vi "SubB.vi"(0 "Target B-Field":dbl=1.0 min=-4.0 max=4.0 step=0.1 format="%.4f", 3 "Custom Folder":string, 5 "optional Bias (V)":dbl=1e-08) -> ()   [LabVIEW 2013]
uses:
  <vilib>/Utility/file.llb/Write To Spreadsheet File (DBL).vi
panel:
  out "Numeric 5":dbl
  out "Difference":dbl
  out "Number of Points":dbl
  out "Time of measurement Measurement":dbl
  in  "Sweep Rate":dbl
  out "Current B-Field":dbl
  out "Numeric 4":i32
  in  "Commutator":bool
  in  "Commute SorceMeter":enum32{"Radio Selection 1", "Radio Selection 2"}(radio)
  out "Numeric 3":i32
  in  "Channel 2 (Vnano3b)":bool
  in  "Channel 1 (Vnano3)":bool
  out "Numeric":i32
  in  "Capacitance (C) and Loss (L)":bool
  in  "Magnetic Field (B)":bool
  in  "Current (Ik3)":bool
  in  "Voltage (Vk3)":bool
  in  "Current (Ik2)":bool
  in  "Voltage (Vk2)":bool
  in  "Channel 2 (Vnano2b)":bool
  in  "Channel 1 (Vnano2)":bool
  in  "Thermometer 1 (T1)":bool=TRUE
  in  "Channel 2 (Vnano1b)":bool
  in  "Channel 1 (Vnano1)":bool
  in  "Current (Ik1)":bool=TRUE
  in  "Voltage (Vk1)":bool
  out "Numeric Current":dbl
  out "Delib Time delay":i32
  in  "points at each Vg":i32=1
  out "XY Graph":cluster{dbl[], dbl[]}(graph)={[1.0, 0.8, 0.6000000000000001, 0.4000000000000001, 0.20000000000000007, 5.551115123125783e-17, -0.19999999999999996, -0.39999999999999997, -0.6, -0.8, -1.0], [0.03352775, 0.056811, 0.03911575, 0.04330675, -0.02468015, 0.011641600000000002, 0.10151450000000001, 0.12386675000000001, 0.08288825000000001, -0.00186266, -0.038650000000000004]}
  in  "Time btw \npoints, sec":dbl=1.0 format="%.2f"
  out "Array 2":dbl[][](array[numeric])
  out "array for data":dbl[](array[numeric])
  out "Numeric 2":dbl
  out "Array":string[](array[string])
  in  "Addr 1 lock-in oop":bool
  in  "Ring":u16(ring) caption="Y-axis:" items=["Vg"]
  out "String":string
  out "Data file:":path
  in  "error in (no error)":errorcluster
  in  "Ring 3":u16(ring)=1 items=["1 kOhm", "10 kOhm", "100 kOhm", "1 Mohm", "10 mOhm"]
  in  "Ring 2":u16(ring)=3 items=["1 kOhm", "10 kOhm", "100 kOhm", "1 Mohm", "10 mOhm"]
  in  "Fixed Current mkA":dbl=1.0
  in  "Current is:":T1(radio)
  in  "Ressitance measurements?":bool=TRUE
  in  "Addr 5 lock-in oop":bool
  in  "Addr 4 lock-in oop":bool
  in  "Addr 3 lock-in oop":bool
  in  "Addr 2 lock-in oop":bool
  in  "Addr 5 lock-in":bool
  in  "Addr 4 lock-in":bool
  in  "Addr 3 lock-in":bool=TRUE
  in  "Addr 2 lock-in":bool=TRUE
  in  "Addr 1 lock-in":bool=TRUE
  # "Keithley 2400: address 12"
  # "SourceMeters"
  # "Nanovoltmeters"
  # "Temperature"
  # "Main"
  # "Magnetic Field"
  # "(not recommended, too slow)"
  # "Capacitance & Loss"
  # "(not recommended, too slow)"
  # "(not recommended, too slow)"
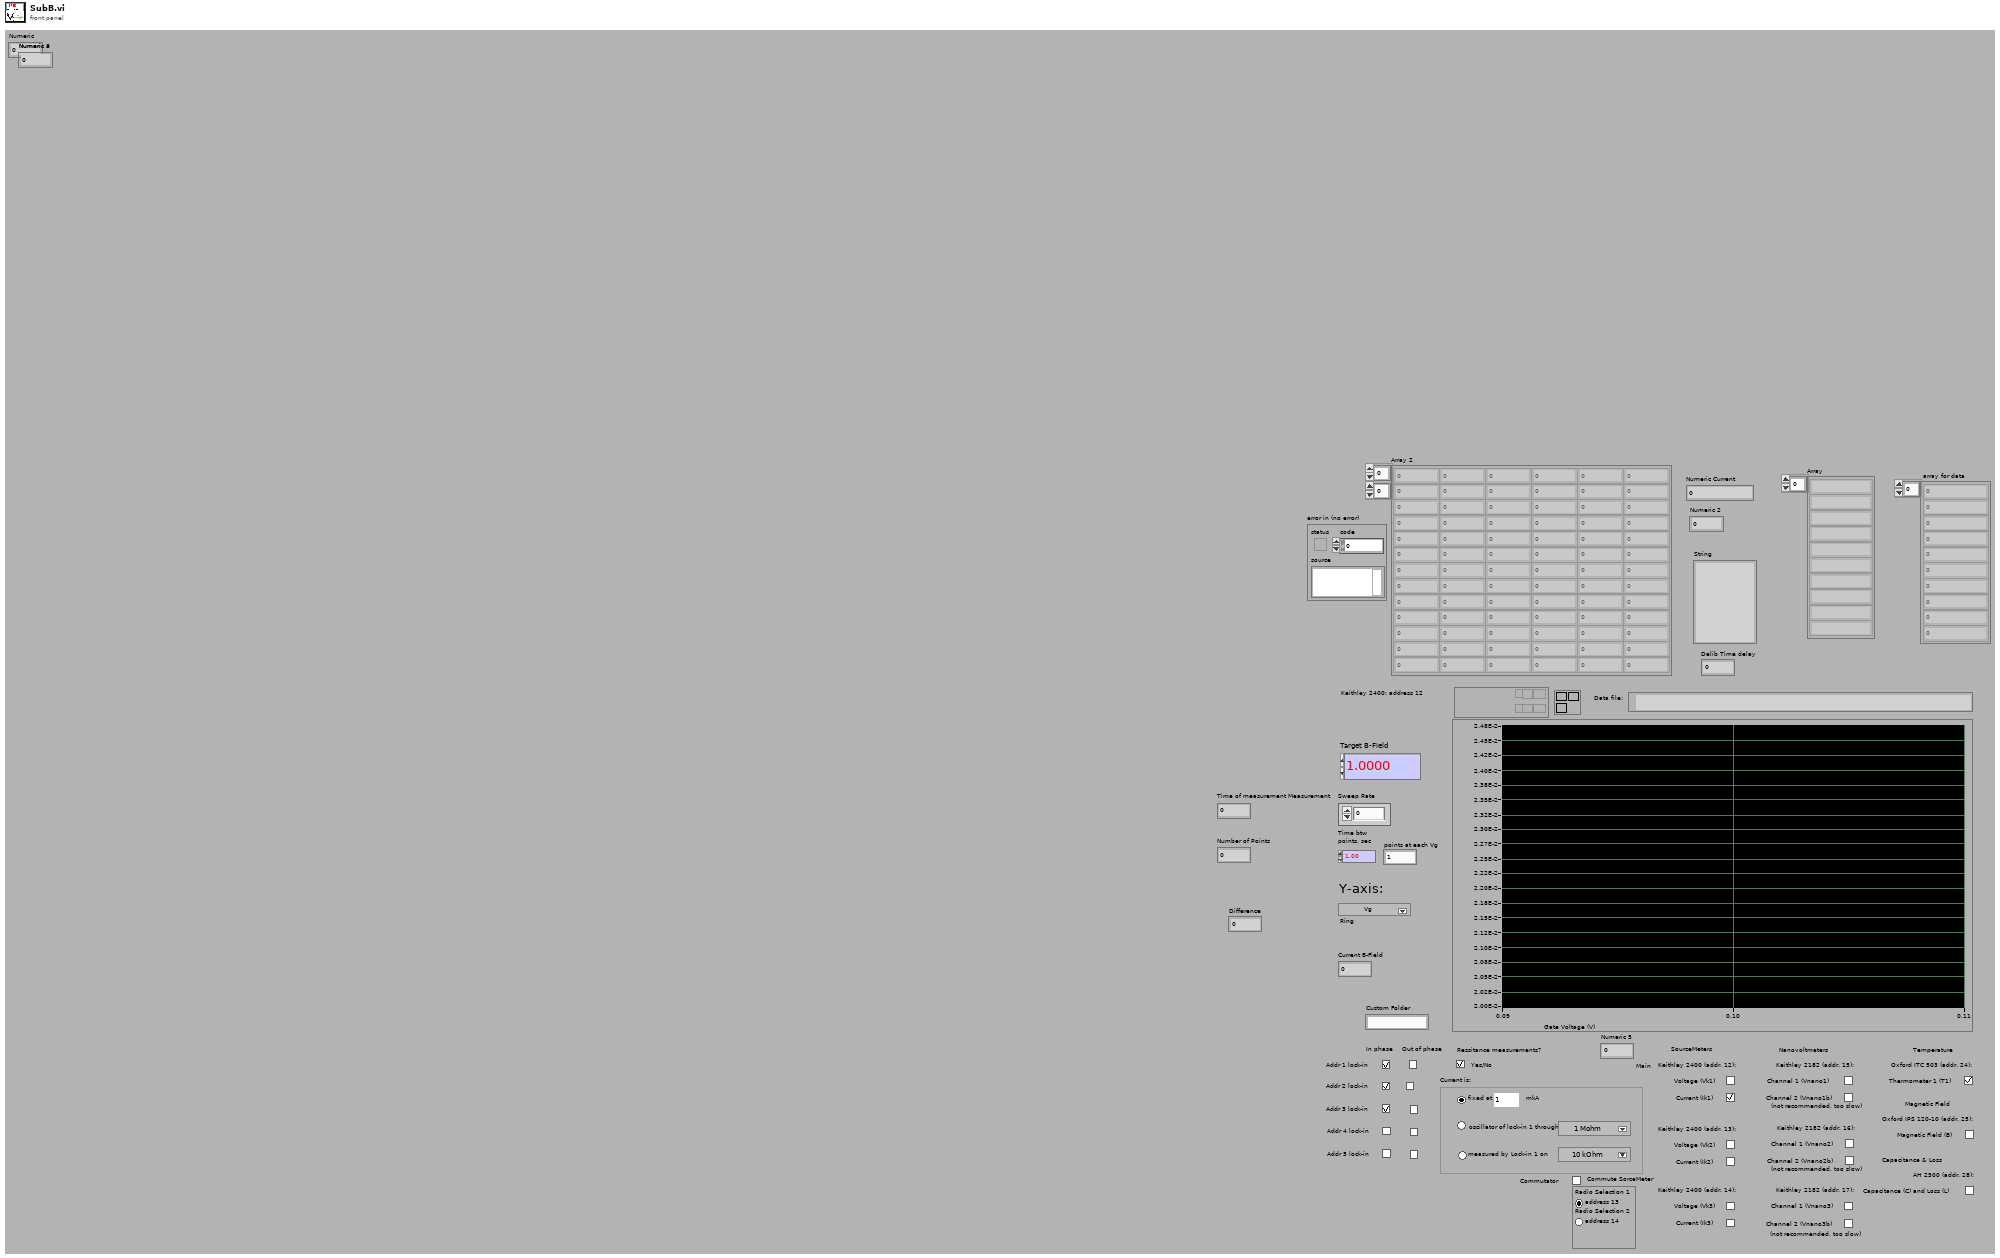
[diagram p1: front panel]
types:
  T1 = enum32{"Radio Selection 1", "Radio Selection 2", "Radio Selection 3"}
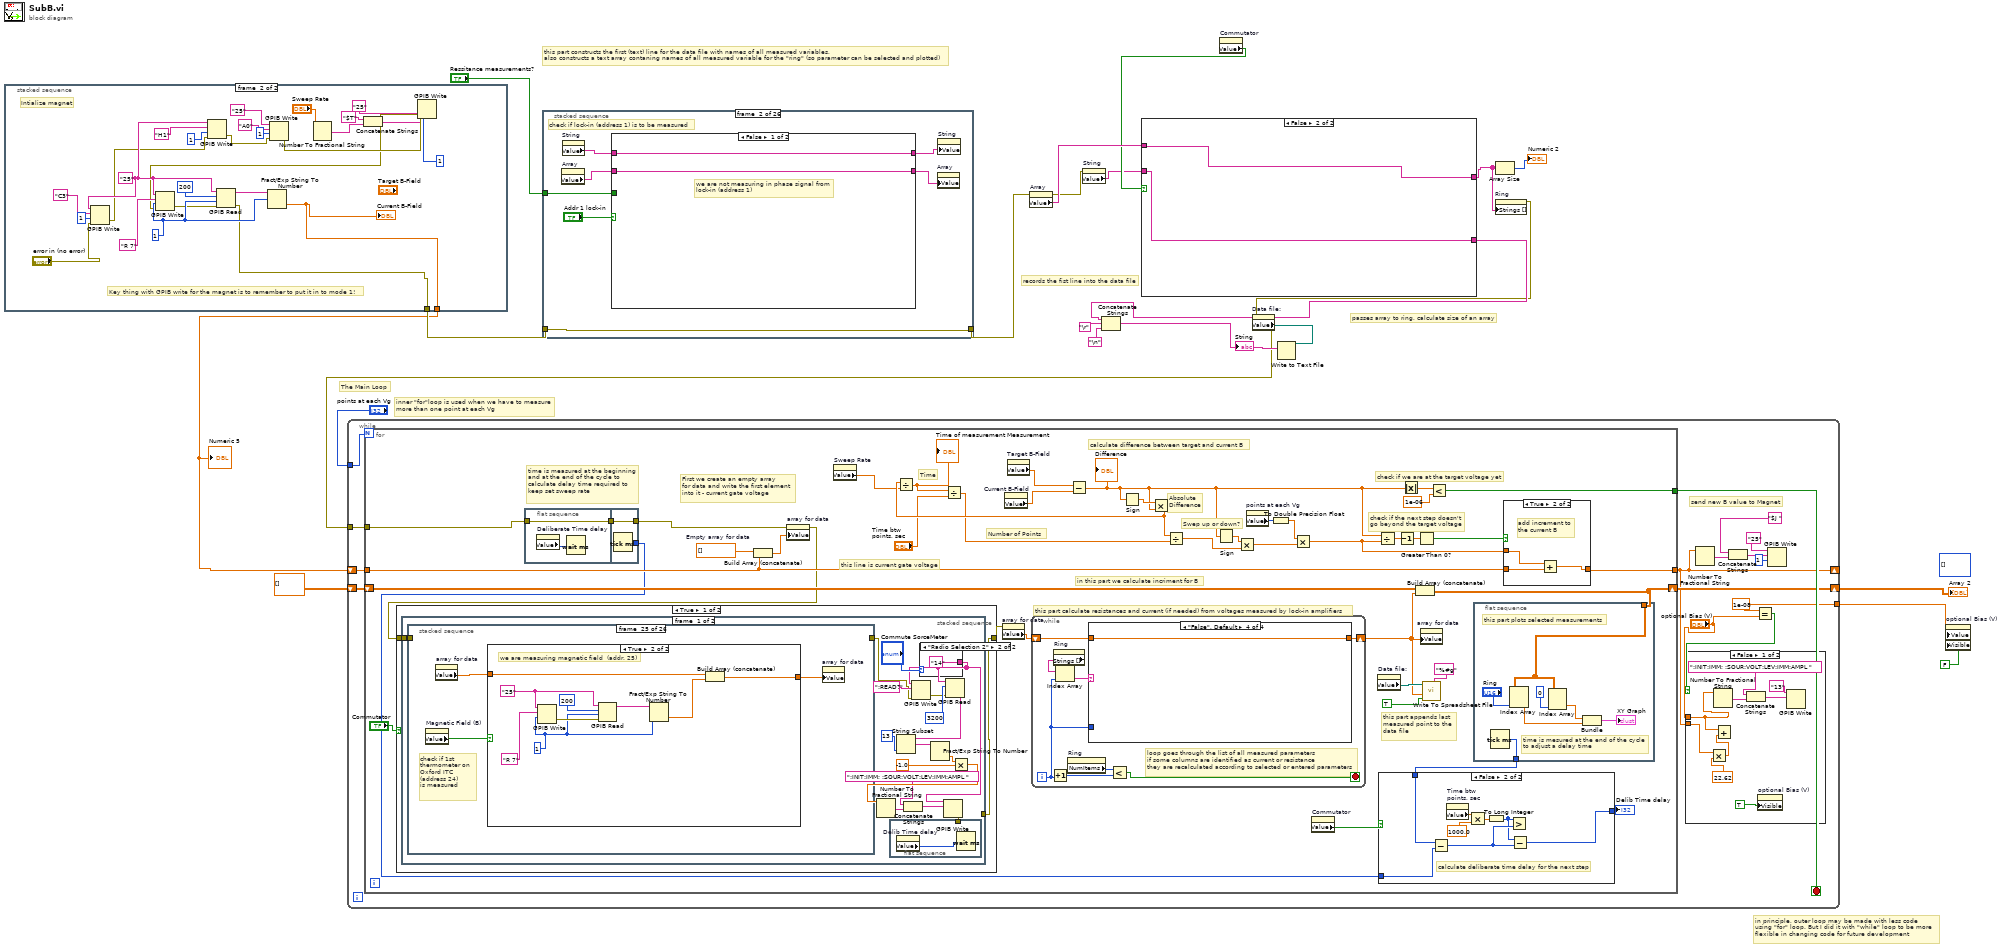
[diagram p0: block diagram]
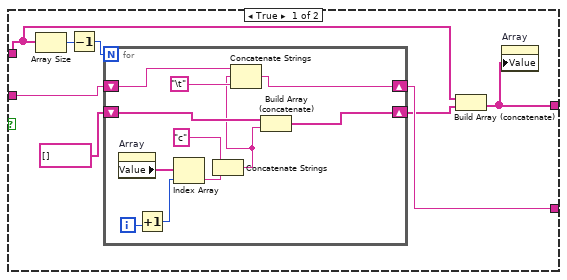
[diagram p2: hidden frame]
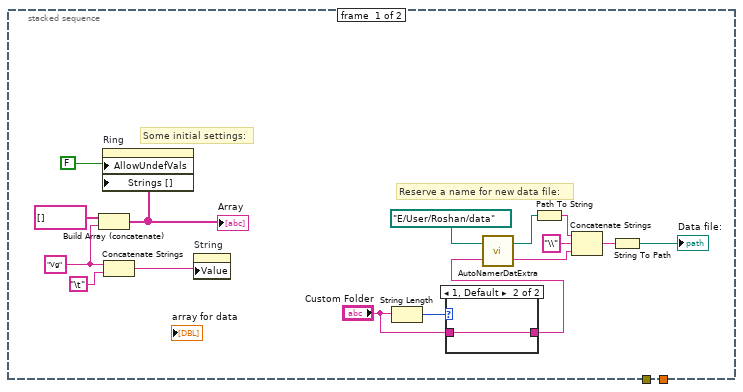
[diagram p3: hidden frame]
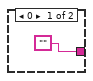
[diagram p4: hidden frame]
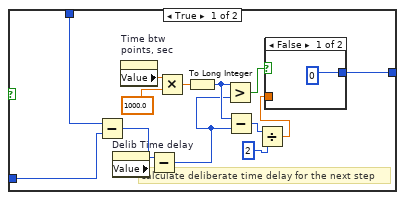
[diagram p6: hidden frame]
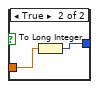
[diagram p7: hidden frame]
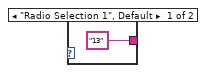
[diagram p8: hidden frame]
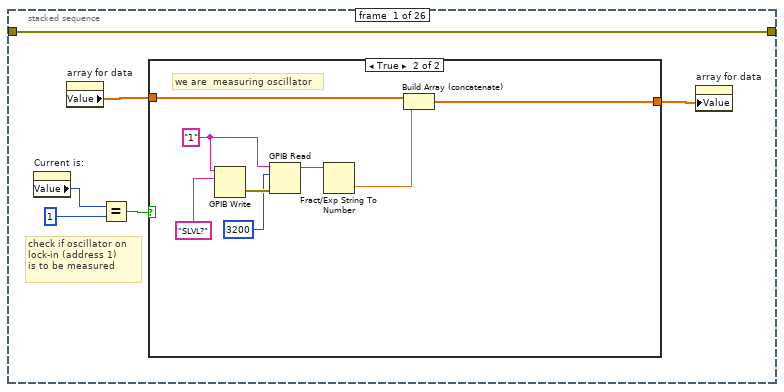
[diagram p9: hidden frame]
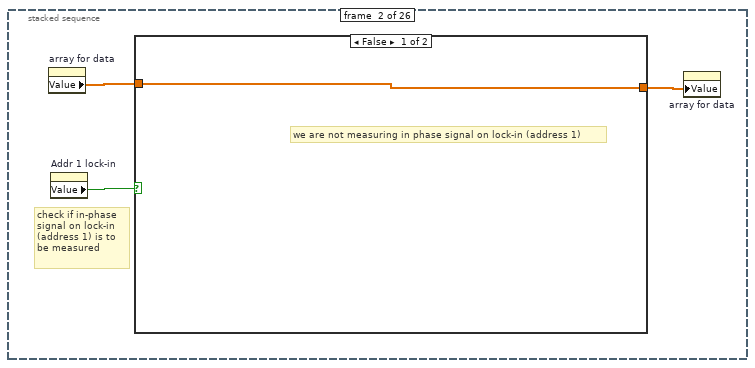
[diagram p11: hidden frame]
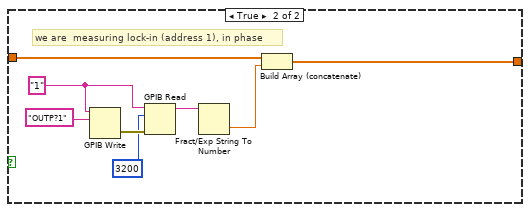
[diagram p12: hidden frame]
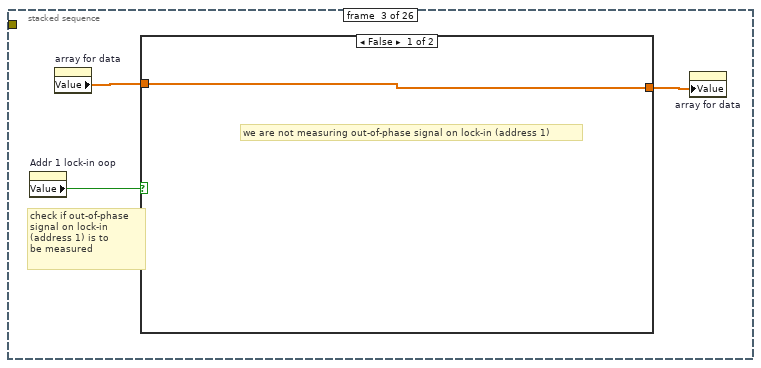
[diagram p13: hidden frame]
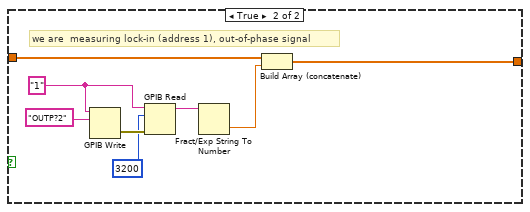
[diagram p14: hidden frame]
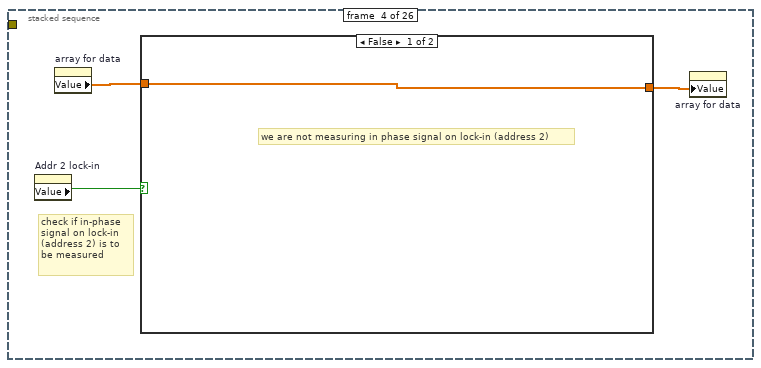
[diagram p15: hidden frame]
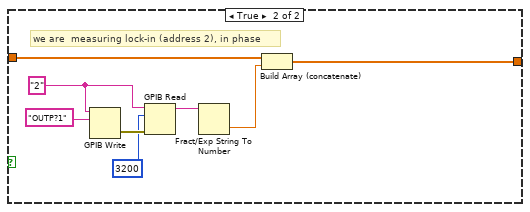
[diagram p16: hidden frame]
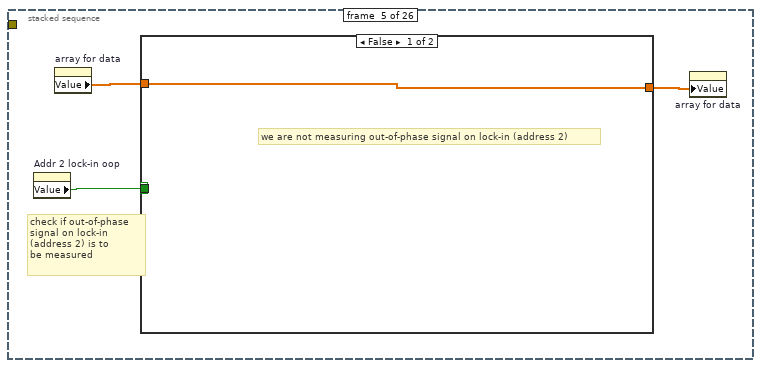
[diagram p17: hidden frame]
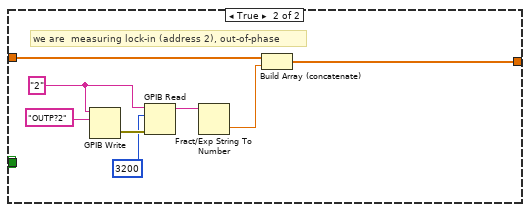
[diagram p18: hidden frame]
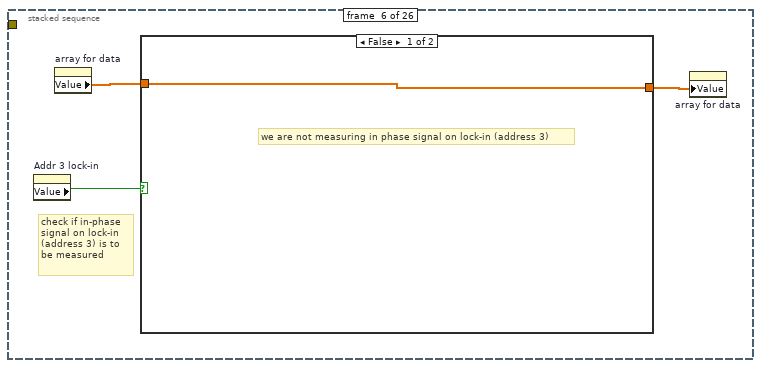
[diagram p19: hidden frame]
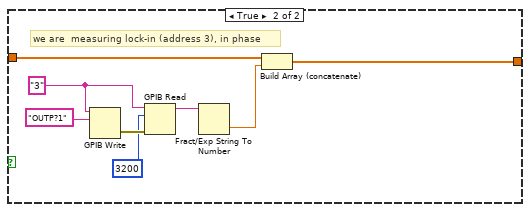
[diagram p20: hidden frame]
diagram:
  (unwired) i32[][] []
  # "passes array to ring, calculate size of an array"
  # "in principle, outer loop may be made with less code\nusing \"for\" loop. But I did it with \"while\" loop to be more \nflexible in changing code for future development"
  # "inner \"for\"loop is used when we have to measure\nmore than one point at each Vg"
  # "The Main Loop"
  # "records the fist line into the data file"
  # "this part constructs the first (text) line for the data file with names of all measured variables,\nalso constructs a text array contaning names of all measured variable for the \"ring\" (so parameter can be selected and plotted)"
  n1 = stacked-sequence {
    tunnel: [_ w61] -> w22
    tunnel: [_ w60] -> w1
    frame #0 {
      w28 = "Vg"
      # "Some initial settings:"
      # "Reserve a name for new data file:"
      n2 = Build Array (concatenate)(string[] [], w28) -> (w30:string[])
      "Array" <- w30
      n3 = property on="Ring" class="Ring (strict)"("AllowUndefVals"=FALSE, "Strings []"=w30) -> ()  [unwired: 2 in, 2 out]
      n4 = Concatenate Strings(w28, "\t") -> (w29:string)
      n5 = property on="String" class="Str"("Value"=w29) -> ()  [unwired: 2 in, 2 out]
      n6 = String Length(string="Custom Folder") -> (length=w25:i32)
      n7 = case shown="1, Default" w25 {
        tunnel: "Custom Folder" -> [_ w40]
        tunnel: ["" w40] -> w23
        frame 0 {
        }
        frame 1, Default {
        }
      }
      n8 = call "AutoNamerDatExtra.vi"("ExtraString"=w23, "Custom User Path"=path "E:/User/Roshan/data") -> ("String"=w38:string, "Path"=w37:path)
      n9 = Path To String(path=w37) -> (string=w32:string)
      n10 = Concatenate Strings(w32, "\\", w38) -> (w34:string)
      n11 = String To Path(string=w34) -> (path=→"Data file:":path)
    }
    frame #1 {
      w66 = 1
      w56 = "25"
      # "Key thing with GPIB write for the magnet is to remember to put it in to mode 1!"
      # "Intialize magnet"
      n12 = GPIB Write(0:w56, 1:"C3" ("data"), 2:i16 1 ("mode (0)"), 3:"error in (no error)") -> (6:w53:errorcluster)  [unwired: 1 in, 1 out]
      n13 = GPIB Write(0:w56, 1:"H1" ("data"), 2:i16 1 ("mode (0)"), 3:w53) -> (6:w49:errorcluster)  [unwired: 1 in, 1 out]
      n14 = GPIB Write(0:"25" ("address string"), 1:"A0" ("data"), 2:i16 1 ("mode (0)"), 3:w49) -> (6:w48:errorcluster)  [unwired: 1 in, 1 out]
      n15 = Number To Fractional String(number="Sweep Rate") -> (F-format string=w44:string)  [unwired: 3 in]
      n16 = Concatenate Strings("$T" ("string"), w44) -> (w42:string)
      n17 = GPIB Write(0:"25" ("address string"), 1:w42, 2:i16 1 ("mode (0)"), 3:w48) -> (6:w47:errorcluster)  [unwired: 1 in, 1 out]
      n18 = GPIB Write(0:w56, 1:"R 7", 2:w66, 3:w47) -> (6:w62:errorcluster)  [unwired: 1 in, 1 out]
      n19 = GPIB Read(0:w56, 1:200, 2:w66, 3:w62) -> (5:w65:string, 7:w61:errorcluster)  [unwired: 1 in, 1 out]
      n20 = Fract/Exp String To Number(string=w65, offset=w66) -> (number=w60:dbl)  [unwired: 2 in, 1 out]
      "Current B-Field" <- w60
    }
  }
  "Numeric 5" <- w1
  n21 = stacked-sequence {
    tunnel: "Ressitance measurements?" -> [w74 w89 w113 w136 w154 w172 w190 w208 w226 w244 w262 _ _ _ _ _ _ _ _ _ _ _ _ _ _ _]
    tunnel: w22 -> [_ w86 _ _ _ _ _ _ _ _ _ _ _ _ _ _ _ _ _ _ _ _ _ _ _ _]
    tunnel: [_ w86 _ _ _ _ _ _ _ _ _ _ _ _ _ _ _ _ _ _ _ _ _ _ _ _] -> w19
    frame #0 {
      # "check if oscillator of  lock-in (address 1) is to be measured"
      n22 = property on="Array" class="Arr (strict)"() -> ("Value"=w69:string[])  [unwired: 2 in, 2 out]
      n23 = property on="String" class="Str"() -> ("Value"=w73:string)  [unwired: 2 in, 2 out]
      n24 = Equal?(x="Current is:", y=1) -> (x = y?=w70:bool)
      n25 = case shown="False" w70 {
        tunnel: w74 -> [_ _]
        tunnel: [w76 w77] -> w72
        tunnel: w73 -> [w76 w80]
        tunnel: w69 -> [w75 w79]
        tunnel: [w75 w78] -> w68
        frame False {
          # "we are not measuring oscillator from\nlock-in (address 1)"
        }
        frame True {
          w81 = "I"
          # "we are  measuring oscillator"
          n26 = GPIB Clear(3:"1") -> ()  [unwired: 1 in, 2 out]
          n27 = Concatenate Strings(w80, w81, "\t") -> (w77:string)
          n28 = Build Array (concatenate)(w79, w81) -> (w78:string[])
        }
      }
      n29 = property on="Array" class="Arr (strict)"("Value"=w68) -> ()  [unwired: 2 in, 2 out]
      n30 = property on="String" class="Str"("Value"=w72) -> ()  [unwired: 2 in, 2 out]
    }
    frame #1 {
      # "check if lock-in (address 1) is to be measured"
      n31 = property on="Array" class="Arr (strict)"() -> ("Value"=w85:string[])  [unwired: 2 in, 2 out]
      n32 = property on="String" class="Str"() -> ("Value"=w88:string)  [unwired: 2 in, 2 out]
      n33 = case shown="False" "Addr 1 lock-in" {
        tunnel: w89 -> [_ w100]
        tunnel: [w92 w96] -> w87
        tunnel: w88 -> [w92 w95]
        tunnel: w85 -> [w91 w97]
        tunnel: [w91 w98] -> w84
        frame False {
          # "we are not measuring in phase signal from\nlock-in (address 1)"
        }
        frame True {
          # "are we measuring resistance?"
          n34 = GPIB Clear(3:"1") -> ()  [unwired: 1 in, 2 out]
          n35 = case shown="True" w100 {
            tunnel: ["V1" w102] -> w93
            frame False {
              # "no, we are not measuring resistanse;\nall lock-ins are measuring voltage"
            }
            frame True {
              # "are we measuring current as well?"
              n36 = property on="Current is:" class="RadioBtnsControl (strict)"() -> ("Value"=w104:T1)  [unwired: 2 in, 2 out]
              n37 = Equal?(x=w104, y=2) -> (x = y?=w105:bool)
              n38 = case shown="False" w105 {
                tunnel: ["R1" "I"] -> w102
                frame False {
                  # "no, we are not \nmeasuring current\nby lock-in \n(address 1); \nso this lock-in is \nmeasuring resistance"
                }
                frame True {
                  # "yes, we are measuring \ncurrent by lock-in \n(address 1) as \nvoltage drop on \nknown resistance"
                }
              }
            }
          }
          n39 = Concatenate Strings(w95, w93, "\t") -> (w96:string)
          n40 = Build Array (concatenate)(w97, w93) -> (w98:string[])
        }
      }
      n41 = property on="Array" class="Arr (strict)"("Value"=w84) -> ()  [unwired: 2 in, 2 out]
      n42 = property on="String" class="Str"("Value"=w87) -> ()  [unwired: 2 in, 2 out]
    }
    frame #2 {
      # "check if out-of-phase signal on  lock-in (address 1) is to be measured"
      n43 = property on="Array" class="Arr (strict)"() -> ("Value"=w110:string[])  [unwired: 2 in, 2 out]
      n44 = property on="String" class="Str"() -> ("Value"=w112:string)  [unwired: 2 in, 2 out]
      n45 = case shown="False" "Addr 1 lock-in oop" {
        tunnel: w113 -> [_ w123]
        tunnel: [w115 w119] -> w111
        tunnel: w112 -> [w115 w118]
        tunnel: w110 -> [w114 w120]
        tunnel: [w114 w121] -> w109
        frame False {
          # "we are not measuring iout-of-phase signal from\nlock-in (address 1)"
        }
        frame True {
          # "are we measuring resistance?"
          n46 = GPIB Clear(3:"1") -> ()  [unwired: 1 in, 2 out]
          n47 = case shown="True" w123 {
            tunnel: ["V1oop" w125] -> w116
            frame False {
              # "no, we are not measuring resistance;\nall lock-ins are measuring voltage"
            }
            frame True {
              # "are we measuring out-of-phase current as well?"
              n48 = property on="Current is:" class="RadioBtnsControl (strict)"() -> ("Value"=w127:T1)  [unwired: 2 in, 2 out]
              n49 = Equal?(x=w127, y=2) -> (x = y?=w128:bool)
              n50 = case shown="False" w128 {
                tunnel: ["R1oop" "Ioop"] -> w125
                frame False {
                  # "no, we are not \nmeasuring current\nby lock-in \n(address 1); so this \nlock-in is measuring\nout-of-phase resistance"
                }
                frame True {
                  # "yes, we are measuring \nout-of phase current \nby lock-in (address 1) \nas voltage drop on \nknown resistance"
                }
              }
            }
          }
          n51 = Concatenate Strings(w118, w116, "\t") -> (w119:string)
          n52 = Build Array (concatenate)(w120, w116) -> (w121:string[])
        }
      }
      n53 = property on="Array" class="Arr (strict)"("Value"=w109) -> ()  [unwired: 2 in, 2 out]
      n54 = property on="String" class="Str"("Value"=w111) -> ()  [unwired: 2 in, 2 out]
    }
    frame #3 {
      # "check if in-phase signal on  lock-in (address 2) is to be measured"
      n55 = property on="Array" class="Arr (strict)"() -> ("Value"=w133:string[])  [unwired: 2 in, 2 out]
      n56 = property on="String" class="Str"() -> ("Value"=w135:string)  [unwired: 2 in, 2 out]
      n57 = case shown="False" "Addr 2 lock-in" {
        tunnel: w136 -> [_ w146]
        tunnel: [w138 w142] -> w134
        tunnel: w135 -> [w138 w141]
        tunnel: w133 -> [w137 w143]
        tunnel: [w137 w144] -> w132
        frame False {
          # "we are not measuring in-phase signal from\nlock-in (address 2)"
        }
        frame True {
          # "are we measuring resistance?"
          n58 = GPIB Clear(3:"2") -> ()  [unwired: 1 in, 2 out]
          n59 = case shown="True" w146 {
            tunnel: ["R2" "V2"] -> w139
            frame True {
              # "we are measuring \nresistance by lock-in \n(address 2)"
            }
            frame False, Default {
              # "no, we are not measuring resistance;\nall lock-ins are measuring voltage"
            }
          }
          n60 = Concatenate Strings(w141, w139, "\t") -> (w142:string)
          n61 = Build Array (concatenate)(w143, w139) -> (w144:string[])
        }
      }
      n62 = property on="Array" class="Arr (strict)"("Value"=w132) -> ()  [unwired: 2 in, 2 out]
      n63 = property on="String" class="Str"("Value"=w134) -> ()  [unwired: 2 in, 2 out]
    }
    frame #4 {
      # "check if out-of-phase signal on  lock-in (address 2) is to be measured"
      n64 = property on="Array" class="Arr (strict)"() -> ("Value"=w151:string[])  [unwired: 2 in, 2 out]
      n65 = property on="String" class="Str"() -> ("Value"=w153:string)  [unwired: 2 in, 2 out]
      n66 = case shown="False" "Addr 2 lock-in oop" {
        tunnel: w154 -> [_ w164]
        tunnel: [w156 w160] -> w152
        tunnel: w153 -> [w156 w159]
        tunnel: w151 -> [w155 w161]
        tunnel: [w155 w162] -> w150
        frame False {
          # "we are not measuring out-of-phase signal from\nlock-in (address 2)"
        }
        frame True {
          # "are we measuring resistance?"
          n67 = GPIB Clear(3:"2") -> ()  [unwired: 1 in, 2 out]
          n68 = case shown="True" w164 {
            tunnel: ["R2oop" "V2oop"] -> w157
            frame True {
              # "we are measuring out-of-phase resistance by lock-in (address 2)\n(address 2)"
            }
            frame False, Default {
              # "no, we are not measuring resistance;\nall lock-ins are measuring voltage"
            }
          }
          n69 = Concatenate Strings(w159, w157, "\t") -> (w160:string)
          n70 = Build Array (concatenate)(w161, w157) -> (w162:string[])
        }
      }
      n71 = property on="Array" class="Arr (strict)"("Value"=w150) -> ()  [unwired: 2 in, 2 out]
      n72 = property on="String" class="Str"("Value"=w152) -> ()  [unwired: 2 in, 2 out]
    }
    frame #5 {
      # "check if in-phase signal on  lock-in (address 3) is to be measured"
      n73 = property on="Array" class="Arr (strict)"() -> ("Value"=w169:string[])  [unwired: 2 in, 2 out]
      n74 = property on="String" class="Str"() -> ("Value"=w171:string)  [unwired: 2 in, 2 out]
      n75 = case shown="False" "Addr 3 lock-in" {
        tunnel: w172 -> [_ w182]
        tunnel: [w174 w178] -> w170
        tunnel: w171 -> [w174 w177]
        tunnel: w169 -> [w173 w179]
        tunnel: [w173 w180] -> w168
        frame False {
          # "we are not measuring in-phase signal from\nlock-in (address 3)"
        }
        frame True {
          # "are we measuring resistance?"
          n76 = GPIB Clear(3:"3") -> ()  [unwired: 1 in, 2 out]
          n77 = case shown="True" w182 {
            tunnel: ["R3" "V3"] -> w175
            frame True {
              # "we are measuring \nresistance by lock-in \n(address 3)"
            }
            frame False, Default {
              # "no, we are not measuring resistance;\nall lock-ins are measuring voltage"
            }
          }
          n78 = Concatenate Strings(w177, w175, "\t") -> (w178:string)
          n79 = Build Array (concatenate)(w179, w175) -> (w180:string[])
        }
      }
      n80 = property on="Array" class="Arr (strict)"("Value"=w168) -> ()  [unwired: 2 in, 2 out]
      n81 = property on="String" class="Str"("Value"=w170) -> ()  [unwired: 2 in, 2 out]
    }
    frame #6 {
      # "check if out-of-phase signal on  lock-in (address 3) is to be measured"
      n82 = property on="Array" class="Arr (strict)"() -> ("Value"=w187:string[])  [unwired: 2 in, 2 out]
      n83 = property on="String" class="Str"() -> ("Value"=w189:string)  [unwired: 2 in, 2 out]
      n84 = case shown="False" "Addr 3 lock-in oop" {
        tunnel: w190 -> [_ w200]
        tunnel: [w192 w196] -> w188
        tunnel: w189 -> [w192 w195]
        tunnel: w187 -> [w191 w197]
        tunnel: [w191 w198] -> w186
        frame False {
          # "we are not measuring out-of-phase signal from\nlock-in (address 3)"
        }
        frame True {
          # "are we measuring resistance?"
          n85 = GPIB Clear(3:"3") -> ()  [unwired: 1 in, 2 out]
          n86 = case shown="True" w200 {
            tunnel: ["R3oop" "V3oop"] -> w193
            frame True {
              # "we are measuring out-of-phase resistance by lock-in (address 3)\n(address 2)"
            }
            frame False, Default {
              # "no, we are not measuring resistance;\nall lock-ins are measuring voltage"
            }
          }
          n87 = Concatenate Strings(w195, w193, "\t") -> (w196:string)
          n88 = Build Array (concatenate)(w197, w193) -> (w198:string[])
        }
      }
      n89 = property on="Array" class="Arr (strict)"("Value"=w186) -> ()  [unwired: 2 in, 2 out]
      n90 = property on="String" class="Str"("Value"=w188) -> ()  [unwired: 2 in, 2 out]
    }
    frame #7 {
      # "check if in-phase signal on  lock-in (address 4) is to be measured"
      n91 = property on="Array" class="Arr (strict)"() -> ("Value"=w205:string[])  [unwired: 2 in, 2 out]
      n92 = property on="String" class="Str"() -> ("Value"=w207:string)  [unwired: 2 in, 2 out]
      n93 = case shown="False" "Addr 4 lock-in" {
        tunnel: w208 -> [_ w218]
        tunnel: [w210 w214] -> w206
        tunnel: w207 -> [w210 w213]
        tunnel: w205 -> [w209 w215]
        tunnel: [w209 w216] -> w204
        frame False {
          # "we are not measuring in-phase signal from\nlock-in (address 4)"
        }
        frame True {
          # "are we measuring resistance?"
          n94 = GPIB Clear(3:"4") -> ()  [unwired: 1 in, 2 out]
          n95 = case shown="True" w218 {
            tunnel: ["R4" "V4"] -> w211
            frame True {
              # "we are measuring \nresistance by lock-in \n(address 4)"
            }
            frame False, Default {
              # "no, we are not measuring resistance;\nall lock-ins are measuring voltage"
            }
          }
          n96 = Concatenate Strings(w213, w211, "\t") -> (w214:string)
          n97 = Build Array (concatenate)(w215, w211) -> (w216:string[])
        }
      }
      n98 = property on="Array" class="Arr (strict)"("Value"=w204) -> ()  [unwired: 2 in, 2 out]
      n99 = property on="String" class="Str"("Value"=w206) -> ()  [unwired: 2 in, 2 out]
    }
    frame #8 {
      # "check if out-of-phase signal on  lock-in (address 4) is to be measured"
      n100 = property on="Array" class="Arr (strict)"() -> ("Value"=w223:string[])  [unwired: 2 in, 2 out]
      n101 = property on="String" class="Str"() -> ("Value"=w225:string)  [unwired: 2 in, 2 out]
      n102 = case shown="False" "Addr 4 lock-in oop" {
        tunnel: w226 -> [_ w236]
        tunnel: [w228 w232] -> w224
        tunnel: w225 -> [w228 w231]
        tunnel: w223 -> [w227 w233]
        tunnel: [w227 w234] -> w222
        frame False {
          # "we are not measuring out-of-phase signal from\nlock-in (address 4)"
        }
        frame True {
          # "are we measuring resistance?"
          n103 = GPIB Clear(3:"4") -> ()  [unwired: 1 in, 2 out]
          n104 = case shown="True" w236 {
            tunnel: ["R4oop" "V4oop"] -> w229
            frame True {
              # "we are measuring out-of-phase resistance by lock-in (address 4)\n(address 2)"
            }
            frame False, Default {
              # "no, we are not measuring resistance;\nall lock-ins are measuring voltage"
            }
          }
          n105 = Concatenate Strings(w231, w229, "\t") -> (w232:string)
          n106 = Build Array (concatenate)(w233, w229) -> (w234:string[])
        }
      }
      n107 = property on="Array" class="Arr (strict)"("Value"=w222) -> ()  [unwired: 2 in, 2 out]
      n108 = property on="String" class="Str"("Value"=w224) -> ()  [unwired: 2 in, 2 out]
    }
    frame #9 {
      # "check if in-phase signal on  lock-in (address 5) is to be measured"
      n109 = property on="Array" class="Arr (strict)"() -> ("Value"=w241:string[])  [unwired: 2 in, 2 out]
      n110 = property on="String" class="Str"() -> ("Value"=w243:string)  [unwired: 2 in, 2 out]
      n111 = case shown="False" "Addr 5 lock-in" {
        tunnel: w244 -> [_ w254]
        tunnel: [w246 w250] -> w242
        tunnel: w243 -> [w246 w249]
        tunnel: w241 -> [w245 w251]
        tunnel: [w245 w252] -> w240
        frame False {
          # "we are not measuring in-phase signal from\nlock-in (address 5)"
        }
        frame True {
          # "are we measuring resistance?"
          n112 = GPIB Clear(3:"5") -> ()  [unwired: 1 in, 2 out]
          n113 = case shown="True" w254 {
            tunnel: ["R5" "V5"] -> w247
            frame True {
              # "we are measuring \nresistance by lock-in \n(address 5)"
            }
            frame False, Default {
              # "no, we are not measuring resistance;\nall lock-ins are measuring voltage"
            }
          }
          n114 = Concatenate Strings(w249, w247, "\t") -> (w250:string)
          n115 = Build Array (concatenate)(w251, w247) -> (w252:string[])
        }
      }
      n116 = property on="Array" class="Arr (strict)"("Value"=w240) -> ()  [unwired: 2 in, 2 out]
      n117 = property on="String" class="Str"("Value"=w242) -> ()  [unwired: 2 in, 2 out]
    }
    frame #10 {
      # "check if out-of-phase signal on  lock-in (address 5) is to be measured"
      n118 = property on="Array" class="Arr (strict)"() -> ("Value"=w259:string[])  [unwired: 2 in, 2 out]
      n119 = property on="String" class="Str"() -> ("Value"=w261:string)  [unwired: 2 in, 2 out]
      n120 = case shown="False" "Addr 5 lock-in oop" {
        tunnel: w262 -> [_ w272]
        tunnel: [w264 w268] -> w260
        tunnel: w261 -> [w264 w267]
        tunnel: w259 -> [w263 w269]
        tunnel: [w263 w270] -> w258
        frame False {
          # "we are not measuring out-of-phase signal from\nlock-in (address 5)"
        }
        frame True {
          # "are we measuring resistance?"
          n121 = GPIB Clear(3:"5") -> ()  [unwired: 1 in, 2 out]
          n122 = case shown="True" w272 {
            tunnel: ["R5oop" "V5oop"] -> w265
            frame True {
              # "we are measuring out-of-phase resistance by lock-in (address 5)\n(address 2)"
            }
            frame False, Default {
              # "no, we are not measuring resistance;\nall lock-ins are measuring voltage"
            }
          }
          n123 = Concatenate Strings(w267, w265, "\t") -> (w268:string)
          n124 = Build Array (concatenate)(w269, w265) -> (w270:string[])
        }
      }
      n125 = property on="Array" class="Arr (strict)"("Value"=w258) -> ()  [unwired: 2 in, 2 out]
      n126 = property on="String" class="Str"("Value"=w260) -> ()  [unwired: 2 in, 2 out]
    }
    frame #11 {
      # "check if voltage on main Keithley 2400 (addr. 12) is measured"
      n127 = property on="Array" class="Arr (strict)"() -> ("Value"=w277:string[])  [unwired: 2 in, 2 out]
      n128 = property on="String" class="Str"() -> ("Value"=w279:string)  [unwired: 2 in, 2 out]
      n129 = case shown="False" "Voltage (Vk1)" {
        tunnel: [w281 w285] -> w278
        tunnel: w279 -> [w281 w284]
        tunnel: w277 -> [w280 w286]
        tunnel: [w280 w287] -> w276
        frame False {
          # "no , we aren't measuring voltage \non main Keithley 2400 (addr. 12)"
        }
        frame True {
          w282 = "Vk1"
          # "yes , we are measuring voltage \non main Keithley 2400 (addr. 12)"
          n130 = GPIB Clear(3:"12") -> ()  [unwired: 1 in, 2 out]
          n131 = Concatenate Strings(w284, w282, "\t") -> (w285:string)
          n132 = Build Array (concatenate)(w286, w282) -> (w287:string[])
        }
      }
      n133 = property on="String" class="Str"("Value"=w278) -> ()  [unwired: 2 in, 2 out]
      n134 = property on="Array" class="Arr (strict)"("Value"=w276) -> ()  [unwired: 2 in, 2 out]
    }
    frame #12 {
      # "check if current on main Keithley 2400 (addr. 12) is measured"
      n135 = property on="Array" class="Arr (strict)"() -> ("Value"=w291:string[])  [unwired: 2 in, 2 out]
      n136 = property on="String" class="Str"() -> ("Value"=w293:string)  [unwired: 2 in, 2 out]
      n137 = case shown="True" "Current (Ik1)" {
        tunnel: [w295 w299] -> w292
        tunnel: w293 -> [w295 w298]
        tunnel: w291 -> [w294 w300]
        tunnel: [w294 w301] -> w290
        frame False {
          # "no , we aren't measuring current\non main Keithley 2400 (addr. 12)"
        }
        frame True {
          w296 = "Ik1"
          # "yes , we are measuring current \non main Keithley 2400 (addr. 12)"
          n138 = GPIB Clear(3:"12") -> ()  [unwired: 1 in, 2 out]
          n139 = Concatenate Strings(w298, w296, "\t") -> (w299:string)
          n140 = Build Array (concatenate)(w300, w296) -> (w301:string[])
        }
      }
      n141 = property on="String" class="Str"("Value"=w292) -> ()  [unwired: 2 in, 2 out]
      n142 = property on="Array" class="Arr (strict)"("Value"=w290) -> ()  [unwired: 2 in, 2 out]
    }
    frame #13 {
      # "check if voltage on additional Keithley 2400 (addr. 13) is measured"
      n143 = property on="Array" class="Arr (strict)"() -> ("Value"=w305:string[])  [unwired: 2 in, 2 out]
      n144 = property on="String" class="Str"() -> ("Value"=w307:string)  [unwired: 2 in, 2 out]
      n145 = case shown="False" "Voltage (Vk2)" {
        tunnel: [w309 w313] -> w306
        tunnel: w307 -> [w309 w312]
        tunnel: w305 -> [w308 w314]
        tunnel: [w308 w315] -> w304
        frame False {
          # "no , we aren't measuring voltage \non Keithley 2400 (addr. 13)"
        }
        frame True {
          w310 = "Vk2"
          # "yes , we are measuring voltage \non Keithley 2400 (addr. 13)"
          n146 = GPIB Clear(3:"13") -> ()  [unwired: 1 in, 2 out]
          n147 = Concatenate Strings(w312, w310, "\t") -> (w313:string)
          n148 = Build Array (concatenate)(w314, w310) -> (w315:string[])
        }
      }
      n149 = property on="String" class="Str"("Value"=w306) -> ()  [unwired: 2 in, 2 out]
      n150 = property on="Array" class="Arr (strict)"("Value"=w304) -> ()  [unwired: 2 in, 2 out]
    }
    frame #14 {
      # "check if current on additional Keithley 2400 (addr. 13) is measured"
      n151 = property on="Array" class="Arr (strict)"() -> ("Value"=w319:string[])  [unwired: 2 in, 2 out]
      n152 = property on="String" class="Str"() -> ("Value"=w321:string)  [unwired: 2 in, 2 out]
      n153 = case shown="False" "Current (Ik2)" {
        tunnel: [w323 w327] -> w320
        tunnel: w321 -> [w323 w326]
        tunnel: w319 -> [w322 w328]
        tunnel: [w322 w329] -> w318
        frame False {
          # "no , we aren't measuring current\non Keithley 2400 (addr. 13)"
        }
        frame True {
          w324 = "Ik2"
          # "yes , we are measuring current \non Keithley 2400 (addr. 13)"
          n154 = GPIB Clear(3:"13") -> ()  [unwired: 1 in, 2 out]
          n155 = Concatenate Strings(w326, w324, "\t") -> (w327:string)
          n156 = Build Array (concatenate)(w328, w324) -> (w329:string[])
        }
      }
      n157 = property on="String" class="Str"("Value"=w320) -> ()  [unwired: 2 in, 2 out]
      n158 = property on="Array" class="Arr (strict)"("Value"=w318) -> ()  [unwired: 2 in, 2 out]
    }
    frame #15 {
      # "check if voltage on additional Keithley 2400 (addr. 14) is measured"
      n159 = property on="Array" class="Arr (strict)"() -> ("Value"=w333:string[])  [unwired: 2 in, 2 out]
      n160 = property on="String" class="Str"() -> ("Value"=w335:string)  [unwired: 2 in, 2 out]
      n161 = case shown="False" "Voltage (Vk3)" {
        tunnel: [w337 w341] -> w334
        tunnel: w335 -> [w337 w340]
        tunnel: w333 -> [w336 w342]
        tunnel: [w336 w343] -> w332
        frame False {
          # "no , we aren't measuring voltage \non Keithley 2400 (addr. 14)"
        }
        frame True {
          w338 = "Vk3"
          # "yes , we are measuring voltage \non Keithley 2400 (addr. 14)"
          n162 = GPIB Clear(3:"14") -> ()  [unwired: 1 in, 2 out]
          n163 = Concatenate Strings(w340, w338, "\t") -> (w341:string)
          n164 = Build Array (concatenate)(w342, w338) -> (w343:string[])
        }
      }
      n165 = property on="String" class="Str"("Value"=w334) -> ()  [unwired: 2 in, 2 out]
      n166 = property on="Array" class="Arr (strict)"("Value"=w332) -> ()  [unwired: 2 in, 2 out]
    }
    frame #16 {
      # "check if current on additional Keithley 2400 (addr. 14) is measured"
      n167 = property on="Array" class="Arr (strict)"() -> ("Value"=w347:string[])  [unwired: 2 in, 2 out]
      n168 = property on="String" class="Str"() -> ("Value"=w349:string)  [unwired: 2 in, 2 out]
      n169 = case shown="False" "Current (Ik3)" {
        tunnel: [w351 w355] -> w348
        tunnel: w349 -> [w351 w354]
        tunnel: w347 -> [w350 w356]
        tunnel: [w350 w357] -> w346
        frame False {
          # "no , we aren't measuring current\non Keithley 2400 (addr. 14)"
        }
        frame True {
          w352 = "Ik3"
          # "yes , we are measuring current \non Keithley 2400 (addr. 14)"
          n170 = GPIB Clear(3:"14") -> ()  [unwired: 1 in, 2 out]
          n171 = Concatenate Strings(w354, w352, "\t") -> (w355:string)
          n172 = Build Array (concatenate)(w356, w352) -> (w357:string[])
        }
      }
      n173 = property on="String" class="Str"("Value"=w348) -> ()  [unwired: 2 in, 2 out]
      n174 = property on="Array" class="Arr (strict)"("Value"=w346) -> ()  [unwired: 2 in, 2 out]
    }
    frame #17 {
      # "check if 1st channel of nanovoltmeter Keithley 2182 (addr. 15) is measured"
      n175 = property on="Array" class="Arr (strict)"() -> ("Value"=w361:string[])  [unwired: 2 in, 2 out]
      n176 = property on="String" class="Str"() -> ("Value"=w363:string)  [unwired: 2 in, 2 out]
      n177 = case shown="True" "Channel 1 (Vnano1)" {
        tunnel: [w365 w370] -> w362
        tunnel: w363 -> [w365 w369]
        tunnel: w361 -> [w364 w371]
        tunnel: [w364 w372] -> w360
        frame False {
          # "no , we are not measuring 1st channel\non Keithley 2182 (addr. 15)"
        }
        frame True {
          w367 = "Vnano1"
          # "yes , we are measuring 1st channel\non Keithley 2182 (addr. 15)"
          n178 = GPIB Clear(3:"15") -> ()  [unwired: 1 in, 2 out]
          n179 = Concatenate Strings(w369, w367, "\t") -> (w370:string)
          n180 = Build Array (concatenate)(w371, w367) -> (w372:string[])
        }
      }
      n181 = property on="String" class="Str"("Value"=w362) -> ()  [unwired: 2 in, 2 out]
      n182 = property on="Array" class="Arr (strict)"("Value"=w360) -> ()  [unwired: 2 in, 2 out]
    }
    frame #18 {
      # "check if 2nd channel of nanovoltmeter Keithley 2182 (addr. 15) is measured"
      n183 = property on="Array" class="Arr (strict)"() -> ("Value"=w375:string[])  [unwired: 2 in, 2 out]
      n184 = property on="String" class="Str"() -> ("Value"=w377:string)  [unwired: 2 in, 2 out]
      n185 = case shown="False" "Channel 2 (Vnano1b)" {
        tunnel: [w379 w383] -> w376
        tunnel: w377 -> [w379 w382]
        tunnel: w375 -> [w378 w384]
        tunnel: [w378 w385] -> w374
        frame False {
          # "no , we are not measuring 2nd channel\non Keithley 2182 (addr. 15)"
        }
        frame True {
          w380 = "Vnano1b"
          # "yes , we are measuring 2nd channel\non Keithley 2182 (addr. 15)"
          n186 = GPIB Clear(3:"15") -> ()  [unwired: 1 in, 2 out]
          n187 = Concatenate Strings(w382, w380, "\t") -> (w383:string)
          n188 = Build Array (concatenate)(w384, w380) -> (w385:string[])
        }
      }
      n189 = property on="String" class="Str"("Value"=w376) -> ()  [unwired: 2 in, 2 out]
      n190 = property on="Array" class="Arr (strict)"("Value"=w374) -> ()  [unwired: 2 in, 2 out]
    }
    frame #19 {
      # "check if 1st channel of nanovoltmeter Keithley 2182 (addr. 16) is measured"
      n191 = property on="Array" class="Arr (strict)"() -> ("Value"=w389:string[])  [unwired: 2 in, 2 out]
      n192 = property on="String" class="Str"() -> ("Value"=w391:string)  [unwired: 2 in, 2 out]
      n193 = case shown="True" "Channel 1 (Vnano2)" {
        tunnel: [w393 w398] -> w390
        tunnel: w391 -> [w393 w397]
        tunnel: w389 -> [w392 w399]
        tunnel: [w392 w400] -> w388
        frame False {
          # "no , we are not measuring 1st channel\non Keithley 2182 (addr. 16)"
        }
        frame True {
          w395 = "Vnano2"
          # "yes , we are measuring 1st channel\non Keithley 2182 (addr. 16)"
          n194 = GPIB Clear(3:"16") -> ()  [unwired: 1 in, 2 out]
          n195 = Concatenate Strings(w397, w395, "\t") -> (w398:string)
          n196 = Build Array (concatenate)(w399, w395) -> (w400:string[])
        }
      }
      n197 = property on="String" class="Str"("Value"=w390) -> ()  [unwired: 2 in, 2 out]
      n198 = property on="Array" class="Arr (strict)"("Value"=w388) -> ()  [unwired: 2 in, 2 out]
    }
    frame #20 {
      # "check if 2nd channel of nanovoltmeter Keithley 2182 (addr. 16) is measured"
      n199 = property on="Array" class="Arr (strict)"() -> ("Value"=w403:string[])  [unwired: 2 in, 2 out]
      n200 = property on="String" class="Str"() -> ("Value"=w405:string)  [unwired: 2 in, 2 out]
      n201 = case shown="False" "Channel 2 (Vnano2b)" {
        tunnel: [w407 w411] -> w404
        tunnel: w405 -> [w407 w410]
        tunnel: w403 -> [w406 w412]
        tunnel: [w406 w413] -> w402
        frame False {
          # "no , we are not measuring 2nd channel\non Keithley 2182 (addr. 16)"
        }
        frame True {
          w408 = "Vnano2b"
          # "yes , we are measuring 2nd channel\non Keithley 2182 (addr. 16)"
          n202 = GPIB Clear(3:"16") -> ()  [unwired: 1 in, 2 out]
          n203 = Concatenate Strings(w410, w408, "\t") -> (w411:string)
          n204 = Build Array (concatenate)(w412, w408) -> (w413:string[])
        }
      }
      n205 = property on="String" class="Str"("Value"=w404) -> ()  [unwired: 2 in, 2 out]
      n206 = property on="Array" class="Arr (strict)"("Value"=w402) -> ()  [unwired: 2 in, 2 out]
    }
    frame #21 {
      # "check if 1st channel of nanovoltmeter Keithley 2182 (addr. 17) is measured"
      n207 = property on="Array" class="Arr (strict)"() -> ("Value"=w417:string[])  [unwired: 2 in, 2 out]
      n208 = property on="String" class="Str"() -> ("Value"=w419:string)  [unwired: 2 in, 2 out]
      n209 = case shown="False" "Channel 1 (Vnano3)" {
        tunnel: [w421 w425] -> w418
        tunnel: w419 -> [w421 w424]
        tunnel: w417 -> [w420 w426]
        tunnel: [w420 w427] -> w416
        frame False {
          # "no , we are not measuring 1st channel\non Keithley 2182 (addr. 17)"
        }
        frame True {
          w422 = "Vnano3"
          # "yes , we are measuring 1st channel\non Keithley 2182 (addr. 17)"
          n210 = GPIB Clear(3:"17") -> ()  [unwired: 1 in, 2 out]
          n211 = Concatenate Strings(w424, w422, "\t") -> (w425:string)
          n212 = Build Array (concatenate)(w426, w422) -> (w427:string[])
        }
      }
      n213 = property on="String" class="Str"("Value"=w418) -> ()  [unwired: 2 in, 2 out]
      n214 = property on="Array" class="Arr (strict)"("Value"=w416) -> ()  [unwired: 2 in, 2 out]
    }
    frame #22 {
      # "check if 2nd channel of nanovoltmeter Keithley 2182 (addr. 16) is measured"
      n215 = property on="Array" class="Arr (strict)"() -> ("Value"=w431:string[])  [unwired: 2 in, 2 out]
      n216 = property on="String" class="Str"() -> ("Value"=w433:string)  [unwired: 2 in, 2 out]
      n217 = case shown="False" "Channel 2 (Vnano3b)" {
        tunnel: [w435 w439] -> w432
        tunnel: w433 -> [w435 w438]
        tunnel: w431 -> [w434 w440]
        tunnel: [w434 w441] -> w430
        frame False {
          # "no , we are not measuring 2nd channel\non Keithley 2182 (addr. 17)"
        }
        frame True {
          w436 = "Vnano3b"
          # "yes , we are measuring 2nd channel\non Keithley 2182 (addr. 17)"
          n218 = GPIB Clear(3:"17") -> ()  [unwired: 1 in, 2 out]
          n219 = Concatenate Strings(w438, w436, "\t") -> (w439:string)
          n220 = Build Array (concatenate)(w440, w436) -> (w441:string[])
        }
      }
      n221 = property on="String" class="Str"("Value"=w432) -> ()  [unwired: 2 in, 2 out]
      n222 = property on="Array" class="Arr (strict)"("Value"=w430) -> ()  [unwired: 2 in, 2 out]
    }
    frame #23 {
      # "check if 1st thermometer on Oxford ITC (address 24) is measured"
      n223 = property on="Array" class="Arr (strict)"() -> ("Value"=w445:string[])  [unwired: 2 in, 2 out]
      n224 = property on="String" class="Str"() -> ("Value"=w447:string)  [unwired: 2 in, 2 out]
      n225 = case shown="True" "Thermometer 1 (T1)" {
        tunnel: [w449 w453] -> w446
        tunnel: w447 -> [w449 w452]
        tunnel: w445 -> [w448 w454]
        tunnel: [w448 w455] -> w444
        frame False {
          # "no, we are not measuring temperature\non thermometer 1 (addr. 24)"
        }
        frame True {
          w450 = "T1"
          # "yes, we are measuring temperature,\nthermometer 1 (addr. 24)"
          n226 = GPIB Clear(3:"24") -> ()  [unwired: 1 in, 2 out]
          n227 = Concatenate Strings(w452, w450, "\t") -> (w453:string)
          n228 = Build Array (concatenate)(w454, w450) -> (w455:string[])
        }
      }
      n229 = property on="String" class="Str"("Value"=w446) -> ()  [unwired: 2 in, 2 out]
      n230 = property on="Array" class="Arr (strict)"("Value"=w444) -> ()  [unwired: 2 in, 2 out]
    }
    frame #24 {
      # "check if magnetic field from Oxford IPS 120 (address 25) is measured"
      n231 = property on="Array" class="Arr (strict)"() -> ("Value"=w459:string[])  [unwired: 2 in, 2 out]
      n232 = property on="String" class="Str"() -> ("Value"=w461:string)  [unwired: 2 in, 2 out]
      n233 = case shown="True" "Magnetic Field (B)" {
        tunnel: [w463 w467] -> w460
        tunnel: w461 -> [w463 w466]
        tunnel: w459 -> [w462 w468]
        tunnel: [w462 w469] -> w458
        frame False {
          # "no, we are not measuring magnetic field  (addr. 25)"
        }
        frame True {
          w464 = "B"
          # "yes, we are measuring magnetic field  (addr. 25)"
          n234 = GPIB Clear(3:"25") -> ()  [unwired: 1 in, 2 out]
          n235 = Concatenate Strings(w466, w464, "\t") -> (w467:string)
          n236 = Build Array (concatenate)(w468, w464) -> (w469:string[])
        }
      }
      n237 = property on="String" class="Str"("Value"=w460) -> ()  [unwired: 2 in, 2 out]
      n238 = property on="Array" class="Arr (strict)"("Value"=w458) -> ()  [unwired: 2 in, 2 out]
    }
    frame #25 {
      # "check if capacitance and loss from AH 2500 (address 28) are measured"
      n239 = property on="Array" class="Arr (strict)"() -> ("Value"=w473:string[])  [unwired: 2 in, 2 out]
      n240 = property on="String" class="Str"() -> ("Value"=w475:string)  [unwired: 2 in, 2 out]
      n241 = case shown="False" "Capacitance (C) and Loss (L)" {
        tunnel: [w477 w486] -> w474
        tunnel: w475 -> [w477 w479]
        tunnel: w473 -> [w476 w481]
        tunnel: [w476 w487] -> w472
        frame False {
          # "no, we are not measuring capacitance  (addr. 28)"
        }
        frame True {
          w482 = "C"
          w484 = "L"
          # "yes, we are measuring capacitance and loss  (addr. 28)"
          n242 = GPIB Clear(3:"28") -> ()  [unwired: 1 in, 2 out]
          n243 = Concatenate Strings(w479, w482, "\t") -> (w478:string)
          n244 = Build Array (concatenate)(w481, w482) -> (w480:string[])
          n245 = Concatenate Strings(w478, w484, "\t") -> (w486:string)
          n246 = Build Array (concatenate)(w480, w484) -> (w487:string[])
        }
      }
      n247 = property on="String" class="Str"("Value"=w474) -> ()  [unwired: 2 in, 2 out]
      n248 = property on="Array" class="Arr (strict)"("Value"=w472) -> ()  [unwired: 2 in, 2 out]
    }
  }
  n249 = property on="Array" class="Arr (strict)"(error in=w19) -> (error out=w2:errorcluster, "Value"=w9:string[])  [unwired: 1 in, 1 out]
  n250 = property on="String" class="Str"(error in=w2) -> ("Value"=w5:string)  [unwired: 1 in, 2 out]
  n251 = property on="Commutator" class="Bool (strict)"() -> ("Value"=w8:bool)  [unwired: 2 in, 2 out]
  n252 = case shown="False" w8 {
    tunnel: w9 -> [w491 w509]
    tunnel: [w489 w509] -> w6
    tunnel: w5 -> [w493 w508]
    tunnel: [w492 w508] -> w4
    frame True {
      n253 = Array Size(array=w491) -> (size(s)=w495:i32)
      n254 = Decrement(x=w495) -> (x-1=w494:i32)
      n255 = for {
        N: w494 -> [_]
        shift-right: [w506] -> w490
        shift-left: string[] [] -> [w507]
        shift-right: [w498] -> w492
        shift-left: w493 -> [w499]
        i -> [w503]
        n256 = property on="Array" class="Arr (strict)"() -> ("Value"=w501:string[])  [unwired: 2 in, 2 out]
        n257 = Increment(x=w503) -> (x+1=w502:i32)
        n258 = Index Array(array=w501, index=w502) -> (element=w505:string)
        n259 = Concatenate Strings("c", w505) -> (w497:string)
        n260 = Concatenate Strings(w499, w497, "\t") -> (w498:string)
        n261 = Build Array (concatenate)(w507, w497) -> (w506:string[])
      }
      n262 = Build Array (concatenate)(w491, w490) -> (w489:string[])
      n263 = property on="Array" class="Arr (strict)"("Value"=w489) -> ()  [unwired: 2 in, 2 out]
    }
    frame False {
    }
  }
  n264 = Concatenate Strings(w4, "\r", "\n") -> (w15:string)
  "String" <- w15
  n265 = property on="Ring" class="Ring (strict)"("Strings []"=w6) -> (error out=w3:errorcluster)  [unwired: 2 in, 1 out]
  n266 = property on="Data file:" class="Path"(error in=w3) -> (error out=w14:errorcluster, "Value"=w16:path)  [unwired: 1 in, 1 out]
  n267 = while {
    tunnel: w14 -> [w524]
    shift-right: [w521] -> w13
    shift-left: dbl[][] [] -> [w523]
    shift-right: [w514] -> _
    shift-left: w1 -> [w520]
    tunnel: "points at each Vg" -> [w516]
    tunnel: [w512] -> w11
    stop <- w522 stop-if-true
    w512 = 1e-08
    # "send new B value to Magnet"
    n268 = for {
      N: w516 -> [_]
      tunnel: w524 -> [w550]
      tunnel: [w567] -> w522
      shift-right: [w555] -> w521
      shift-left: w523 -> [w574]
      tunnel: w520 -> [w565]
      tunnel: [w570] -> w514
      w566 = dbl[] []  # Empty array for data
      # "Number of Points"
      # "Time"
      # "Swep up or down?"
      # "Absolute\nDifference"
      # "this part appends last\nmeasured point to the \ndata file"
      # "this line is current gate voltage"
      # "First we create an empty array \nfor data and write the first element \ninto it - current gate voltage"
      # "time is measured at the beginning\nand at the end of the cycle to\ncalculate delay time required to\nkeep set sweep rate"
      # "this part calculate resistances and current (if needed) from voltages measured by lock-in amplifiers"
      # "check if the next step doesn't\ngo beyond the target voltage"
      # "calculate difference between target and current B"
      # "check if we are at the target voltage yet"
      # "in this part we calculate incriment for B"
      n269 = flat-sequence {
        tunnel: w550 -> [w1752]
        tunnel: [w1752] -> w548
        tunnel: [w1754] -> w549
        tunnel: w548 -> [w1754]
        tunnel: [w1753] -> w547
        frame #0 {
          n270 = property on="Deliberate Time delay" class="DigNum (strict)"() -> ("Value"=w1751:i32)  [unwired: 2 in, 2 out]
          n271 = Wait (ms)(milliseconds to wait=w1751) -> ()  [unwired: 1 out]
        }
        frame #1 {
          n272 = Tick Count (ms)() -> (millisecond timer value=w1753:u32)
        }
      }
      n273 = Build Array (concatenate)(w566, w565) -> (w564:dbl[])
      n274 = property on="array for data" class="Arr (strict)"(error in=w549, "Value"=w564) -> (error out=w563:errorcluster)  [unwired: 1 in, 1 out]
      n275 = case shown="True" "Commutator" {
        tunnel: [w601 w1381] -> w575
        tunnel: w563 -> [w602 w1380]
        frame True {
          n276 = stacked-sequence {
            tunnel: w602 -> [w619 w1008]
            tunnel: [_ w993] -> w601
            frame #0 {
              n277 = stacked-sequence {
                tunnel: w619 -> [w623 _ _ _ _ _ _ _ _ _ _ _ _ _ _ _ _ _ _ _ _ _ _ _ _ _]
                tunnel: [w623 _ _ _ _ _ _ _ _ _ _ _ _ _ _ _ _ _ _ _ _ _ _ _ _ _] -> w603
                frame #0 {
                  # "check if oscillator on \nlock-in (address 1)\nis to be measured"
                  n278 = property on="Current is:" class="RadioBtnsControl (strict)"() -> ("Value"=w626:T1)  [unwired: 2 in, 2 out]
                  n279 = property on="array for data" class="Arr (strict)"() -> ("Value"=w625:dbl[])  [unwired: 2 in, 2 out]
                  n280 = Equal?(x=w626, y=1) -> (x = y?=w627:bool)
                  n281 = case shown="True" w627 {
                    tunnel: w625 -> [w629 w637]
                    tunnel: [w629 w636] -> w624
                    frame False {
                      # "we are not measuring oscillator from\nlock-in (address 1)"
                    }
                    frame True {
                      w633 = "1"
                      # "we are  measuring oscillator"
                      n282 = GPIB Write(0:w633, 1:"SLVL?") -> (6:w634:errorcluster)  [unwired: 3 in, 1 out]
                      n283 = GPIB Read(0:w633, 1:3200, 3:w634) -> (5:w631:string)  [unwired: 2 in, 2 out]
                      n284 = Fract/Exp String To Number(string=w631) -> (number=w630:dbl)  [unwired: 3 in, 1 out]
                      n285 = Build Array (concatenate)(w637, w630) -> (w636:dbl[])
                    }
                  }
                  n286 = property on="array for data" class="Arr (strict)"("Value"=w624) -> ()  [unwired: 2 in, 2 out]
                }
                frame #1 {
                  # "check if in-phase\nsignal on lock-in \n(address 1) is to\nbe measured"
                  n287 = property on="array for data" class="Arr (strict)"() -> ("Value"=w640:dbl[])  [unwired: 2 in, 2 out]
                  n288 = property on="Addr 1 lock-in" class="Bool (strict)"() -> ("Value"=w638:bool)  [unwired: 2 in, 2 out]
                  n289 = case shown="False" w638 {
                    tunnel: w640 -> [w641 w649]
                    tunnel: [w641 w648] -> w639
                    frame False {
                      # "we are not measuring in phase signal on lock-in (address 1)"
                    }
                    frame True {
                      w646 = "1"
                      # "we are  measuring lock-in (address 1), in phase"
                      n290 = GPIB Write(0:w646, 1:"OUTP?1") -> (6:w647:errorcluster)  [unwired: 3 in, 1 out]
                      n291 = GPIB Read(0:w646, 1:3200, 3:w647) -> (5:w644:string)  [unwired: 2 in, 2 out]
                      n292 = Fract/Exp String To Number(string=w644) -> (number=w643:dbl)  [unwired: 3 in, 1 out]
                      n293 = Build Array (concatenate)(w649, w643) -> (w648:dbl[])
                    }
                  }
                  n294 = property on="array for data" class="Arr (strict)"("Value"=w639) -> ()  [unwired: 2 in, 2 out]
                }
                frame #2 {
                  # "check if out-of-phase\nsignal on lock-in \n(address 1) is to\nbe measured"
                  n295 = property on="Addr 1 lock-in oop" class="Bool (strict)"() -> ("Value"=w650:bool)  [unwired: 2 in, 2 out]
                  n296 = property on="array for data" class="Arr (strict)"() -> ("Value"=w652:dbl[])  [unwired: 2 in, 2 out]
                  n297 = case shown="False" w650 {
                    tunnel: w652 -> [w653 w661]
                    tunnel: [w653 w660] -> w651
                    frame False {
                      # "we are not measuring out-of-phase signal on lock-in (address 1)"
                    }
                    frame True {
                      w658 = "1"
                      # "we are  measuring lock-in (address 1), out-of-phase signal"
                      n298 = GPIB Write(0:w658, 1:"OUTP?2") -> (6:w659:errorcluster)  [unwired: 3 in, 1 out]
                      n299 = GPIB Read(0:w658, 1:3200, 3:w659) -> (5:w656:string)  [unwired: 2 in, 2 out]
                      n300 = Fract/Exp String To Number(string=w656) -> (number=w655:dbl)  [unwired: 3 in, 1 out]
                      n301 = Build Array (concatenate)(w661, w655) -> (w660:dbl[])
                    }
                  }
                  n302 = property on="array for data" class="Arr (strict)"("Value"=w651) -> ()  [unwired: 2 in, 2 out]
                }
                frame #3 {
                  # "check if in-phase\nsignal on lock-in \n(address 2) is to\nbe measured"
                  n303 = property on="Addr 2 lock-in" class="Bool (strict)"() -> ("Value"=w662:bool)  [unwired: 2 in, 2 out]
                  n304 = property on="array for data" class="Arr (strict)"() -> ("Value"=w664:dbl[])  [unwired: 2 in, 2 out]
                  n305 = case shown="False" w662 {
                    tunnel: w664 -> [w665 w673]
                    tunnel: [w665 w672] -> w663
                    frame False {
                      # "we are not measuring in phase signal on lock-in (address 2)"
                    }
                    frame True {
                      w670 = "2"
                      # "we are  measuring lock-in (address 2), in phase"
                      n306 = GPIB Write(0:w670, 1:"OUTP?1") -> (6:w671:errorcluster)  [unwired: 3 in, 1 out]
                      n307 = GPIB Read(0:w670, 1:3200, 3:w671) -> (5:w668:string)  [unwired: 2 in, 2 out]
                      n308 = Fract/Exp String To Number(string=w668) -> (number=w667:dbl)  [unwired: 3 in, 1 out]
                      n309 = Build Array (concatenate)(w673, w667) -> (w672:dbl[])
                    }
                  }
                  n310 = property on="array for data" class="Arr (strict)"("Value"=w663) -> ()  [unwired: 2 in, 2 out]
                }
                frame #4 {
                  # "check if out-of-phase\nsignal on lock-in \n(address 2) is to\nbe measured"
                  n311 = property on="Addr 2 lock-in oop" class="Bool (strict)"() -> ("Value"=w674:bool)  [unwired: 2 in, 2 out]
                  n312 = property on="array for data" class="Arr (strict)"() -> ("Value"=w676:dbl[])  [unwired: 2 in, 2 out]
                  n313 = case shown="False" w674 {
                    tunnel: w676 -> [w677 w685]
                    tunnel: [w677 w684] -> w675
                    tunnel: w674 -> [_ _]
                    frame False {
                      # "we are not measuring out-of-phase signal on lock-in (address 2)"
                    }
                    frame True {
                      w682 = "2"
                      # "we are  measuring lock-in (address 2), out-of-phase"
                      n314 = GPIB Write(0:w682, 1:"OUTP?2") -> (6:w683:errorcluster)  [unwired: 3 in, 1 out]
                      n315 = GPIB Read(0:w682, 1:3200, 3:w683) -> (5:w680:string)  [unwired: 2 in, 2 out]
                      n316 = Fract/Exp String To Number(string=w680) -> (number=w679:dbl)  [unwired: 3 in, 1 out]
                      n317 = Build Array (concatenate)(w685, w679) -> (w684:dbl[])
                    }
                  }
                  n318 = property on="array for data" class="Arr (strict)"("Value"=w675) -> ()  [unwired: 2 in, 2 out]
                }
                frame #5 {
                  # "check if in-phase\nsignal on lock-in \n(address 3) is to\nbe measured"
                  n319 = property on="Addr 3 lock-in" class="Bool (strict)"() -> ("Value"=w686:bool)  [unwired: 2 in, 2 out]
                  n320 = property on="array for data" class="Arr (strict)"() -> ("Value"=w688:dbl[])  [unwired: 2 in, 2 out]
                  n321 = case shown="False" w686 {
                    tunnel: w688 -> [w689 w697]
                    tunnel: [w689 w696] -> w687
                    frame False {
                      # "we are not measuring in phase signal on lock-in (address 3)"
                    }
                    frame True {
                      w694 = "3"
                      # "we are  measuring lock-in (address 3), in phase"
                      n322 = GPIB Write(0:w694, 1:"OUTP?1") -> (6:w695:errorcluster)  [unwired: 3 in, 1 out]
                      n323 = GPIB Read(0:w694, 1:3200, 3:w695) -> (5:w692:string)  [unwired: 2 in, 2 out]
                      n324 = Fract/Exp String To Number(string=w692) -> (number=w691:dbl)  [unwired: 3 in, 1 out]
                      n325 = Build Array (concatenate)(w697, w691) -> (w696:dbl[])
                    }
                  }
                  n326 = property on="array for data" class="Arr (strict)"("Value"=w687) -> ()  [unwired: 2 in, 2 out]
                }
                frame #6 {
                  # "check if out-of-phase\nsignal on lock-in \n(address 3) is to\nbe measured"
                  n327 = property on="Addr 3 lock-in oop" class="Bool (strict)"() -> ("Value"=w698:bool)  [unwired: 2 in, 2 out]
                  n328 = property on="array for data" class="Arr (strict)"() -> ("Value"=w700:dbl[])  [unwired: 2 in, 2 out]
                  n329 = case shown="False" w698 {
                    tunnel: w700 -> [w701 w709]
                    tunnel: [w701 w708] -> w699
                    frame False {
                      # "we are not measuring out-of-phase signal on lock-in (address 3)"
                    }
                    frame True {
                      w706 = "3"
                      # "we are  measuring lock-in (address 3), out-of-phase"
                      n330 = GPIB Write(0:w706, 1:"OUTP?2") -> (6:w707:errorcluster)  [unwired: 3 in, 1 out]
                      n331 = GPIB Read(0:w706, 1:3200, 3:w707) -> (5:w704:string)  [unwired: 2 in, 2 out]
                      n332 = Fract/Exp String To Number(string=w704) -> (number=w703:dbl)  [unwired: 3 in, 1 out]
                      n333 = Build Array (concatenate)(w709, w703) -> (w708:dbl[])
                    }
                  }
                  n334 = property on="array for data" class="Arr (strict)"("Value"=w699) -> ()  [unwired: 2 in, 2 out]
                }
                frame #7 {
                  # "check if in-phase\nsignal on lock-in \n(address 4) is to\nbe measured"
                  n335 = property on="Addr 4 lock-in" class="Bool (strict)"() -> ("Value"=w710:bool)  [unwired: 2 in, 2 out]
                  n336 = property on="array for data" class="Arr (strict)"() -> ("Value"=w712:dbl[])  [unwired: 2 in, 2 out]
                  n337 = case shown="False" w710 {
                    tunnel: w712 -> [w713 w721]
                    tunnel: [w713 w720] -> w711
                    frame False {
                      # "we are not measuring in phase signal on lock-in (address 4)"
                    }
                    frame True {
                      w718 = "4"
                      # "we are  measuring lock-in (address 4), in phase"
                      n338 = GPIB Write(0:w718, 1:"OUTP?1") -> (6:w719:errorcluster)  [unwired: 3 in, 1 out]
                      n339 = GPIB Read(0:w718, 1:3200, 3:w719) -> (5:w716:string)  [unwired: 2 in, 2 out]
                      n340 = Fract/Exp String To Number(string=w716) -> (number=w715:dbl)  [unwired: 3 in, 1 out]
                      n341 = Build Array (concatenate)(w721, w715) -> (w720:dbl[])
                    }
                  }
                  n342 = property on="array for data" class="Arr (strict)"("Value"=w711) -> ()  [unwired: 2 in, 2 out]
                }
                frame #8 {
                  # "check if out-of-phase\nsignal on lock-in \n(address 4) is to\nbe measured"
                  n343 = property on="Addr 4 lock-in oop" class="Bool (strict)"() -> ("Value"=w722:bool)  [unwired: 2 in, 2 out]
                  n344 = property on="array for data" class="Arr (strict)"() -> ("Value"=w724:dbl[])  [unwired: 2 in, 2 out]
                  n345 = case shown="False" w722 {
                    tunnel: w724 -> [w725 w733]
                    tunnel: [w725 w732] -> w723
                    frame False {
                      # "we are not measuring out-of-phase signal on lock-in (address 4)"
                    }
                    frame True {
                      w730 = "4"
                      # "we are  measuring lock-in (address 4), out-of-phase"
                      n346 = GPIB Write(0:w730, 1:"OUTP?2") -> (6:w731:errorcluster)  [unwired: 3 in, 1 out]
                      n347 = GPIB Read(0:w730, 1:3200, 3:w731) -> (5:w728:string)  [unwired: 2 in, 2 out]
                      n348 = Fract/Exp String To Number(string=w728) -> (number=w727:dbl)  [unwired: 3 in, 1 out]
                      n349 = Build Array (concatenate)(w733, w727) -> (w732:dbl[])
                    }
                  }
                  n350 = property on="array for data" class="Arr (strict)"("Value"=w723) -> ()  [unwired: 2 in, 2 out]
                }
                frame #9 {
                  # "check if in-phase\nsignal on lock-in \n(address 5) is to\nbe measured"
                  n351 = property on="Addr 5 lock-in" class="Bool (strict)"() -> ("Value"=w734:bool)  [unwired: 2 in, 2 out]
                  n352 = property on="array for data" class="Arr (strict)"() -> ("Value"=w736:dbl[])  [unwired: 2 in, 2 out]
                  n353 = case shown="False" w734 {
                    tunnel: w736 -> [w737 w745]
                    tunnel: [w737 w744] -> w735
                    frame False {
                      # "we are not measuring in phase signal on lock-in (address 5)"
                    }
                    frame True {
                      w742 = "5"
                      # "we are  measuring lock-in (address 5), in phase"
                      n354 = GPIB Write(0:w742, 1:"OUTP?1") -> (6:w743:errorcluster)  [unwired: 3 in, 1 out]
                      n355 = GPIB Read(0:w742, 1:3200, 3:w743) -> (5:w740:string)  [unwired: 2 in, 2 out]
                      n356 = Fract/Exp String To Number(string=w740) -> (number=w739:dbl)  [unwired: 3 in, 1 out]
                      n357 = Build Array (concatenate)(w745, w739) -> (w744:dbl[])
                    }
                  }
                  n358 = property on="array for data" class="Arr (strict)"("Value"=w735) -> ()  [unwired: 2 in, 2 out]
                }
                frame #10 {
                  # "check if out-of-phase\nsignal on lock-in \n(address 5) is to\nbe measured"
                  n359 = property on="Addr 5 lock-in oop" class="Bool (strict)"() -> ("Value"=w746:bool)  [unwired: 2 in, 2 out]
                  n360 = property on="array for data" class="Arr (strict)"() -> ("Value"=w748:dbl[])  [unwired: 2 in, 2 out]
                  n361 = case shown="False" w746 {
                    tunnel: w748 -> [w749 w757]
                    tunnel: [w749 w756] -> w747
                    frame False {
                      # "we are not measuring out-of-phase signal on lock-in (address 5)"
                    }
                    frame True {
                      w754 = "5"
                      # "we are  measuring lock-in (address 5), out-of-phase"
                      n362 = GPIB Write(0:w754, 1:"OUTP?2") -> (6:w755:errorcluster)  [unwired: 3 in, 1 out]
                      n363 = GPIB Read(0:w754, 1:3200, 3:w755) -> (5:w752:string)  [unwired: 2 in, 2 out]
                      n364 = Fract/Exp String To Number(string=w752) -> (number=w751:dbl)  [unwired: 3 in, 1 out]
                      n365 = Build Array (concatenate)(w757, w751) -> (w756:dbl[])
                    }
                  }
                  n366 = property on="array for data" class="Arr (strict)"("Value"=w747) -> ()  [unwired: 2 in, 2 out]
                }
                frame #11 {
                  # "check if voltage on \nmain Keithley 2400 \n(addr. 12) is to\nbe measured"
                  n367 = property on="Voltage (Vk1)" class="Bool (strict)"() -> ("Value"=w758:bool)  [unwired: 2 in, 2 out]
                  n368 = property on="array for data" class="Arr (strict)"() -> ("Value"=w760:dbl[])  [unwired: 2 in, 2 out]
                  n369 = case shown="False" w758 {
                    tunnel: w760 -> [w761 w771]
                    tunnel: [w761 w770] -> w759
                    frame False {
                      # "we aren't measuring voltage \non main Keithley 2400 (addr. 12)"
                    }
                    frame True {
                      w768 = "12"
                      # "we are measuring voltage \non main Keithley 2400 (addr. 12)"
                      n370 = GPIB Write(0:w768, 1:":READ?") -> (6:w769:errorcluster)  [unwired: 3 in, 1 out]
                      n371 = GPIB Read(0:w768, 1:3200, 3:w769) -> (5:w764:string)  [unwired: 2 in, 2 out]
                      n372 = String Subset(string=w764, length (rest)=13) -> (substring=w763:string)  [unwired: 1 in]
                      n373 = Fract/Exp String To Number(string=w763) -> (number=w766:dbl)  [unwired: 3 in, 1 out]
                      n374 = Build Array (concatenate)(w771, w766) -> (w770:dbl[])
                    }
                  }
                  n375 = property on="array for data" class="Arr (strict)"("Value"=w759) -> ()  [unwired: 2 in, 2 out]
                }
                frame #12 {
                  # "check if  current on \nmain Keithley 2400 \n(addr. 12) is to\nbe measured"
                  n376 = property on="Current (Ik1)" class="Bool (strict)"() -> ("Value"=w772:bool)  [unwired: 2 in, 2 out]
                  n377 = property on="array for data" class="Arr (strict)"() -> ("Value"=w774:dbl[])  [unwired: 2 in, 2 out]
                  n378 = case shown="True" w772 {
                    tunnel: w774 -> [w775 w786]
                    tunnel: [w775 w785] -> w773
                    frame False {
                      # "we aren't measuring current \non main Keithley 2400 (addr. 12)"
                    }
                    frame True {
                      w783 = "12"
                      # "we are measuring current\non main Keithley 2400 (addr. 12)"
                      n379 = GPIB Write(0:w783, 1:":READ?") -> (6:w784:errorcluster)  [unwired: 3 in, 1 out]
                      n380 = GPIB Read(0:w783, 1:3200, 3:w784) -> (5:w779:string)  [unwired: 2 in, 2 out]
                      n381 = String Subset(string=w779, offset (0)=14, length (rest)=13) -> (substring=w778:string)
                      n382 = Fract/Exp String To Number(string=w778) -> (number=w781:dbl)  [unwired: 3 in, 1 out]
                      n383 = Build Array (concatenate)(w786, w781) -> (w785:dbl[])
                    }
                  }
                  n384 = property on="array for data" class="Arr (strict)"("Value"=w773) -> ()  [unwired: 2 in, 2 out]
                }
                frame #13 {
                  # "check if voltage on \nadd. Keithley 2400 \n(addr. 13) is to\nbe measured"
                  n385 = property on="Voltage (Vk2)" class="Bool (strict)"() -> ("Value"=w787:bool)  [unwired: 2 in, 2 out]
                  n386 = property on="array for data" class="Arr (strict)"() -> ("Value"=w789:dbl[])  [unwired: 2 in, 2 out]
                  n387 = case shown="True" w787 {
                    tunnel: w789 -> [w790 w800]
                    tunnel: [w790 w799] -> w788
                    frame False {
                      # "we aren't measuring voltage \non additional Keithley 2400 (addr. 13)"
                    }
                    frame True {
                      w797 = "13"
                      # "we are measuring voltage \non additional Keithley 2400 (addr. 13)"
                      n388 = GPIB Write(0:w797, 1:":READ?") -> (6:w798:errorcluster)  [unwired: 3 in, 1 out]
                      n389 = GPIB Read(0:w797, 1:3200, 3:w798) -> (5:w793:string)  [unwired: 2 in, 2 out]
                      n390 = String Subset(string=w793, length (rest)=13) -> (substring=w792:string)  [unwired: 1 in]
                      n391 = Fract/Exp String To Number(string=w792) -> (number=w795:dbl)  [unwired: 3 in, 1 out]
                      n392 = Build Array (concatenate)(w800, w795) -> (w799:dbl[])
                    }
                  }
                  n393 = property on="array for data" class="Arr (strict)"("Value"=w788) -> ()  [unwired: 2 in, 2 out]
                }
                frame #14 {
                  # "check if  current on \nadd. Keithley 2400 \n(addr. 13) is to\nbe measured"
                  n394 = property on="Current (Ik2)" class="Bool (strict)"() -> ("Value"=w801:bool)  [unwired: 2 in, 2 out]
                  n395 = property on="array for data" class="Arr (strict)"() -> ("Value"=w803:dbl[])  [unwired: 2 in, 2 out]
                  n396 = case shown="True" w801 {
                    tunnel: w803 -> [w804 w815]
                    tunnel: [w804 w814] -> w802
                    frame False {
                      # "we aren't measuring current \non additional Keithley 2400 (addr. 13)"
                    }
                    frame True {
                      w812 = "13"
                      # "we are measuring current\non additional Keithley 2400 (addr. 13)"
                      n397 = GPIB Write(0:w812, 1:":READ?") -> (6:w813:errorcluster)  [unwired: 3 in, 1 out]
                      n398 = GPIB Read(0:w812, 1:3200, 3:w813) -> (5:w808:string)  [unwired: 2 in, 2 out]
                      n399 = String Subset(string=w808, offset (0)=14, length (rest)=13) -> (substring=w807:string)
                      n400 = Fract/Exp String To Number(string=w807) -> (number=w810:dbl)  [unwired: 3 in, 1 out]
                      n401 = Build Array (concatenate)(w815, w810) -> (w814:dbl[])
                    }
                  }
                  n402 = property on="array for data" class="Arr (strict)"("Value"=w802) -> ()  [unwired: 2 in, 2 out]
                }
                frame #15 {
                  # "check if voltage on \nadd. Keithley 2400 \n(addr. 14) is to\nbe measured"
                  n403 = property on="Voltage (Vk3)" class="Bool (strict)"() -> ("Value"=w816:bool)  [unwired: 2 in, 2 out]
                  n404 = property on="array for data" class="Arr (strict)"() -> ("Value"=w818:dbl[])  [unwired: 2 in, 2 out]
                  n405 = case shown="True" w816 {
                    tunnel: w818 -> [w819 w829]
                    tunnel: [w819 w828] -> w817
                    frame False {
                      # "we aren't measuring voltage \non additional Keithley 2400 (addr. 14)"
                    }
                    frame True {
                      w826 = "14"
                      # "we are measuring voltage \non additional Keithley 2400 (addr. 14)"
                      n406 = GPIB Write(0:w826, 1:":READ?") -> (6:w827:errorcluster)  [unwired: 3 in, 1 out]
                      n407 = GPIB Read(0:w826, 1:3200, 3:w827) -> (5:w822:string)  [unwired: 2 in, 2 out]
                      n408 = String Subset(string=w822, length (rest)=13) -> (substring=w821:string)  [unwired: 1 in]
                      n409 = Fract/Exp String To Number(string=w821) -> (number=w824:dbl)  [unwired: 3 in, 1 out]
                      n410 = Build Array (concatenate)(w829, w824) -> (w828:dbl[])
                    }
                  }
                  n411 = property on="array for data" class="Arr (strict)"("Value"=w817) -> ()  [unwired: 2 in, 2 out]
                }
                frame #16 {
                  # "check if  current on \nadd. Keithley 2400 \n(addr. 14) is to\nbe measured"
                  n412 = property on="Current (Ik3)" class="Bool (strict)"() -> ("Value"=w830:bool)  [unwired: 2 in, 2 out]
                  n413 = property on="array for data" class="Arr (strict)"() -> ("Value"=w832:dbl[])  [unwired: 2 in, 2 out]
                  n414 = case shown="True" w830 {
                    tunnel: w832 -> [w833 w844]
                    tunnel: [w833 w843] -> w831
                    frame False {
                      # "we aren't measuring current \non additional Keithley 2400 (addr. 14)"
                    }
                    frame True {
                      w841 = "14"
                      # "we are measuring current\non additional Keithley 2400 (addr. 14)"
                      n415 = GPIB Write(0:w841, 1:":READ?") -> (6:w842:errorcluster)  [unwired: 3 in, 1 out]
                      n416 = GPIB Read(0:w841, 1:3200, 3:w842) -> (5:w837:string)  [unwired: 2 in, 2 out]
                      n417 = String Subset(string=w837, offset (0)=14, length (rest)=13) -> (substring=w836:string)
                      n418 = Fract/Exp String To Number(string=w836) -> (number=w839:dbl)  [unwired: 3 in, 1 out]
                      n419 = Build Array (concatenate)(w844, w839) -> (w843:dbl[])
                    }
                  }
                  n420 = property on="array for data" class="Arr (strict)"("Value"=w831) -> ()  [unwired: 2 in, 2 out]
                }
                frame #17 {
                  # "check if 1st channel\non Keithley 2182 \n(addr. 15) is to\nbe measured"
                  n421 = property on="Channel 1 (Vnano1)" class="Bool (strict)"() -> ("Value"=w845:bool)  [unwired: 2 in, 2 out]
                  n422 = property on="array for data" class="Arr (strict)"() -> ("Value"=w847:dbl[])  [unwired: 2 in, 2 out]
                  n423 = case shown="True" w845 {
                    tunnel: w847 -> [w848 w856]
                    tunnel: [w848 w855] -> w846
                    frame False {
                      # "we are not measuring 1st channel\non Keithley 2182 (addr. 15)"
                    }
                    frame True {
                      w853 = "15"
                      # "we are measuring 1st channel\non Keithley 2182 (addr. 15)"
                      n424 = GPIB Write(0:w853, 1:":SENSe:DATA:FRES?") -> (6:w854:errorcluster)  [unwired: 3 in, 1 out]
                      n425 = GPIB Read(0:w853, 1:200, 3:w854) -> (5:w849:string)  [unwired: 2 in, 2 out]
                      n426 = Fract/Exp String To Number(string=w849) -> (number=w851:dbl)  [unwired: 3 in, 1 out]
                      n427 = Build Array (concatenate)(w856, w851) -> (w855:dbl[])
                    }
                  }
                  n428 = property on="array for data" class="Arr (strict)"("Value"=w846) -> ()  [unwired: 2 in, 2 out]
                }
                frame #18 {
                  # "check if 2nd channel\non Keithley 2182 \n(addr. 15) is to\nbe measured"
                  n429 = property on="Channel 2 (Vnano1b)" class="Bool (strict)"() -> ("Value"=w857:bool)  [unwired: 2 in, 2 out]
                  n430 = property on="array for data" class="Arr (strict)"() -> ("Value"=w859:dbl[])  [unwired: 2 in, 2 out]
                  n431 = case shown="False" w857 {
                    tunnel: w859 -> [w860 w872]
                    tunnel: [w860 w871] -> w858
                    frame False {
                      # "we are not measuring 1st channel\non Keithley 2182 (addr. 15)"
                    }
                    frame True {
                      w863 = "15"
                      # "switching to channel 2 and then\nback to channel 1"
                      # "we are measuring 2nd channel\non Keithley 2182 (addr. 15)"
                      n432 = GPIB Write(0:w863, 1:":SENSe:CHAN 2") -> (6:w864:errorcluster)  [unwired: 3 in, 1 out]
                      n433 = GPIB Write(0:w863, 1:":SENSe:DATA:FRES?", 3:w864) -> (6:w870:errorcluster)  [unwired: 2 in, 1 out]
                      n434 = GPIB Read(0:w863, 1:200, 3:w870) -> (5:w866:string, 7:w862:errorcluster)  [unwired: 2 in, 1 out]
                      n435 = GPIB Write(0:w863, 1:":SENSe:CHAN 1", 3:w862) -> ()  [unwired: 2 in, 2 out]
                      n436 = Fract/Exp String To Number(string=w866) -> (number=w868:dbl)  [unwired: 3 in, 1 out]
                      n437 = Build Array (concatenate)(w872, w868) -> (w871:dbl[])
                    }
                  }
                  n438 = property on="array for data" class="Arr (strict)"("Value"=w858) -> ()  [unwired: 2 in, 2 out]
                }
                frame #19 {
                  # "check if 1st channel\non Keithley 2182 \n(addr. 16) is to\nbe measured"
                  n439 = property on="Channel 1 (Vnano2)" class="Bool (strict)"() -> ("Value"=w873:bool)  [unwired: 2 in, 2 out]
                  n440 = property on="array for data" class="Arr (strict)"() -> ("Value"=w875:dbl[])  [unwired: 2 in, 2 out]
                  n441 = case shown="True" w873 {
                    tunnel: w875 -> [w876 w884]
                    tunnel: [w876 w883] -> w874
                    frame False {
                      # "we are not measuring 1st channel\non Keithley 2182 (addr. 16)"
                    }
                    frame True {
                      w881 = "16"
                      # "we are measuring 1st channel\non Keithley 2182 (addr. 16)"
                      n442 = GPIB Write(0:w881, 1:":SENSe:DATA:FRES?") -> (6:w882:errorcluster)  [unwired: 3 in, 1 out]
                      n443 = GPIB Read(0:w881, 1:200, 3:w882) -> (5:w877:string)  [unwired: 2 in, 2 out]
                      n444 = Fract/Exp String To Number(string=w877) -> (number=w879:dbl)  [unwired: 3 in, 1 out]
                      n445 = Build Array (concatenate)(w884, w879) -> (w883:dbl[])
                    }
                  }
                  n446 = property on="array for data" class="Arr (strict)"("Value"=w874) -> ()  [unwired: 2 in, 2 out]
                }
                frame #20 {
                  # "check if 2nd channel\non Keithley 2182 \n(addr. 16) is to\nbe measured"
                  n447 = property on="Channel 2 (Vnano2b)" class="Bool (strict)"() -> ("Value"=w885:bool)  [unwired: 2 in, 2 out]
                  n448 = property on="array for data" class="Arr (strict)"() -> ("Value"=w887:dbl[])  [unwired: 2 in, 2 out]
                  n449 = case shown="False" w885 {
                    tunnel: w887 -> [w888 w900]
                    tunnel: [w888 w899] -> w886
                    frame False {
                      # "we are not measuring 1st channel\non Keithley 2182 (addr. 16)"
                    }
                    frame True {
                      w891 = "16"
                      # "switching to channel 2 and then\nback to channel 1"
                      # "we are measuring 2nd channel\non Keithley 2182 (addr. 16)"
                      n450 = GPIB Write(0:w891, 1:":SENSe:CHAN 2") -> (6:w892:errorcluster)  [unwired: 3 in, 1 out]
                      n451 = GPIB Write(0:w891, 1:":SENSe:DATA:FRES?", 3:w892) -> (6:w898:errorcluster)  [unwired: 2 in, 1 out]
                      n452 = GPIB Read(0:w891, 1:200, 3:w898) -> (5:w894:string, 7:w890:errorcluster)  [unwired: 2 in, 1 out]
                      n453 = GPIB Write(0:w891, 1:":SENSe:CHAN 1", 3:w890) -> ()  [unwired: 2 in, 2 out]
                      n454 = Fract/Exp String To Number(string=w894) -> (number=w896:dbl)  [unwired: 3 in, 1 out]
                      n455 = Build Array (concatenate)(w900, w896) -> (w899:dbl[])
                    }
                  }
                  n456 = property on="array for data" class="Arr (strict)"("Value"=w886) -> ()  [unwired: 2 in, 2 out]
                }
                frame #21 {
                  # "check if 1st channel\non Keithley 2182 \n(addr. 17) is to\nbe measured"
                  n457 = property on="Channel 1 (Vnano3)" class="Bool (strict)"() -> ("Value"=w901:bool)  [unwired: 2 in, 2 out]
                  n458 = property on="array for data" class="Arr (strict)"() -> ("Value"=w903:dbl[])  [unwired: 2 in, 2 out]
                  n459 = case shown="True" w901 {
                    tunnel: w903 -> [w904 w912]
                    tunnel: [w904 w911] -> w902
                    frame False {
                      # "we are not measuring 1st channel\non Keithley 2182 (addr. 17)"
                    }
                    frame True {
                      w909 = "17"
                      # "we are measuring 1st channel\non Keithley 2182 (addr. 17)"
                      n460 = GPIB Write(0:w909, 1:":SENSe:DATA:FRES?") -> (6:w910:errorcluster)  [unwired: 3 in, 1 out]
                      n461 = GPIB Read(0:w909, 1:200, 3:w910) -> (5:w905:string)  [unwired: 2 in, 2 out]
                      n462 = Fract/Exp String To Number(string=w905) -> (number=w907:dbl)  [unwired: 3 in, 1 out]
                      n463 = Build Array (concatenate)(w912, w907) -> (w911:dbl[])
                    }
                  }
                  n464 = property on="array for data" class="Arr (strict)"("Value"=w902) -> ()  [unwired: 2 in, 2 out]
                }
                frame #22 {
                  # "check if 2nd channel\non Keithley 2182 \n(addr. 17) is to\nbe measured"
                  n465 = property on="Channel 2 (Vnano3b)" class="Bool (strict)"() -> ("Value"=w913:bool)  [unwired: 2 in, 2 out]
                  n466 = property on="array for data" class="Arr (strict)"() -> ("Value"=w915:dbl[])  [unwired: 2 in, 2 out]
                  n467 = case shown="False" w913 {
                    tunnel: w915 -> [w916 w928]
                    tunnel: [w916 w927] -> w914
                    frame False {
                      # "we are not measuring 1st channel\non Keithley 2182 (addr. 17)"
                    }
                    frame True {
                      w919 = "17"
                      # "switching to channel 2 and then\nback to channel 1"
                      # "we are measuring 2nd channel\non Keithley 2182 (addr. 17)"
                      n468 = GPIB Write(0:w919, 1:":SENSe:CHAN 2") -> (6:w920:errorcluster)  [unwired: 3 in, 1 out]
                      n469 = GPIB Write(0:w919, 1:":SENSe:DATA:FRES?", 3:w920) -> (6:w926:errorcluster)  [unwired: 2 in, 1 out]
                      n470 = GPIB Read(0:w919, 1:200, 3:w926) -> (5:w922:string, 7:w918:errorcluster)  [unwired: 2 in, 1 out]
                      n471 = GPIB Write(0:w919, 1:":SENSe:CHAN 1", 3:w918) -> ()  [unwired: 2 in, 2 out]
                      n472 = Fract/Exp String To Number(string=w922) -> (number=w924:dbl)  [unwired: 3 in, 1 out]
                      n473 = Build Array (concatenate)(w928, w924) -> (w927:dbl[])
                    }
                  }
                  n474 = property on="array for data" class="Arr (strict)"("Value"=w914) -> ()  [unwired: 2 in, 2 out]
                }
                frame #23 {
                  # "check if 1st \nthermometer on \nOxford ITC \n(address 24) \nis measured"
                  n475 = property on="Thermometer 1 (T1)" class="Bool (strict)"() -> ("Value"=w929:bool)  [unwired: 2 in, 2 out]
                  n476 = property on="array for data" class="Arr (strict)"() -> ("Value"=w931:dbl[])  [unwired: 2 in, 2 out]
                  n477 = case shown="True" w929 {
                    tunnel: w931 -> [w932 w941]
                    tunnel: [w932 w940] -> w930
                    frame False {
                      # "we are not measuring temperature on\nthermometer 1 (addr. 24)"
                    }
                    frame True {
                      w933 = 1
                      w938 = "24"
                      # "we are measuring temperature,\nthermometer 1 (addr. 24)"
                      n478 = GPIB Write(0:w938, 1:"R 1", 2:w933) -> (6:w939:errorcluster)  [unwired: 2 in, 1 out]
                      n479 = GPIB Read(0:w938, 1:200, 2:w933, 3:w939) -> (5:w934:string)  [unwired: 1 in, 2 out]
                      n480 = Fract/Exp String To Number(string=w934, offset=w933) -> (number=w936:dbl)  [unwired: 2 in, 1 out]
                      n481 = Build Array (concatenate)(w941, w936) -> (w940:dbl[])
                    }
                  }
                  n482 = property on="array for data" class="Arr (strict)"("Value"=w930) -> ()  [unwired: 2 in, 2 out]
                }
                frame #24 {
                  # "check if 1st \nthermometer on \nOxford ITC \n(address 24) \nis measured"
                  n483 = property on="Magnetic Field (B)" class="Bool (strict)"() -> ("Value"=w942:bool)  [unwired: 2 in, 2 out]
                  n484 = property on="array for data" class="Arr (strict)"() -> ("Value"=w944:dbl[])  [unwired: 2 in, 2 out]
                  n485 = case shown="True" w942 {
                    tunnel: w944 -> [w945 w954]
                    tunnel: [w945 w953] -> w943
                    frame False {
                      # "we are not measuringmagnetic field (addr. 25)"
                    }
                    frame True {
                      w946 = 1
                      w951 = "25"
                      # "we are measuring magnetic field  (addr. 25)"
                      n486 = GPIB Write(0:w951, 1:"R 7", 2:w946) -> (6:w952:errorcluster)  [unwired: 2 in, 1 out]
                      n487 = GPIB Read(0:w951, 1:200, 2:w946, 3:w952) -> (5:w947:string)  [unwired: 1 in, 2 out]
                      n488 = Fract/Exp String To Number(string=w947, offset=w946) -> (number=w949:dbl)  [unwired: 2 in, 1 out]
                      n489 = Build Array (concatenate)(w954, w949) -> (w953:dbl[])
                    }
                  }
                  n490 = property on="array for data" class="Arr (strict)"("Value"=w943) -> ()  [unwired: 2 in, 2 out]
                }
                frame #25 {
                  # "check if capacitance\nand loss (address 28)\nare measured"
                  n491 = property on="Capacitance (C) and Loss (L)" class="Bool (strict)"() -> ("Value"=w955:bool)  [unwired: 2 in, 2 out]
                  n492 = property on="array for data" class="Arr (strict)"() -> ("Value"=w957:dbl[])  [unwired: 2 in, 2 out]
                  n493 = case shown="False" w955 {
                    tunnel: w957 -> [w958 w964]
                    tunnel: [w958 w960] -> w956
                    frame False {
                      # "we are not measuringmagnetic capacitance (addr. 28)"
                    }
                    frame True {
                      # "we are measuring capacitance and loss  (addr. 28)"
                      n494 = stacked-sequence {
                        seq-local: [w966 _ _] -> [_ _ w989]
                        tunnel: [_ _ w983] -> w959
                        tunnel: [_ _ w984] -> w962
                        tunnel: "28" ("data") -> [w965 w969 w978]
                        frame #0 {
                          n495 = GPIB Write(0:w965, 1:"SINGLE" ("data"), 2:i16 0 ("mode (0)")) -> (6:w966:errorcluster)  [unwired: 2 in, 1 out]
                        }
                        frame #1 {
                          n496 = while {
                            tunnel: w969 -> [w970]
                            i -> [w971]
                            stop <- w973 continue-if-true
                            n497 = GPIB Serial Poll(0:w970) -> (2:w975:i16)  [unwired: 1 in, 2 out]
                            n498 = Less?(x=w975, y=i16 128) -> (x < y?=w973:bool)
                            n499 = Wait (ms)(milliseconds to wait=u32 50) -> ()  [unwired: 1 out]
                            "Numeric" <- w971
                          }
                        }
                        frame #2 {
                          w976 = i16 2 ("mode (0)")
                          n500 = GPIB Read(0:w978, 1:200 ("byte count"), 2:i16 2 ("mode (0)"), 3:w989) -> (5:w982:string)  [unwired: 1 in, 2 out]
                          n501 = Match Pattern(string=w982, regular expression="C=") -> (after substring=w981:string)  [unwired: 1 in, 3 out]
                          n502 = Match Pattern(string=w981, regular expression="PF L=") -> (after substring=w979:string)  [unwired: 1 in, 3 out]
                          n503 = Search/Split String(string=w981, search string/char (-)=" ", offset (0)=w976) -> (substring before match=w986:string)  [unwired: 2 out]
                          n504 = Search/Split String(string=w979, search string/char (-)=" ", offset (0)=w976) -> (substring before match=w985:string)  [unwired: 2 out]
                          n505 = Fract/Exp String To Number(string=w985) -> (number=w983:dbl)  [unwired: 3 in, 1 out]
                          n506 = Fract/Exp String To Number(string=w986) -> (number=w984:dbl)  [unwired: 3 in, 1 out]
                        }
                      }
                      n507 = Build Array (concatenate)(w964, w962) -> (w961:dbl[])
                      n508 = Build Array (concatenate)(w961, w959) -> (w960:dbl[])
                    }
                  }
                  n509 = property on="array for data" class="Arr (strict)"("Value"=w956) -> ()  [unwired: 2 in, 2 out]
                }
              }
              n510 = flat-sequence {
                tunnel: w604 -> [_]
                frame #0 {
                  n511 = property on="Delib Time delay" class="DigNum (strict)"() -> ("Value"=w620:i32)  [unwired: 2 in, 2 out]
                  n512 = Wait (ms)(milliseconds to wait=w620) -> ()  [unwired: 1 out]
                }
              }
              n513 = case shown="\"Radio Selection 2\"" "Commute SorceMeter" {
                tunnel: ["13" "14"] -> w605
                frame "Radio Selection 1", Default {
                }
                frame "Radio Selection 2" {
                }
              }
              n514 = GPIB Write(0:w605, 1:":READ?", 3:w603) -> (6:w606:errorcluster)  [unwired: 2 in, 1 out]
              n515 = GPIB Read(0:w605, 1:3200, 3:w606) -> (5:w609:string)  [unwired: 2 in, 2 out]
              n516 = String Subset(string=w609, length (rest)=13) -> (substring=w610:string)  [unwired: 1 in]
              n517 = Fract/Exp String To Number(string=w610) -> (number=w612:dbl)  [unwired: 3 in, 1 out]
              n518 = Multiply(x=w612, y=-1.0) -> (x*y=w617:dbl)
              n519 = Number To Fractional String(number=w617) -> (F-format string=w614:string)  [unwired: 3 in]
              n520 = Concatenate Strings(":INIT:IMM; :SOUR:VOLT:LEV:IMM:AMPL " ("data"), w614) -> (w615:string)
              n521 = GPIB Write(0:w605, 1:w615) -> (6:w604:errorcluster)  [unwired: 3 in, 1 out]
            }
            frame #1 {
              n522 = stacked-sequence {
                tunnel: w1008 -> [w1011 _ _ _ _ _ _ _ _ _ _ _ _ _ _ _ _ _ _ _ _ _ _ _ _ _]
                tunnel: [w1011 _ _ _ _ _ _ _ _ _ _ _ _ _ _ _ _ _ _ _ _ _ _ _ _ _] -> w994
                frame #0 {
                  # "check if oscillator on \nlock-in (address 1)\nis to be measured"
                  n523 = property on="Current is:" class="RadioBtnsControl (strict)"() -> ("Value"=w1014:T1)  [unwired: 2 in, 2 out]
                  n524 = property on="array for data" class="Arr (strict)"() -> ("Value"=w1013:dbl[])  [unwired: 2 in, 2 out]
                  n525 = Equal?(x=w1014, y=1) -> (x = y?=w1015:bool)
                  n526 = case shown="False" w1015 {
                    tunnel: w1013 -> [w1017 w1025]
                    tunnel: [w1017 w1024] -> w1012
                    frame False {
                      # "we are not measuring oscillator from\nlock-in (address 1)"
                    }
                    frame True {
                      w1021 = "1"
                      # "we are  measuring oscillator"
                      n527 = GPIB Write(0:w1021, 1:"SLVL?") -> (6:w1022:errorcluster)  [unwired: 3 in, 1 out]
                      n528 = GPIB Read(0:w1021, 1:3200, 3:w1022) -> (5:w1019:string)  [unwired: 2 in, 2 out]
                      n529 = Fract/Exp String To Number(string=w1019) -> (number=w1018:dbl)  [unwired: 3 in, 1 out]
                      n530 = Build Array (concatenate)(w1025, w1018) -> (w1024:dbl[])
                    }
                  }
                  n531 = property on="array for data" class="Arr (strict)"("Value"=w1012) -> ()  [unwired: 2 in, 2 out]
                }
                frame #1 {
                  # "check if in-phase\nsignal on lock-in \n(address 1) is to\nbe measured"
                  n532 = property on="array for data" class="Arr (strict)"() -> ("Value"=w1028:dbl[])  [unwired: 2 in, 2 out]
                  n533 = property on="Addr 1 lock-in" class="Bool (strict)"() -> ("Value"=w1026:bool)  [unwired: 2 in, 2 out]
                  n534 = case shown="True" w1026 {
                    tunnel: w1028 -> [w1029 w1037]
                    tunnel: [w1029 w1036] -> w1027
                    frame False {
                      # "we are not measuring in phase signal on lock-in (address 1)"
                    }
                    frame True {
                      w1034 = "1"
                      # "we are  measuring lock-in (address 1), in phase"
                      n535 = GPIB Write(0:w1034, 1:"OUTP?1") -> (6:w1035:errorcluster)  [unwired: 3 in, 1 out]
                      n536 = GPIB Read(0:w1034, 1:3200, 3:w1035) -> (5:w1032:string)  [unwired: 2 in, 2 out]
                      n537 = Fract/Exp String To Number(string=w1032) -> (number=w1031:dbl)  [unwired: 3 in, 1 out]
                      n538 = Build Array (concatenate)(w1037, w1031) -> (w1036:dbl[])
                    }
                  }
                  n539 = property on="array for data" class="Arr (strict)"("Value"=w1027) -> ()  [unwired: 2 in, 2 out]
                }
                frame #2 {
                  # "check if out-of-phase\nsignal on lock-in \n(address 1) is to\nbe measured"
                  n540 = property on="Addr 1 lock-in oop" class="Bool (strict)"() -> ("Value"=w1038:bool)  [unwired: 2 in, 2 out]
                  n541 = property on="array for data" class="Arr (strict)"() -> ("Value"=w1040:dbl[])  [unwired: 2 in, 2 out]
                  n542 = case shown="True" w1038 {
                    tunnel: w1040 -> [w1041 w1049]
                    tunnel: [w1041 w1048] -> w1039
                    frame False {
                      # "we are not measuring out-of-phase signal on lock-in (address 1)"
                    }
                    frame True {
                      w1046 = "1"
                      # "we are  measuring lock-in (address 1), out-of-phase signal"
                      n543 = GPIB Write(0:w1046, 1:"OUTP?2") -> (6:w1047:errorcluster)  [unwired: 3 in, 1 out]
                      n544 = GPIB Read(0:w1046, 1:3200, 3:w1047) -> (5:w1044:string)  [unwired: 2 in, 2 out]
                      n545 = Fract/Exp String To Number(string=w1044) -> (number=w1043:dbl)  [unwired: 3 in, 1 out]
                      n546 = Build Array (concatenate)(w1049, w1043) -> (w1048:dbl[])
                    }
                  }
                  n547 = property on="array for data" class="Arr (strict)"("Value"=w1039) -> ()  [unwired: 2 in, 2 out]
                }
                frame #3 {
                  # "check if in-phase\nsignal on lock-in \n(address 2) is to\nbe measured"
                  n548 = property on="Addr 2 lock-in" class="Bool (strict)"() -> ("Value"=w1050:bool)  [unwired: 2 in, 2 out]
                  n549 = property on="array for data" class="Arr (strict)"() -> ("Value"=w1052:dbl[])  [unwired: 2 in, 2 out]
                  n550 = case shown="False" w1050 {
                    tunnel: w1052 -> [w1053 w1061]
                    tunnel: [w1053 w1060] -> w1051
                    frame False {
                      # "we are not measuring in phase signal on lock-in (address 2)"
                    }
                    frame True {
                      w1058 = "2"
                      # "we are  measuring lock-in (address 2), in phase"
                      n551 = GPIB Write(0:w1058, 1:"OUTP?1") -> (6:w1059:errorcluster)  [unwired: 3 in, 1 out]
                      n552 = GPIB Read(0:w1058, 1:3200, 3:w1059) -> (5:w1056:string)  [unwired: 2 in, 2 out]
                      n553 = Fract/Exp String To Number(string=w1056) -> (number=w1055:dbl)  [unwired: 3 in, 1 out]
                      n554 = Build Array (concatenate)(w1061, w1055) -> (w1060:dbl[])
                    }
                  }
                  n555 = property on="array for data" class="Arr (strict)"("Value"=w1051) -> ()  [unwired: 2 in, 2 out]
                }
                frame #4 {
                  # "check if out-of-phase\nsignal on lock-in \n(address 2) is to\nbe measured"
                  n556 = property on="Addr 2 lock-in oop" class="Bool (strict)"() -> ("Value"=w1062:bool)  [unwired: 2 in, 2 out]
                  n557 = property on="array for data" class="Arr (strict)"() -> ("Value"=w1064:dbl[])  [unwired: 2 in, 2 out]
                  n558 = case shown="False" w1062 {
                    tunnel: w1064 -> [w1065 w1073]
                    tunnel: [w1065 w1072] -> w1063
                    tunnel: w1062 -> [_ _]
                    frame False {
                      # "we are not measuring out-of-phase signal on lock-in (address 2)"
                    }
                    frame True {
                      w1070 = "2"
                      # "we are  measuring lock-in (address 2), out-of-phase"
                      n559 = GPIB Write(0:w1070, 1:"OUTP?2") -> (6:w1071:errorcluster)  [unwired: 3 in, 1 out]
                      n560 = GPIB Read(0:w1070, 1:3200, 3:w1071) -> (5:w1068:string)  [unwired: 2 in, 2 out]
                      n561 = Fract/Exp String To Number(string=w1068) -> (number=w1067:dbl)  [unwired: 3 in, 1 out]
                      n562 = Build Array (concatenate)(w1073, w1067) -> (w1072:dbl[])
                    }
                  }
                  n563 = property on="array for data" class="Arr (strict)"("Value"=w1063) -> ()  [unwired: 2 in, 2 out]
                }
                frame #5 {
                  # "check if in-phase\nsignal on lock-in \n(address 3) is to\nbe measured"
                  n564 = property on="Addr 3 lock-in" class="Bool (strict)"() -> ("Value"=w1074:bool)  [unwired: 2 in, 2 out]
                  n565 = property on="array for data" class="Arr (strict)"() -> ("Value"=w1076:dbl[])  [unwired: 2 in, 2 out]
                  n566 = case shown="True" w1074 {
                    tunnel: w1076 -> [w1077 w1085]
                    tunnel: [w1077 w1084] -> w1075
                    frame False {
                      # "we are not measuring in phase signal on lock-in (address 3)"
                    }
                    frame True {
                      w1082 = "3"
                      # "we are  measuring lock-in (address 3), in phase"
                      n567 = GPIB Write(0:w1082, 1:"OUTP?1") -> (6:w1083:errorcluster)  [unwired: 3 in, 1 out]
                      n568 = GPIB Read(0:w1082, 1:3200, 3:w1083) -> (5:w1080:string)  [unwired: 2 in, 2 out]
                      n569 = Fract/Exp String To Number(string=w1080) -> (number=w1079:dbl)  [unwired: 3 in, 1 out]
                      n570 = Build Array (concatenate)(w1085, w1079) -> (w1084:dbl[])
                    }
                  }
                  n571 = property on="array for data" class="Arr (strict)"("Value"=w1075) -> ()  [unwired: 2 in, 2 out]
                }
                frame #6 {
                  # "check if out-of-phase\nsignal on lock-in \n(address 3) is to\nbe measured"
                  n572 = property on="Addr 3 lock-in oop" class="Bool (strict)"() -> ("Value"=w1086:bool)  [unwired: 2 in, 2 out]
                  n573 = property on="array for data" class="Arr (strict)"() -> ("Value"=w1088:dbl[])  [unwired: 2 in, 2 out]
                  n574 = case shown="True" w1086 {
                    tunnel: w1088 -> [w1089 w1097]
                    tunnel: [w1089 w1096] -> w1087
                    frame False {
                      # "we are not measuring out-of-phase signal on lock-in (address 3)"
                    }
                    frame True {
                      w1094 = "3"
                      # "we are  measuring lock-in (address 3), out-of-phase"
                      n575 = GPIB Write(0:w1094, 1:"OUTP?2") -> (6:w1095:errorcluster)  [unwired: 3 in, 1 out]
                      n576 = GPIB Read(0:w1094, 1:3200, 3:w1095) -> (5:w1092:string)  [unwired: 2 in, 2 out]
                      n577 = Fract/Exp String To Number(string=w1092) -> (number=w1091:dbl)  [unwired: 3 in, 1 out]
                      n578 = Build Array (concatenate)(w1097, w1091) -> (w1096:dbl[])
                    }
                  }
                  n579 = property on="array for data" class="Arr (strict)"("Value"=w1087) -> ()  [unwired: 2 in, 2 out]
                }
                frame #7 {
                  # "check if in-phase\nsignal on lock-in \n(address 4) is to\nbe measured"
                  n580 = property on="Addr 4 lock-in" class="Bool (strict)"() -> ("Value"=w1098:bool)  [unwired: 2 in, 2 out]
                  n581 = property on="array for data" class="Arr (strict)"() -> ("Value"=w1100:dbl[])  [unwired: 2 in, 2 out]
                  n582 = case shown="True" w1098 {
                    tunnel: w1100 -> [w1101 w1109]
                    tunnel: [w1101 w1108] -> w1099
                    frame False {
                      # "we are not measuring in phase signal on lock-in (address 4)"
                    }
                    frame True {
                      w1106 = "4"
                      # "we are  measuring lock-in (address 4), in phase"
                      n583 = GPIB Write(0:w1106, 1:"OUTP?1") -> (6:w1107:errorcluster)  [unwired: 3 in, 1 out]
                      n584 = GPIB Read(0:w1106, 1:3200, 3:w1107) -> (5:w1104:string)  [unwired: 2 in, 2 out]
                      n585 = Fract/Exp String To Number(string=w1104) -> (number=w1103:dbl)  [unwired: 3 in, 1 out]
                      n586 = Build Array (concatenate)(w1109, w1103) -> (w1108:dbl[])
                    }
                  }
                  n587 = property on="array for data" class="Arr (strict)"("Value"=w1099) -> ()  [unwired: 2 in, 2 out]
                }
                frame #8 {
                  # "check if out-of-phase\nsignal on lock-in \n(address 4) is to\nbe measured"
                  n588 = property on="Addr 4 lock-in oop" class="Bool (strict)"() -> ("Value"=w1110:bool)  [unwired: 2 in, 2 out]
                  n589 = property on="array for data" class="Arr (strict)"() -> ("Value"=w1112:dbl[])  [unwired: 2 in, 2 out]
                  n590 = case shown="True" w1110 {
                    tunnel: w1112 -> [w1113 w1121]
                    tunnel: [w1113 w1120] -> w1111
                    frame False {
                      # "we are not measuring out-of-phase signal on lock-in (address 4)"
                    }
                    frame True {
                      w1118 = "4"
                      # "we are  measuring lock-in (address 4), out-of-phase"
                      n591 = GPIB Write(0:w1118, 1:"OUTP?2") -> (6:w1119:errorcluster)  [unwired: 3 in, 1 out]
                      n592 = GPIB Read(0:w1118, 1:3200, 3:w1119) -> (5:w1116:string)  [unwired: 2 in, 2 out]
                      n593 = Fract/Exp String To Number(string=w1116) -> (number=w1115:dbl)  [unwired: 3 in, 1 out]
                      n594 = Build Array (concatenate)(w1121, w1115) -> (w1120:dbl[])
                    }
                  }
                  n595 = property on="array for data" class="Arr (strict)"("Value"=w1111) -> ()  [unwired: 2 in, 2 out]
                }
                frame #9 {
                  # "check if in-phase\nsignal on lock-in \n(address 5) is to\nbe measured"
                  n596 = property on="Addr 5 lock-in" class="Bool (strict)"() -> ("Value"=w1122:bool)  [unwired: 2 in, 2 out]
                  n597 = property on="array for data" class="Arr (strict)"() -> ("Value"=w1124:dbl[])  [unwired: 2 in, 2 out]
                  n598 = case shown="False" w1122 {
                    tunnel: w1124 -> [w1125 w1133]
                    tunnel: [w1125 w1132] -> w1123
                    frame False {
                      # "we are not measuring in phase signal on lock-in (address 5)"
                    }
                    frame True {
                      w1130 = "5"
                      # "we are  measuring lock-in (address 5), in phase"
                      n599 = GPIB Write(0:w1130, 1:"OUTP?1") -> (6:w1131:errorcluster)  [unwired: 3 in, 1 out]
                      n600 = GPIB Read(0:w1130, 1:3200, 3:w1131) -> (5:w1128:string)  [unwired: 2 in, 2 out]
                      n601 = Fract/Exp String To Number(string=w1128) -> (number=w1127:dbl)  [unwired: 3 in, 1 out]
                      n602 = Build Array (concatenate)(w1133, w1127) -> (w1132:dbl[])
                    }
                  }
                  n603 = property on="array for data" class="Arr (strict)"("Value"=w1123) -> ()  [unwired: 2 in, 2 out]
                }
                frame #10 {
                  # "check if out-of-phase\nsignal on lock-in \n(address 5) is to\nbe measured"
                  n604 = property on="Addr 5 lock-in oop" class="Bool (strict)"() -> ("Value"=w1134:bool)  [unwired: 2 in, 2 out]
                  n605 = property on="array for data" class="Arr (strict)"() -> ("Value"=w1136:dbl[])  [unwired: 2 in, 2 out]
                  n606 = case shown="False" w1134 {
                    tunnel: w1136 -> [w1137 w1145]
                    tunnel: [w1137 w1144] -> w1135
                    frame False {
                      # "we are not measuring out-of-phase signal on lock-in (address 5)"
                    }
                    frame True {
                      w1142 = "5"
                      # "we are  measuring lock-in (address 5), out-of-phase"
                      n607 = GPIB Write(0:w1142, 1:"OUTP?2") -> (6:w1143:errorcluster)  [unwired: 3 in, 1 out]
                      n608 = GPIB Read(0:w1142, 1:3200, 3:w1143) -> (5:w1140:string)  [unwired: 2 in, 2 out]
                      n609 = Fract/Exp String To Number(string=w1140) -> (number=w1139:dbl)  [unwired: 3 in, 1 out]
                      n610 = Build Array (concatenate)(w1145, w1139) -> (w1144:dbl[])
                    }
                  }
                  n611 = property on="array for data" class="Arr (strict)"("Value"=w1135) -> ()  [unwired: 2 in, 2 out]
                }
                frame #11 {
                  # "check if voltage on \nmain Keithley 2400 \n(addr. 12) is to\nbe measured"
                  n612 = property on="Voltage (Vk1)" class="Bool (strict)"() -> ("Value"=w1146:bool)  [unwired: 2 in, 2 out]
                  n613 = property on="array for data" class="Arr (strict)"() -> ("Value"=w1148:dbl[])  [unwired: 2 in, 2 out]
                  n614 = case shown="False" w1146 {
                    tunnel: w1148 -> [w1149 w1159]
                    tunnel: [w1149 w1158] -> w1147
                    frame False {
                      # "we aren't measuring voltage \non main Keithley 2400 (addr. 12)"
                    }
                    frame True {
                      w1156 = "12"
                      # "we are measuring voltage \non main Keithley 2400 (addr. 12)"
                      n615 = GPIB Write(0:w1156, 1:":READ?") -> (6:w1157:errorcluster)  [unwired: 3 in, 1 out]
                      n616 = GPIB Read(0:w1156, 1:3200, 3:w1157) -> (5:w1152:string)  [unwired: 2 in, 2 out]
                      n617 = String Subset(string=w1152, length (rest)=13) -> (substring=w1151:string)  [unwired: 1 in]
                      n618 = Fract/Exp String To Number(string=w1151) -> (number=w1154:dbl)  [unwired: 3 in, 1 out]
                      n619 = Build Array (concatenate)(w1159, w1154) -> (w1158:dbl[])
                    }
                  }
                  n620 = property on="array for data" class="Arr (strict)"("Value"=w1147) -> ()  [unwired: 2 in, 2 out]
                }
                frame #12 {
                  # "check if  current on \nmain Keithley 2400 \n(addr. 12) is to\nbe measured"
                  n621 = property on="Current (Ik1)" class="Bool (strict)"() -> ("Value"=w1160:bool)  [unwired: 2 in, 2 out]
                  n622 = property on="array for data" class="Arr (strict)"() -> ("Value"=w1162:dbl[])  [unwired: 2 in, 2 out]
                  n623 = case shown="True" w1160 {
                    tunnel: w1162 -> [w1163 w1174]
                    tunnel: [w1163 w1173] -> w1161
                    frame False {
                      # "we aren't measuring current \non main Keithley 2400 (addr. 12)"
                    }
                    frame True {
                      w1171 = "12"
                      # "we are measuring current\non main Keithley 2400 (addr. 12)"
                      n624 = GPIB Write(0:w1171, 1:":READ?") -> (6:w1172:errorcluster)  [unwired: 3 in, 1 out]
                      n625 = GPIB Read(0:w1171, 1:3200, 3:w1172) -> (5:w1167:string)  [unwired: 2 in, 2 out]
                      n626 = String Subset(string=w1167, offset (0)=14, length (rest)=13) -> (substring=w1166:string)
                      n627 = Fract/Exp String To Number(string=w1166) -> (number=w1169:dbl)  [unwired: 3 in, 1 out]
                      n628 = Build Array (concatenate)(w1174, w1169) -> (w1173:dbl[])
                    }
                  }
                  n629 = property on="array for data" class="Arr (strict)"("Value"=w1161) -> ()  [unwired: 2 in, 2 out]
                }
                frame #13 {
                  # "check if voltage on \nadd. Keithley 2400 \n(addr. 13) is to\nbe measured"
                  n630 = property on="Voltage (Vk2)" class="Bool (strict)"() -> ("Value"=w1175:bool)  [unwired: 2 in, 2 out]
                  n631 = property on="array for data" class="Arr (strict)"() -> ("Value"=w1177:dbl[])  [unwired: 2 in, 2 out]
                  n632 = case shown="True" w1175 {
                    tunnel: w1177 -> [w1178 w1188]
                    tunnel: [w1178 w1187] -> w1176
                    frame False {
                      # "we aren't measuring voltage \non additional Keithley 2400 (addr. 13)"
                    }
                    frame True {
                      w1185 = "13"
                      # "we are measuring voltage \non additional Keithley 2400 (addr. 13)"
                      n633 = GPIB Write(0:w1185, 1:":READ?") -> (6:w1186:errorcluster)  [unwired: 3 in, 1 out]
                      n634 = GPIB Read(0:w1185, 1:3200, 3:w1186) -> (5:w1181:string)  [unwired: 2 in, 2 out]
                      n635 = String Subset(string=w1181, length (rest)=13) -> (substring=w1180:string)  [unwired: 1 in]
                      n636 = Fract/Exp String To Number(string=w1180) -> (number=w1183:dbl)  [unwired: 3 in, 1 out]
                      n637 = Build Array (concatenate)(w1188, w1183) -> (w1187:dbl[])
                    }
                  }
                  n638 = property on="array for data" class="Arr (strict)"("Value"=w1176) -> ()  [unwired: 2 in, 2 out]
                }
                frame #14 {
                  # "check if  current on \nadd. Keithley 2400 \n(addr. 13) is to\nbe measured"
                  n639 = property on="Current (Ik2)" class="Bool (strict)"() -> ("Value"=w1189:bool)  [unwired: 2 in, 2 out]
                  n640 = property on="array for data" class="Arr (strict)"() -> ("Value"=w1191:dbl[])  [unwired: 2 in, 2 out]
                  n641 = case shown="True" w1189 {
                    tunnel: w1191 -> [w1192 w1203]
                    tunnel: [w1192 w1202] -> w1190
                    frame False {
                      # "we aren't measuring current \non additional Keithley 2400 (addr. 13)"
                    }
                    frame True {
                      w1200 = "13"
                      # "we are measuring current\non additional Keithley 2400 (addr. 13)"
                      n642 = GPIB Write(0:w1200, 1:":READ?") -> (6:w1201:errorcluster)  [unwired: 3 in, 1 out]
                      n643 = GPIB Read(0:w1200, 1:3200, 3:w1201) -> (5:w1196:string)  [unwired: 2 in, 2 out]
                      n644 = String Subset(string=w1196, offset (0)=14, length (rest)=13) -> (substring=w1195:string)
                      n645 = Fract/Exp String To Number(string=w1195) -> (number=w1198:dbl)  [unwired: 3 in, 1 out]
                      n646 = Build Array (concatenate)(w1203, w1198) -> (w1202:dbl[])
                    }
                  }
                  n647 = property on="array for data" class="Arr (strict)"("Value"=w1190) -> ()  [unwired: 2 in, 2 out]
                }
                frame #15 {
                  # "check if voltage on \nadd. Keithley 2400 \n(addr. 14) is to\nbe measured"
                  n648 = property on="Voltage (Vk3)" class="Bool (strict)"() -> ("Value"=w1204:bool)  [unwired: 2 in, 2 out]
                  n649 = property on="array for data" class="Arr (strict)"() -> ("Value"=w1206:dbl[])  [unwired: 2 in, 2 out]
                  n650 = case shown="False" w1204 {
                    tunnel: w1206 -> [w1207 w1217]
                    tunnel: [w1207 w1216] -> w1205
                    frame False {
                      # "we aren't measuring voltage \non additional Keithley 2400 (addr. 14)"
                    }
                    frame True {
                      w1214 = "14"
                      # "we are measuring voltage \non additional Keithley 2400 (addr. 14)"
                      n651 = GPIB Write(0:w1214, 1:":READ?") -> (6:w1215:errorcluster)  [unwired: 3 in, 1 out]
                      n652 = GPIB Read(0:w1214, 1:3200, 3:w1215) -> (5:w1210:string)  [unwired: 2 in, 2 out]
                      n653 = String Subset(string=w1210, length (rest)=13) -> (substring=w1209:string)  [unwired: 1 in]
                      n654 = Fract/Exp String To Number(string=w1209) -> (number=w1212:dbl)  [unwired: 3 in, 1 out]
                      n655 = Build Array (concatenate)(w1217, w1212) -> (w1216:dbl[])
                    }
                  }
                  n656 = property on="array for data" class="Arr (strict)"("Value"=w1205) -> ()  [unwired: 2 in, 2 out]
                }
                frame #16 {
                  # "check if  current on \nadd. Keithley 2400 \n(addr. 14) is to\nbe measured"
                  n657 = property on="Current (Ik3)" class="Bool (strict)"() -> ("Value"=w1218:bool)  [unwired: 2 in, 2 out]
                  n658 = property on="array for data" class="Arr (strict)"() -> ("Value"=w1220:dbl[])  [unwired: 2 in, 2 out]
                  n659 = case shown="True" w1218 {
                    tunnel: w1220 -> [w1221 w1232]
                    tunnel: [w1221 w1231] -> w1219
                    frame False {
                      # "we aren't measuring current \non additional Keithley 2400 (addr. 14)"
                    }
                    frame True {
                      w1229 = "14"
                      # "we are measuring current\non additional Keithley 2400 (addr. 14)"
                      n660 = GPIB Write(0:w1229, 1:":READ?") -> (6:w1230:errorcluster)  [unwired: 3 in, 1 out]
                      n661 = GPIB Read(0:w1229, 1:3200, 3:w1230) -> (5:w1225:string)  [unwired: 2 in, 2 out]
                      n662 = String Subset(string=w1225, offset (0)=14, length (rest)=13) -> (substring=w1224:string)
                      n663 = Fract/Exp String To Number(string=w1224) -> (number=w1227:dbl)  [unwired: 3 in, 1 out]
                      n664 = Build Array (concatenate)(w1232, w1227) -> (w1231:dbl[])
                    }
                  }
                  n665 = property on="array for data" class="Arr (strict)"("Value"=w1219) -> ()  [unwired: 2 in, 2 out]
                }
                frame #17 {
                  # "check if 1st channel\non Keithley 2182 \n(addr. 15) is to\nbe measured"
                  n666 = property on="Channel 1 (Vnano1)" class="Bool (strict)"() -> ("Value"=w1233:bool)  [unwired: 2 in, 2 out]
                  n667 = property on="array for data" class="Arr (strict)"() -> ("Value"=w1235:dbl[])  [unwired: 2 in, 2 out]
                  n668 = case shown="True" w1233 {
                    tunnel: w1235 -> [w1236 w1244]
                    tunnel: [w1236 w1243] -> w1234
                    frame False {
                      # "we are not measuring 1st channel\non Keithley 2182 (addr. 15)"
                    }
                    frame True {
                      w1241 = "15"
                      # "we are measuring 1st channel\non Keithley 2182 (addr. 15)"
                      n669 = GPIB Write(0:w1241, 1:":SENSe:DATA:FRES?") -> (6:w1242:errorcluster)  [unwired: 3 in, 1 out]
                      n670 = GPIB Read(0:w1241, 1:200, 3:w1242) -> (5:w1237:string)  [unwired: 2 in, 2 out]
                      n671 = Fract/Exp String To Number(string=w1237) -> (number=w1239:dbl)  [unwired: 3 in, 1 out]
                      n672 = Build Array (concatenate)(w1244, w1239) -> (w1243:dbl[])
                    }
                  }
                  n673 = property on="array for data" class="Arr (strict)"("Value"=w1234) -> ()  [unwired: 2 in, 2 out]
                }
                frame #18 {
                  # "check if 2nd channel\non Keithley 2182 \n(addr. 15) is to\nbe measured"
                  n674 = property on="Channel 2 (Vnano1b)" class="Bool (strict)"() -> ("Value"=w1245:bool)  [unwired: 2 in, 2 out]
                  n675 = property on="array for data" class="Arr (strict)"() -> ("Value"=w1247:dbl[])  [unwired: 2 in, 2 out]
                  n676 = case shown="False" w1245 {
                    tunnel: w1247 -> [w1248 w1260]
                    tunnel: [w1248 w1259] -> w1246
                    frame False {
                      # "we are not measuring 1st channel\non Keithley 2182 (addr. 15)"
                    }
                    frame True {
                      w1251 = "15"
                      # "switching to channel 2 and then\nback to channel 1"
                      # "we are measuring 2nd channel\non Keithley 2182 (addr. 15)"
                      n677 = GPIB Write(0:w1251, 1:":SENSe:CHAN 2") -> (6:w1252:errorcluster)  [unwired: 3 in, 1 out]
                      n678 = GPIB Write(0:w1251, 1:":SENSe:DATA:FRES?", 3:w1252) -> (6:w1258:errorcluster)  [unwired: 2 in, 1 out]
                      n679 = GPIB Read(0:w1251, 1:200, 3:w1258) -> (5:w1254:string, 7:w1250:errorcluster)  [unwired: 2 in, 1 out]
                      n680 = GPIB Write(0:w1251, 1:":SENSe:CHAN 1", 3:w1250) -> ()  [unwired: 2 in, 2 out]
                      n681 = Fract/Exp String To Number(string=w1254) -> (number=w1256:dbl)  [unwired: 3 in, 1 out]
                      n682 = Build Array (concatenate)(w1260, w1256) -> (w1259:dbl[])
                    }
                  }
                  n683 = property on="array for data" class="Arr (strict)"("Value"=w1246) -> ()  [unwired: 2 in, 2 out]
                }
                frame #19 {
                  # "check if 1st channel\non Keithley 2182 \n(addr. 16) is to\nbe measured"
                  n684 = property on="Channel 1 (Vnano2)" class="Bool (strict)"() -> ("Value"=w1261:bool)  [unwired: 2 in, 2 out]
                  n685 = property on="array for data" class="Arr (strict)"() -> ("Value"=w1263:dbl[])  [unwired: 2 in, 2 out]
                  n686 = case shown="True" w1261 {
                    tunnel: w1263 -> [w1264 w1272]
                    tunnel: [w1264 w1271] -> w1262
                    frame False {
                      # "we are not measuring 1st channel\non Keithley 2182 (addr. 16)"
                    }
                    frame True {
                      w1269 = "16"
                      # "we are measuring 1st channel\non Keithley 2182 (addr. 16)"
                      n687 = GPIB Write(0:w1269, 1:":SENSe:DATA:FRES?") -> (6:w1270:errorcluster)  [unwired: 3 in, 1 out]
                      n688 = GPIB Read(0:w1269, 1:200, 3:w1270) -> (5:w1265:string)  [unwired: 2 in, 2 out]
                      n689 = Fract/Exp String To Number(string=w1265) -> (number=w1267:dbl)  [unwired: 3 in, 1 out]
                      n690 = Build Array (concatenate)(w1272, w1267) -> (w1271:dbl[])
                    }
                  }
                  n691 = property on="array for data" class="Arr (strict)"("Value"=w1262) -> ()  [unwired: 2 in, 2 out]
                }
                frame #20 {
                  # "check if 2nd channel\non Keithley 2182 \n(addr. 16) is to\nbe measured"
                  n692 = property on="Channel 2 (Vnano2b)" class="Bool (strict)"() -> ("Value"=w1273:bool)  [unwired: 2 in, 2 out]
                  n693 = property on="array for data" class="Arr (strict)"() -> ("Value"=w1275:dbl[])  [unwired: 2 in, 2 out]
                  n694 = case shown="True" w1273 {
                    tunnel: w1275 -> [w1276 w1288]
                    tunnel: [w1276 w1287] -> w1274
                    frame False {
                      # "we are not measuring 1st channel\non Keithley 2182 (addr. 16)"
                    }
                    frame True {
                      w1279 = "16"
                      # "switching to channel 2 and then\nback to channel 1"
                      # "we are measuring 2nd channel\non Keithley 2182 (addr. 16)"
                      n695 = GPIB Write(0:w1279, 1:":SENSe:CHAN 2") -> (6:w1280:errorcluster)  [unwired: 3 in, 1 out]
                      n696 = GPIB Write(0:w1279, 1:":SENSe:DATA:FRES?", 3:w1280) -> (6:w1286:errorcluster)  [unwired: 2 in, 1 out]
                      n697 = GPIB Read(0:w1279, 1:200, 3:w1286) -> (5:w1282:string, 7:w1278:errorcluster)  [unwired: 2 in, 1 out]
                      n698 = GPIB Write(0:w1279, 1:":SENSe:CHAN 1", 3:w1278) -> ()  [unwired: 2 in, 2 out]
                      n699 = Fract/Exp String To Number(string=w1282) -> (number=w1284:dbl)  [unwired: 3 in, 1 out]
                      n700 = Build Array (concatenate)(w1288, w1284) -> (w1287:dbl[])
                    }
                  }
                  n701 = property on="array for data" class="Arr (strict)"("Value"=w1274) -> ()  [unwired: 2 in, 2 out]
                }
                frame #21 {
                  # "check if 1st channel\non Keithley 2182 \n(addr. 17) is to\nbe measured"
                  n702 = property on="Channel 1 (Vnano3)" class="Bool (strict)"() -> ("Value"=w1289:bool)  [unwired: 2 in, 2 out]
                  n703 = property on="array for data" class="Arr (strict)"() -> ("Value"=w1291:dbl[])  [unwired: 2 in, 2 out]
                  n704 = case shown="True" w1289 {
                    tunnel: w1291 -> [w1292 w1300]
                    tunnel: [w1292 w1299] -> w1290
                    frame False {
                      # "we are not measuring 1st channel\non Keithley 2182 (addr. 17)"
                    }
                    frame True {
                      w1297 = "17"
                      # "we are measuring 1st channel\non Keithley 2182 (addr. 17)"
                      n705 = GPIB Write(0:w1297, 1:":SENSe:DATA:FRES?") -> (6:w1298:errorcluster)  [unwired: 3 in, 1 out]
                      n706 = GPIB Read(0:w1297, 1:200, 3:w1298) -> (5:w1293:string)  [unwired: 2 in, 2 out]
                      n707 = Fract/Exp String To Number(string=w1293) -> (number=w1295:dbl)  [unwired: 3 in, 1 out]
                      n708 = Build Array (concatenate)(w1300, w1295) -> (w1299:dbl[])
                    }
                  }
                  n709 = property on="array for data" class="Arr (strict)"("Value"=w1290) -> ()  [unwired: 2 in, 2 out]
                }
                frame #22 {
                  # "check if 2nd channel\non Keithley 2182 \n(addr. 17) is to\nbe measured"
                  n710 = property on="Channel 2 (Vnano3b)" class="Bool (strict)"() -> ("Value"=w1301:bool)  [unwired: 2 in, 2 out]
                  n711 = property on="array for data" class="Arr (strict)"() -> ("Value"=w1303:dbl[])  [unwired: 2 in, 2 out]
                  n712 = case shown="True" w1301 {
                    tunnel: w1303 -> [w1304 w1316]
                    tunnel: [w1304 w1315] -> w1302
                    frame False {
                      # "we are not measuring 1st channel\non Keithley 2182 (addr. 17)"
                    }
                    frame True {
                      w1307 = "17"
                      # "switching to channel 2 and then\nback to channel 1"
                      # "we are measuring 2nd channel\non Keithley 2182 (addr. 17)"
                      n713 = GPIB Write(0:w1307, 1:":SENSe:CHAN 2") -> (6:w1308:errorcluster)  [unwired: 3 in, 1 out]
                      n714 = GPIB Write(0:w1307, 1:":SENSe:DATA:FRES?", 3:w1308) -> (6:w1314:errorcluster)  [unwired: 2 in, 1 out]
                      n715 = GPIB Read(0:w1307, 1:200, 3:w1314) -> (5:w1310:string, 7:w1306:errorcluster)  [unwired: 2 in, 1 out]
                      n716 = GPIB Write(0:w1307, 1:":SENSe:CHAN 1", 3:w1306) -> ()  [unwired: 2 in, 2 out]
                      n717 = Fract/Exp String To Number(string=w1310) -> (number=w1312:dbl)  [unwired: 3 in, 1 out]
                      n718 = Build Array (concatenate)(w1316, w1312) -> (w1315:dbl[])
                    }
                  }
                  n719 = property on="array for data" class="Arr (strict)"("Value"=w1302) -> ()  [unwired: 2 in, 2 out]
                }
                frame #23 {
                  # "check if 1st \nthermometer on \nOxford ITC \n(address 24) \nis measured"
                  n720 = property on="Thermometer 1 (T1)" class="Bool (strict)"() -> ("Value"=w1317:bool)  [unwired: 2 in, 2 out]
                  n721 = property on="array for data" class="Arr (strict)"() -> ("Value"=w1319:dbl[])  [unwired: 2 in, 2 out]
                  n722 = case shown="True" w1317 {
                    tunnel: w1319 -> [w1320 w1329]
                    tunnel: [w1320 w1328] -> w1318
                    frame False {
                      # "we are not measuring temperature on\nthermometer 1 (addr. 24)"
                    }
                    frame True {
                      w1321 = 1
                      w1326 = "24"
                      # "we are measuring temperature,\nthermometer 1 (addr. 24)"
                      n723 = GPIB Write(0:w1326, 1:"R 1", 2:w1321) -> (6:w1327:errorcluster)  [unwired: 2 in, 1 out]
                      n724 = GPIB Read(0:w1326, 1:200, 2:w1321, 3:w1327) -> (5:w1322:string)  [unwired: 1 in, 2 out]
                      n725 = Fract/Exp String To Number(string=w1322, offset=w1321) -> (number=w1324:dbl)  [unwired: 2 in, 1 out]
                      n726 = Build Array (concatenate)(w1329, w1324) -> (w1328:dbl[])
                    }
                  }
                  n727 = property on="array for data" class="Arr (strict)"("Value"=w1318) -> ()  [unwired: 2 in, 2 out]
                }
                frame #24 {
                  # "check if 1st \nthermometer on \nOxford ITC \n(address 24) \nis measured"
                  n728 = property on="Magnetic Field (B)" class="Bool (strict)"() -> ("Value"=w1330:bool)  [unwired: 2 in, 2 out]
                  n729 = property on="array for data" class="Arr (strict)"() -> ("Value"=w1332:dbl[])  [unwired: 2 in, 2 out]
                  n730 = case shown="True" w1330 {
                    tunnel: w1332 -> [w1333 w1342]
                    tunnel: [w1333 w1341] -> w1331
                    frame False {
                      # "we are not measuringmagnetic field (addr. 25)"
                    }
                    frame True {
                      w1334 = 1
                      w1339 = "25"
                      # "we are measuring magnetic field  (addr. 25)"
                      n731 = GPIB Write(0:w1339, 1:"R 8", 2:w1334) -> (6:w1340:errorcluster)  [unwired: 2 in, 1 out]
                      n732 = GPIB Read(0:w1339, 1:200, 2:w1334, 3:w1340) -> (5:w1335:string)  [unwired: 1 in, 2 out]
                      n733 = Fract/Exp String To Number(string=w1335, offset=w1334) -> (number=w1337:dbl)  [unwired: 2 in, 1 out]
                      n734 = Build Array (concatenate)(w1342, w1337) -> (w1341:dbl[])
                    }
                  }
                  n735 = property on="array for data" class="Arr (strict)"("Value"=w1331) -> ()  [unwired: 2 in, 2 out]
                }
                frame #25 {
                  # "check if capacitance\nand loss (address 28)\nare measured"
                  n736 = property on="Capacitance (C) and Loss (L)" class="Bool (strict)"() -> ("Value"=w1343:bool)  [unwired: 2 in, 2 out]
                  n737 = property on="array for data" class="Arr (strict)"() -> ("Value"=w1345:dbl[])  [unwired: 2 in, 2 out]
                  n738 = case shown="True" w1343 {
                    tunnel: w1345 -> [w1346 w1352]
                    tunnel: [w1346 w1348] -> w1344
                    frame False {
                      # "we are not measuringmagnetic capacitance (addr. 28)"
                    }
                    frame True {
                      # "we are measuring capacitance and loss  (addr. 28)"
                      n739 = stacked-sequence {
                        seq-local: [w1354 _ _] -> [_ _ w1377]
                        tunnel: [_ _ w1371] -> w1347
                        tunnel: [_ _ w1372] -> w1350
                        tunnel: "28" ("data") -> [w1353 w1357 w1366]
                        frame #0 {
                          n740 = GPIB Write(0:w1353, 1:"SINGLE" ("data"), 2:i16 0 ("mode (0)")) -> (6:w1354:errorcluster)  [unwired: 2 in, 1 out]
                        }
                        frame #1 {
                          n741 = while {
                            tunnel: w1357 -> [w1358]
                            i -> [w1359]
                            stop <- w1361 continue-if-true
                            n742 = GPIB Serial Poll(0:w1358) -> (2:w1363:i16)  [unwired: 1 in, 2 out]
                            n743 = Less?(x=w1363, y=i16 128) -> (x < y?=w1361:bool)
                            n744 = Wait (ms)(milliseconds to wait=u32 50) -> ()  [unwired: 1 out]
                            "Numeric 4" <- w1359
                          }
                        }
                        frame #2 {
                          w1364 = i16 2 ("mode (0)")
                          n745 = GPIB Read(0:w1366, 1:200 ("byte count"), 2:i16 2 ("mode (0)"), 3:w1377) -> (5:w1370:string)  [unwired: 1 in, 2 out]
                          n746 = Match Pattern(string=w1370, regular expression="C=") -> (after substring=w1369:string)  [unwired: 1 in, 3 out]
                          n747 = Match Pattern(string=w1369, regular expression="PF L=") -> (after substring=w1367:string)  [unwired: 1 in, 3 out]
                          n748 = Search/Split String(string=w1369, search string/char (-)=" ", offset (0)=w1364) -> (substring before match=w1374:string)  [unwired: 2 out]
                          n749 = Search/Split String(string=w1367, search string/char (-)=" ", offset (0)=w1364) -> (substring before match=w1373:string)  [unwired: 2 out]
                          n750 = Fract/Exp String To Number(string=w1373) -> (number=w1371:dbl)  [unwired: 3 in, 1 out]
                          n751 = Fract/Exp String To Number(string=w1374) -> (number=w1372:dbl)  [unwired: 3 in, 1 out]
                        }
                      }
                      n752 = Build Array (concatenate)(w1352, w1350) -> (w1349:dbl[])
                      n753 = Build Array (concatenate)(w1349, w1347) -> (w1348:dbl[])
                    }
                  }
                  n754 = property on="array for data" class="Arr (strict)"("Value"=w1344) -> ()  [unwired: 2 in, 2 out]
                }
              }
              n755 = property on="Commute SorceMeter" class="RadioBtnsControl (strict)"() -> ("Value"=w992:enum32{"Radio Selection 1", "Radio Selection 2"})  [unwired: 2 in, 2 out]
              n756 = case shown="\"Radio Selection 1\", Default" w992 {
                tunnel: ["13" "14"] -> w995
                frame "Radio Selection 1", Default {
                }
                frame "Radio Selection 2" {
                }
              }
              n757 = GPIB Write(0:w995, 1:":READ?", 3:w994) -> (6:w996:errorcluster)  [unwired: 2 in, 1 out]
              n758 = GPIB Read(0:w995, 1:3200, 3:w996) -> (5:w999:string)  [unwired: 2 in, 2 out]
              n759 = String Subset(string=w999, length (rest)=13) -> (substring=w1000:string)  [unwired: 1 in]
              n760 = Fract/Exp String To Number(string=w1000) -> (number=w1002:dbl)  [unwired: 3 in, 1 out]
              n761 = Multiply(x=w1002, y=-1.0) -> (x*y=w1007:dbl)
              n762 = Number To Fractional String(number=w1007) -> (F-format string=w1004:string)  [unwired: 3 in]
              n763 = Concatenate Strings(":INIT:IMM; :SOUR:VOLT:LEV:IMM:AMPL " ("data"), w1004) -> (w1005:string)
              n764 = GPIB Write(0:w995, 1:w1005) -> (6:w993:errorcluster)  [unwired: 3 in, 1 out]
            }
          }
        }
        frame False {
          # "all measurements are done in this stacked sequence; reading from each device is recorded to \"array for data\""
          n765 = stacked-sequence {
            tunnel: w1380 -> [w1382 _ _ _ _ _ _ _ _ _ _ _ _ _ _ _ _ _ _ _ _ _ _ _ _ _]
            tunnel: [w1382 _ _ _ _ _ _ _ _ _ _ _ _ _ _ _ _ _ _ _ _ _ _ _ _ _] -> w1381
            frame #0 {
              # "check if oscillator on \nlock-in (address 1)\nis to be measured"
              n766 = property on="Current is:" class="RadioBtnsControl (strict)"() -> ("Value"=w1385:T1)  [unwired: 2 in, 2 out]
              n767 = property on="array for data" class="Arr (strict)"() -> ("Value"=w1384:dbl[])  [unwired: 2 in, 2 out]
              n768 = Equal?(x=w1385, y=1) -> (x = y?=w1386:bool)
              n769 = case shown="False" w1386 {
                tunnel: w1384 -> [w1388 w1396]
                tunnel: [w1388 w1395] -> w1383
                frame False {
                  # "we are not measuring oscillator from\nlock-in (address 1)"
                }
                frame True {
                  w1392 = "1"
                  # "we are  measuring oscillator"
                  n770 = GPIB Write(0:w1392, 1:"SLVL?") -> (6:w1393:errorcluster)  [unwired: 3 in, 1 out]
                  n771 = GPIB Read(0:w1392, 1:3200, 3:w1393) -> (5:w1390:string)  [unwired: 2 in, 2 out]
                  n772 = Fract/Exp String To Number(string=w1390) -> (number=w1389:dbl)  [unwired: 3 in, 1 out]
                  n773 = Build Array (concatenate)(w1396, w1389) -> (w1395:dbl[])
                }
              }
              n774 = property on="array for data" class="Arr (strict)"("Value"=w1383) -> ()  [unwired: 2 in, 2 out]
            }
            frame #1 {
              # "check if in-phase\nsignal on lock-in \n(address 1) is to\nbe measured"
              n775 = property on="array for data" class="Arr (strict)"() -> ("Value"=w1399:dbl[])  [unwired: 2 in, 2 out]
              n776 = property on="Addr 1 lock-in" class="Bool (strict)"() -> ("Value"=w1397:bool)  [unwired: 2 in, 2 out]
              n777 = case shown="False" w1397 {
                tunnel: w1399 -> [w1400 w1408]
                tunnel: [w1400 w1407] -> w1398
                frame False {
                  # "we are not measuring in phase signal on lock-in (address 1)"
                }
                frame True {
                  w1405 = "1"
                  # "we are  measuring lock-in (address 1), in phase"
                  n778 = GPIB Write(0:w1405, 1:"OUTP?1") -> (6:w1406:errorcluster)  [unwired: 3 in, 1 out]
                  n779 = GPIB Read(0:w1405, 1:3200, 3:w1406) -> (5:w1403:string)  [unwired: 2 in, 2 out]
                  n780 = Fract/Exp String To Number(string=w1403) -> (number=w1402:dbl)  [unwired: 3 in, 1 out]
                  n781 = Build Array (concatenate)(w1408, w1402) -> (w1407:dbl[])
                }
              }
              n782 = property on="array for data" class="Arr (strict)"("Value"=w1398) -> ()  [unwired: 2 in, 2 out]
            }
            frame #2 {
              # "check if out-of-phase\nsignal on lock-in \n(address 1) is to\nbe measured"
              n783 = property on="Addr 1 lock-in oop" class="Bool (strict)"() -> ("Value"=w1409:bool)  [unwired: 2 in, 2 out]
              n784 = property on="array for data" class="Arr (strict)"() -> ("Value"=w1411:dbl[])  [unwired: 2 in, 2 out]
              n785 = case shown="False" w1409 {
                tunnel: w1411 -> [w1412 w1420]
                tunnel: [w1412 w1419] -> w1410
                frame False {
                  # "we are not measuring out-of-phase signal on lock-in (address 1)"
                }
                frame True {
                  w1417 = "1"
                  # "we are  measuring lock-in (address 1), out-of-phase signal"
                  n786 = GPIB Write(0:w1417, 1:"OUTP?2") -> (6:w1418:errorcluster)  [unwired: 3 in, 1 out]
                  n787 = GPIB Read(0:w1417, 1:3200, 3:w1418) -> (5:w1415:string)  [unwired: 2 in, 2 out]
                  n788 = Fract/Exp String To Number(string=w1415) -> (number=w1414:dbl)  [unwired: 3 in, 1 out]
                  n789 = Build Array (concatenate)(w1420, w1414) -> (w1419:dbl[])
                }
              }
              n790 = property on="array for data" class="Arr (strict)"("Value"=w1410) -> ()  [unwired: 2 in, 2 out]
            }
            frame #3 {
              # "check if in-phase\nsignal on lock-in \n(address 2) is to\nbe measured"
              n791 = property on="Addr 2 lock-in" class="Bool (strict)"() -> ("Value"=w1421:bool)  [unwired: 2 in, 2 out]
              n792 = property on="array for data" class="Arr (strict)"() -> ("Value"=w1423:dbl[])  [unwired: 2 in, 2 out]
              n793 = case shown="False" w1421 {
                tunnel: w1423 -> [w1424 w1432]
                tunnel: [w1424 w1431] -> w1422
                frame False {
                  # "we are not measuring in phase signal on lock-in (address 2)"
                }
                frame True {
                  w1429 = "2"
                  # "we are  measuring lock-in (address 2), in phase"
                  n794 = GPIB Write(0:w1429, 1:"OUTP?1") -> (6:w1430:errorcluster)  [unwired: 3 in, 1 out]
                  n795 = GPIB Read(0:w1429, 1:3200, 3:w1430) -> (5:w1427:string)  [unwired: 2 in, 2 out]
                  n796 = Fract/Exp String To Number(string=w1427) -> (number=w1426:dbl)  [unwired: 3 in, 1 out]
                  n797 = Build Array (concatenate)(w1432, w1426) -> (w1431:dbl[])
                }
              }
              n798 = property on="array for data" class="Arr (strict)"("Value"=w1422) -> ()  [unwired: 2 in, 2 out]
            }
            frame #4 {
              # "check if out-of-phase\nsignal on lock-in \n(address 2) is to\nbe measured"
              n799 = property on="Addr 2 lock-in oop" class="Bool (strict)"() -> ("Value"=w1433:bool)  [unwired: 2 in, 2 out]
              n800 = property on="array for data" class="Arr (strict)"() -> ("Value"=w1435:dbl[])  [unwired: 2 in, 2 out]
              n801 = case shown="False" w1433 {
                tunnel: w1435 -> [w1436 w1444]
                tunnel: [w1436 w1443] -> w1434
                tunnel: w1433 -> [_ _]
                frame False {
                  # "we are not measuring out-of-phase signal on lock-in (address 2)"
                }
                frame True {
                  w1441 = "2"
                  # "we are  measuring lock-in (address 2), out-of-phase"
                  n802 = GPIB Write(0:w1441, 1:"OUTP?2") -> (6:w1442:errorcluster)  [unwired: 3 in, 1 out]
                  n803 = GPIB Read(0:w1441, 1:3200, 3:w1442) -> (5:w1439:string)  [unwired: 2 in, 2 out]
                  n804 = Fract/Exp String To Number(string=w1439) -> (number=w1438:dbl)  [unwired: 3 in, 1 out]
                  n805 = Build Array (concatenate)(w1444, w1438) -> (w1443:dbl[])
                }
              }
              n806 = property on="array for data" class="Arr (strict)"("Value"=w1434) -> ()  [unwired: 2 in, 2 out]
            }
            frame #5 {
              # "check if in-phase\nsignal on lock-in \n(address 3) is to\nbe measured"
              n807 = property on="Addr 3 lock-in" class="Bool (strict)"() -> ("Value"=w1445:bool)  [unwired: 2 in, 2 out]
              n808 = property on="array for data" class="Arr (strict)"() -> ("Value"=w1447:dbl[])  [unwired: 2 in, 2 out]
              n809 = case shown="False" w1445 {
                tunnel: w1447 -> [w1448 w1456]
                tunnel: [w1448 w1455] -> w1446
                frame False {
                  # "we are not measuring in phase signal on lock-in (address 3)"
                }
                frame True {
                  w1453 = "3"
                  # "we are  measuring lock-in (address 3), in phase"
                  n810 = GPIB Write(0:w1453, 1:"OUTP?1") -> (6:w1454:errorcluster)  [unwired: 3 in, 1 out]
                  n811 = GPIB Read(0:w1453, 1:3200, 3:w1454) -> (5:w1451:string)  [unwired: 2 in, 2 out]
                  n812 = Fract/Exp String To Number(string=w1451) -> (number=w1450:dbl)  [unwired: 3 in, 1 out]
                  n813 = Build Array (concatenate)(w1456, w1450) -> (w1455:dbl[])
                }
              }
              n814 = property on="array for data" class="Arr (strict)"("Value"=w1446) -> ()  [unwired: 2 in, 2 out]
            }
            frame #6 {
              # "check if out-of-phase\nsignal on lock-in \n(address 3) is to\nbe measured"
              n815 = property on="Addr 3 lock-in oop" class="Bool (strict)"() -> ("Value"=w1457:bool)  [unwired: 2 in, 2 out]
              n816 = property on="array for data" class="Arr (strict)"() -> ("Value"=w1459:dbl[])  [unwired: 2 in, 2 out]
              n817 = case shown="False" w1457 {
                tunnel: w1459 -> [w1460 w1468]
                tunnel: [w1460 w1467] -> w1458
                frame False {
                  # "we are not measuring out-of-phase signal on lock-in (address 3)"
                }
                frame True {
                  w1465 = "3"
                  # "we are  measuring lock-in (address 3), out-of-phase"
                  n818 = GPIB Write(0:w1465, 1:"OUTP?2") -> (6:w1466:errorcluster)  [unwired: 3 in, 1 out]
                  n819 = GPIB Read(0:w1465, 1:3200, 3:w1466) -> (5:w1463:string)  [unwired: 2 in, 2 out]
                  n820 = Fract/Exp String To Number(string=w1463) -> (number=w1462:dbl)  [unwired: 3 in, 1 out]
                  n821 = Build Array (concatenate)(w1468, w1462) -> (w1467:dbl[])
                }
              }
              n822 = property on="array for data" class="Arr (strict)"("Value"=w1458) -> ()  [unwired: 2 in, 2 out]
            }
            frame #7 {
              # "check if in-phase\nsignal on lock-in \n(address 4) is to\nbe measured"
              n823 = property on="Addr 4 lock-in" class="Bool (strict)"() -> ("Value"=w1469:bool)  [unwired: 2 in, 2 out]
              n824 = property on="array for data" class="Arr (strict)"() -> ("Value"=w1471:dbl[])  [unwired: 2 in, 2 out]
              n825 = case shown="False" w1469 {
                tunnel: w1471 -> [w1472 w1480]
                tunnel: [w1472 w1479] -> w1470
                frame False {
                  # "we are not measuring in phase signal on lock-in (address 4)"
                }
                frame True {
                  w1477 = "4"
                  # "we are  measuring lock-in (address 4), in phase"
                  n826 = GPIB Write(0:w1477, 1:"OUTP?1") -> (6:w1478:errorcluster)  [unwired: 3 in, 1 out]
                  n827 = GPIB Read(0:w1477, 1:3200, 3:w1478) -> (5:w1475:string)  [unwired: 2 in, 2 out]
                  n828 = Fract/Exp String To Number(string=w1475) -> (number=w1474:dbl)  [unwired: 3 in, 1 out]
                  n829 = Build Array (concatenate)(w1480, w1474) -> (w1479:dbl[])
                }
              }
              n830 = property on="array for data" class="Arr (strict)"("Value"=w1470) -> ()  [unwired: 2 in, 2 out]
            }
            frame #8 {
              # "check if out-of-phase\nsignal on lock-in \n(address 4) is to\nbe measured"
              n831 = property on="Addr 4 lock-in oop" class="Bool (strict)"() -> ("Value"=w1481:bool)  [unwired: 2 in, 2 out]
              n832 = property on="array for data" class="Arr (strict)"() -> ("Value"=w1483:dbl[])  [unwired: 2 in, 2 out]
              n833 = case shown="False" w1481 {
                tunnel: w1483 -> [w1484 w1492]
                tunnel: [w1484 w1491] -> w1482
                frame False {
                  # "we are not measuring out-of-phase signal on lock-in (address 4)"
                }
                frame True {
                  w1489 = "4"
                  # "we are  measuring lock-in (address 4), out-of-phase"
                  n834 = GPIB Write(0:w1489, 1:"OUTP?2") -> (6:w1490:errorcluster)  [unwired: 3 in, 1 out]
                  n835 = GPIB Read(0:w1489, 1:3200, 3:w1490) -> (5:w1487:string)  [unwired: 2 in, 2 out]
                  n836 = Fract/Exp String To Number(string=w1487) -> (number=w1486:dbl)  [unwired: 3 in, 1 out]
                  n837 = Build Array (concatenate)(w1492, w1486) -> (w1491:dbl[])
                }
              }
              n838 = property on="array for data" class="Arr (strict)"("Value"=w1482) -> ()  [unwired: 2 in, 2 out]
            }
            frame #9 {
              # "check if in-phase\nsignal on lock-in \n(address 5) is to\nbe measured"
              n839 = property on="Addr 5 lock-in" class="Bool (strict)"() -> ("Value"=w1493:bool)  [unwired: 2 in, 2 out]
              n840 = property on="array for data" class="Arr (strict)"() -> ("Value"=w1495:dbl[])  [unwired: 2 in, 2 out]
              n841 = case shown="False" w1493 {
                tunnel: w1495 -> [w1496 w1504]
                tunnel: [w1496 w1503] -> w1494
                frame False {
                  # "we are not measuring in phase signal on lock-in (address 5)"
                }
                frame True {
                  w1501 = "5"
                  # "we are  measuring lock-in (address 5), in phase"
                  n842 = GPIB Write(0:w1501, 1:"OUTP?1") -> (6:w1502:errorcluster)  [unwired: 3 in, 1 out]
                  n843 = GPIB Read(0:w1501, 1:3200, 3:w1502) -> (5:w1499:string)  [unwired: 2 in, 2 out]
                  n844 = Fract/Exp String To Number(string=w1499) -> (number=w1498:dbl)  [unwired: 3 in, 1 out]
                  n845 = Build Array (concatenate)(w1504, w1498) -> (w1503:dbl[])
                }
              }
              n846 = property on="array for data" class="Arr (strict)"("Value"=w1494) -> ()  [unwired: 2 in, 2 out]
            }
            frame #10 {
              # "check if out-of-phase\nsignal on lock-in \n(address 5) is to\nbe measured"
              n847 = property on="Addr 5 lock-in oop" class="Bool (strict)"() -> ("Value"=w1505:bool)  [unwired: 2 in, 2 out]
              n848 = property on="array for data" class="Arr (strict)"() -> ("Value"=w1507:dbl[])  [unwired: 2 in, 2 out]
              n849 = case shown="False" w1505 {
                tunnel: w1507 -> [w1508 w1516]
                tunnel: [w1508 w1515] -> w1506
                frame False {
                  # "we are not measuring out-of-phase signal on lock-in (address 5)"
                }
                frame True {
                  w1513 = "5"
                  # "we are  measuring lock-in (address 5), out-of-phase"
                  n850 = GPIB Write(0:w1513, 1:"OUTP?2") -> (6:w1514:errorcluster)  [unwired: 3 in, 1 out]
                  n851 = GPIB Read(0:w1513, 1:3200, 3:w1514) -> (5:w1511:string)  [unwired: 2 in, 2 out]
                  n852 = Fract/Exp String To Number(string=w1511) -> (number=w1510:dbl)  [unwired: 3 in, 1 out]
                  n853 = Build Array (concatenate)(w1516, w1510) -> (w1515:dbl[])
                }
              }
              n854 = property on="array for data" class="Arr (strict)"("Value"=w1506) -> ()  [unwired: 2 in, 2 out]
            }
            frame #11 {
              # "check if voltage on \nmain Keithley 2400 \n(addr. 12) is to\nbe measured"
              n855 = property on="Voltage (Vk1)" class="Bool (strict)"() -> ("Value"=w1517:bool)  [unwired: 2 in, 2 out]
              n856 = property on="array for data" class="Arr (strict)"() -> ("Value"=w1519:dbl[])  [unwired: 2 in, 2 out]
              n857 = case shown="False" w1517 {
                tunnel: w1519 -> [w1520 w1530]
                tunnel: [w1520 w1529] -> w1518
                frame False {
                  # "we aren't measuring voltage \non main Keithley 2400 (addr. 12)"
                }
                frame True {
                  w1527 = "12"
                  # "we are measuring voltage \non main Keithley 2400 (addr. 12)"
                  n858 = GPIB Write(0:w1527, 1:":READ?") -> (6:w1528:errorcluster)  [unwired: 3 in, 1 out]
                  n859 = GPIB Read(0:w1527, 1:3200, 3:w1528) -> (5:w1523:string)  [unwired: 2 in, 2 out]
                  n860 = String Subset(string=w1523, length (rest)=13) -> (substring=w1522:string)  [unwired: 1 in]
                  n861 = Fract/Exp String To Number(string=w1522) -> (number=w1525:dbl)  [unwired: 3 in, 1 out]
                  n862 = Build Array (concatenate)(w1530, w1525) -> (w1529:dbl[])
                }
              }
              n863 = property on="array for data" class="Arr (strict)"("Value"=w1518) -> ()  [unwired: 2 in, 2 out]
            }
            frame #12 {
              # "check if  current on \nmain Keithley 2400 \n(addr. 12) is to\nbe measured"
              n864 = property on="Current (Ik1)" class="Bool (strict)"() -> ("Value"=w1531:bool)  [unwired: 2 in, 2 out]
              n865 = property on="array for data" class="Arr (strict)"() -> ("Value"=w1533:dbl[])  [unwired: 2 in, 2 out]
              n866 = case shown="True" w1531 {
                tunnel: w1533 -> [w1534 w1545]
                tunnel: [w1534 w1544] -> w1532
                frame False {
                  # "we aren't measuring current \non main Keithley 2400 (addr. 12)"
                }
                frame True {
                  w1542 = "12"
                  # "we are measuring current\non main Keithley 2400 (addr. 12)"
                  n867 = GPIB Write(0:w1542, 1:":READ?") -> (6:w1543:errorcluster)  [unwired: 3 in, 1 out]
                  n868 = GPIB Read(0:w1542, 1:3200, 3:w1543) -> (5:w1538:string)  [unwired: 2 in, 2 out]
                  n869 = String Subset(string=w1538, offset (0)=14, length (rest)=13) -> (substring=w1537:string)
                  n870 = Fract/Exp String To Number(string=w1537) -> (number=w1540:dbl)  [unwired: 3 in, 1 out]
                  n871 = Build Array (concatenate)(w1545, w1540) -> (w1544:dbl[])
                }
              }
              n872 = property on="array for data" class="Arr (strict)"("Value"=w1532) -> ()  [unwired: 2 in, 2 out]
            }
            frame #13 {
              # "check if voltage on \nadd. Keithley 2400 \n(addr. 13) is to\nbe measured"
              n873 = property on="Voltage (Vk2)" class="Bool (strict)"() -> ("Value"=w1546:bool)  [unwired: 2 in, 2 out]
              n874 = property on="array for data" class="Arr (strict)"() -> ("Value"=w1548:dbl[])  [unwired: 2 in, 2 out]
              n875 = case shown="True" w1546 {
                tunnel: w1548 -> [w1549 w1559]
                tunnel: [w1549 w1558] -> w1547
                frame False {
                  # "we aren't measuring voltage \non additional Keithley 2400 (addr. 13)"
                }
                frame True {
                  w1556 = "13"
                  # "we are measuring voltage \non additional Keithley 2400 (addr. 13)"
                  n876 = GPIB Write(0:w1556, 1:":READ?") -> (6:w1557:errorcluster)  [unwired: 3 in, 1 out]
                  n877 = GPIB Read(0:w1556, 1:3200, 3:w1557) -> (5:w1552:string)  [unwired: 2 in, 2 out]
                  n878 = String Subset(string=w1552, length (rest)=13) -> (substring=w1551:string)  [unwired: 1 in]
                  n879 = Fract/Exp String To Number(string=w1551) -> (number=w1554:dbl)  [unwired: 3 in, 1 out]
                  n880 = Build Array (concatenate)(w1559, w1554) -> (w1558:dbl[])
                }
              }
              n881 = property on="array for data" class="Arr (strict)"("Value"=w1547) -> ()  [unwired: 2 in, 2 out]
            }
            frame #14 {
              # "check if  current on \nadd. Keithley 2400 \n(addr. 13) is to\nbe measured"
              n882 = property on="Current (Ik2)" class="Bool (strict)"() -> ("Value"=w1560:bool)  [unwired: 2 in, 2 out]
              n883 = property on="array for data" class="Arr (strict)"() -> ("Value"=w1562:dbl[])  [unwired: 2 in, 2 out]
              n884 = case shown="False" w1560 {
                tunnel: w1562 -> [w1563 w1574]
                tunnel: [w1563 w1573] -> w1561
                frame False {
                  # "we aren't measuring current \non additional Keithley 2400 (addr. 13)"
                }
                frame True {
                  w1571 = "13"
                  # "we are measuring current\non additional Keithley 2400 (addr. 13)"
                  n885 = GPIB Write(0:w1571, 1:":READ?") -> (6:w1572:errorcluster)  [unwired: 3 in, 1 out]
                  n886 = GPIB Read(0:w1571, 1:3200, 3:w1572) -> (5:w1567:string)  [unwired: 2 in, 2 out]
                  n887 = String Subset(string=w1567, offset (0)=14, length (rest)=13) -> (substring=w1566:string)
                  n888 = Fract/Exp String To Number(string=w1566) -> (number=w1569:dbl)  [unwired: 3 in, 1 out]
                  n889 = Build Array (concatenate)(w1574, w1569) -> (w1573:dbl[])
                }
              }
              n890 = property on="array for data" class="Arr (strict)"("Value"=w1561) -> ()  [unwired: 2 in, 2 out]
            }
            frame #15 {
              # "check if voltage on \nadd. Keithley 2400 \n(addr. 14) is to\nbe measured"
              n891 = property on="Voltage (Vk3)" class="Bool (strict)"() -> ("Value"=w1575:bool)  [unwired: 2 in, 2 out]
              n892 = property on="array for data" class="Arr (strict)"() -> ("Value"=w1577:dbl[])  [unwired: 2 in, 2 out]
              n893 = case shown="False" w1575 {
                tunnel: w1577 -> [w1578 w1588]
                tunnel: [w1578 w1587] -> w1576
                frame False {
                  # "we aren't measuring voltage \non additional Keithley 2400 (addr. 14)"
                }
                frame True {
                  w1585 = "14"
                  # "we are measuring voltage \non additional Keithley 2400 (addr. 14)"
                  n894 = GPIB Write(0:w1585, 1:":READ?") -> (6:w1586:errorcluster)  [unwired: 3 in, 1 out]
                  n895 = GPIB Read(0:w1585, 1:3200, 3:w1586) -> (5:w1581:string)  [unwired: 2 in, 2 out]
                  n896 = String Subset(string=w1581, length (rest)=13) -> (substring=w1580:string)  [unwired: 1 in]
                  n897 = Fract/Exp String To Number(string=w1580) -> (number=w1583:dbl)  [unwired: 3 in, 1 out]
                  n898 = Build Array (concatenate)(w1588, w1583) -> (w1587:dbl[])
                }
              }
              n899 = property on="array for data" class="Arr (strict)"("Value"=w1576) -> ()  [unwired: 2 in, 2 out]
            }
            frame #16 {
              # "check if  current on \nadd. Keithley 2400 \n(addr. 14) is to\nbe measured"
              n900 = property on="Current (Ik3)" class="Bool (strict)"() -> ("Value"=w1589:bool)  [unwired: 2 in, 2 out]
              n901 = property on="array for data" class="Arr (strict)"() -> ("Value"=w1591:dbl[])  [unwired: 2 in, 2 out]
              n902 = case shown="True" w1589 {
                tunnel: w1591 -> [w1592 w1603]
                tunnel: [w1592 w1602] -> w1590
                frame False {
                  # "we aren't measuring current \non additional Keithley 2400 (addr. 14)"
                }
                frame True {
                  w1600 = "14"
                  # "we are measuring current\non additional Keithley 2400 (addr. 14)"
                  n903 = GPIB Write(0:w1600, 1:":READ?") -> (6:w1601:errorcluster)  [unwired: 3 in, 1 out]
                  n904 = GPIB Read(0:w1600, 1:3200, 3:w1601) -> (5:w1596:string)  [unwired: 2 in, 2 out]
                  n905 = String Subset(string=w1596, offset (0)=14, length (rest)=13) -> (substring=w1595:string)
                  n906 = Fract/Exp String To Number(string=w1595) -> (number=w1598:dbl)  [unwired: 3 in, 1 out]
                  n907 = Build Array (concatenate)(w1603, w1598) -> (w1602:dbl[])
                }
              }
              n908 = property on="array for data" class="Arr (strict)"("Value"=w1590) -> ()  [unwired: 2 in, 2 out]
            }
            frame #17 {
              # "check if 1st channel\non Keithley 2182 \n(addr. 15) is to\nbe measured"
              n909 = property on="Channel 1 (Vnano1)" class="Bool (strict)"() -> ("Value"=w1604:bool)  [unwired: 2 in, 2 out]
              n910 = property on="array for data" class="Arr (strict)"() -> ("Value"=w1606:dbl[])  [unwired: 2 in, 2 out]
              n911 = case shown="True" w1604 {
                tunnel: w1606 -> [w1607 w1615]
                tunnel: [w1607 w1614] -> w1605
                frame False {
                  # "we are not measuring 1st channel\non Keithley 2182 (addr. 15)"
                }
                frame True {
                  w1612 = "15"
                  # "we are measuring 1st channel\non Keithley 2182 (addr. 15)"
                  n912 = GPIB Write(0:w1612, 1:":SENSe:DATA:FRES?") -> (6:w1613:errorcluster)  [unwired: 3 in, 1 out]
                  n913 = GPIB Read(0:w1612, 1:200, 3:w1613) -> (5:w1608:string)  [unwired: 2 in, 2 out]
                  n914 = Fract/Exp String To Number(string=w1608) -> (number=w1610:dbl)  [unwired: 3 in, 1 out]
                  n915 = Build Array (concatenate)(w1615, w1610) -> (w1614:dbl[])
                }
              }
              n916 = property on="array for data" class="Arr (strict)"("Value"=w1605) -> ()  [unwired: 2 in, 2 out]
            }
            frame #18 {
              # "check if 2nd channel\non Keithley 2182 \n(addr. 15) is to\nbe measured"
              n917 = property on="Channel 2 (Vnano1b)" class="Bool (strict)"() -> ("Value"=w1616:bool)  [unwired: 2 in, 2 out]
              n918 = property on="array for data" class="Arr (strict)"() -> ("Value"=w1618:dbl[])  [unwired: 2 in, 2 out]
              n919 = case shown="False" w1616 {
                tunnel: w1618 -> [w1619 w1631]
                tunnel: [w1619 w1630] -> w1617
                frame False {
                  # "we are not measuring 1st channel\non Keithley 2182 (addr. 15)"
                }
                frame True {
                  w1622 = "15"
                  # "switching to channel 2 and then\nback to channel 1"
                  # "we are measuring 2nd channel\non Keithley 2182 (addr. 15)"
                  n920 = GPIB Write(0:w1622, 1:":SENSe:CHAN 2") -> (6:w1623:errorcluster)  [unwired: 3 in, 1 out]
                  n921 = GPIB Write(0:w1622, 1:":SENSe:DATA:FRES?", 3:w1623) -> (6:w1629:errorcluster)  [unwired: 2 in, 1 out]
                  n922 = GPIB Read(0:w1622, 1:200, 3:w1629) -> (5:w1625:string, 7:w1621:errorcluster)  [unwired: 2 in, 1 out]
                  n923 = GPIB Write(0:w1622, 1:":SENSe:CHAN 1", 3:w1621) -> ()  [unwired: 2 in, 2 out]
                  n924 = Fract/Exp String To Number(string=w1625) -> (number=w1627:dbl)  [unwired: 3 in, 1 out]
                  n925 = Build Array (concatenate)(w1631, w1627) -> (w1630:dbl[])
                }
              }
              n926 = property on="array for data" class="Arr (strict)"("Value"=w1617) -> ()  [unwired: 2 in, 2 out]
            }
            frame #19 {
              # "check if 1st channel\non Keithley 2182 \n(addr. 16) is to\nbe measured"
              n927 = property on="Channel 1 (Vnano2)" class="Bool (strict)"() -> ("Value"=w1632:bool)  [unwired: 2 in, 2 out]
              n928 = property on="array for data" class="Arr (strict)"() -> ("Value"=w1634:dbl[])  [unwired: 2 in, 2 out]
              n929 = case shown="True" w1632 {
                tunnel: w1634 -> [w1635 w1643]
                tunnel: [w1635 w1642] -> w1633
                frame False {
                  # "we are not measuring 1st channel\non Keithley 2182 (addr. 16)"
                }
                frame True {
                  w1640 = "16"
                  # "we are measuring 1st channel\non Keithley 2182 (addr. 16)"
                  n930 = GPIB Write(0:w1640, 1:":SENSe:DATA:FRES?") -> (6:w1641:errorcluster)  [unwired: 3 in, 1 out]
                  n931 = GPIB Read(0:w1640, 1:200, 3:w1641) -> (5:w1636:string)  [unwired: 2 in, 2 out]
                  n932 = Fract/Exp String To Number(string=w1636) -> (number=w1638:dbl)  [unwired: 3 in, 1 out]
                  n933 = Build Array (concatenate)(w1643, w1638) -> (w1642:dbl[])
                }
              }
              n934 = property on="array for data" class="Arr (strict)"("Value"=w1633) -> ()  [unwired: 2 in, 2 out]
            }
            frame #20 {
              # "check if 2nd channel\non Keithley 2182 \n(addr. 16) is to\nbe measured"
              n935 = property on="Channel 2 (Vnano2b)" class="Bool (strict)"() -> ("Value"=w1644:bool)  [unwired: 2 in, 2 out]
              n936 = property on="array for data" class="Arr (strict)"() -> ("Value"=w1646:dbl[])  [unwired: 2 in, 2 out]
              n937 = case shown="False" w1644 {
                tunnel: w1646 -> [w1647 w1659]
                tunnel: [w1647 w1658] -> w1645
                frame False {
                  # "we are not measuring 1st channel\non Keithley 2182 (addr. 16)"
                }
                frame True {
                  w1650 = "16"
                  # "switching to channel 2 and then\nback to channel 1"
                  # "we are measuring 2nd channel\non Keithley 2182 (addr. 16)"
                  n938 = GPIB Write(0:w1650, 1:":SENSe:CHAN 2") -> (6:w1651:errorcluster)  [unwired: 3 in, 1 out]
                  n939 = GPIB Write(0:w1650, 1:":SENSe:DATA:FRES?", 3:w1651) -> (6:w1657:errorcluster)  [unwired: 2 in, 1 out]
                  n940 = GPIB Read(0:w1650, 1:200, 3:w1657) -> (5:w1653:string, 7:w1649:errorcluster)  [unwired: 2 in, 1 out]
                  n941 = GPIB Write(0:w1650, 1:":SENSe:CHAN 1", 3:w1649) -> ()  [unwired: 2 in, 2 out]
                  n942 = Fract/Exp String To Number(string=w1653) -> (number=w1655:dbl)  [unwired: 3 in, 1 out]
                  n943 = Build Array (concatenate)(w1659, w1655) -> (w1658:dbl[])
                }
              }
              n944 = property on="array for data" class="Arr (strict)"("Value"=w1645) -> ()  [unwired: 2 in, 2 out]
            }
            frame #21 {
              # "check if 1st channel\non Keithley 2182 \n(addr. 17) is to\nbe measured"
              n945 = property on="Channel 1 (Vnano3)" class="Bool (strict)"() -> ("Value"=w1660:bool)  [unwired: 2 in, 2 out]
              n946 = property on="array for data" class="Arr (strict)"() -> ("Value"=w1662:dbl[])  [unwired: 2 in, 2 out]
              n947 = case shown="False" w1660 {
                tunnel: w1662 -> [w1663 w1671]
                tunnel: [w1663 w1670] -> w1661
                frame False {
                  # "we are not measuring 1st channel\non Keithley 2182 (addr. 17)"
                }
                frame True {
                  w1668 = "17"
                  # "we are measuring 1st channel\non Keithley 2182 (addr. 17)"
                  n948 = GPIB Write(0:w1668, 1:":SENSe:DATA:FRES?") -> (6:w1669:errorcluster)  [unwired: 3 in, 1 out]
                  n949 = GPIB Read(0:w1668, 1:200, 3:w1669) -> (5:w1664:string)  [unwired: 2 in, 2 out]
                  n950 = Fract/Exp String To Number(string=w1664) -> (number=w1666:dbl)  [unwired: 3 in, 1 out]
                  n951 = Build Array (concatenate)(w1671, w1666) -> (w1670:dbl[])
                }
              }
              n952 = property on="array for data" class="Arr (strict)"("Value"=w1661) -> ()  [unwired: 2 in, 2 out]
            }
            frame #22 {
              # "check if 2nd channel\non Keithley 2182 \n(addr. 17) is to\nbe measured"
              n953 = property on="Channel 2 (Vnano3b)" class="Bool (strict)"() -> ("Value"=w1672:bool)  [unwired: 2 in, 2 out]
              n954 = property on="array for data" class="Arr (strict)"() -> ("Value"=w1674:dbl[])  [unwired: 2 in, 2 out]
              n955 = case shown="False" w1672 {
                tunnel: w1674 -> [w1675 w1687]
                tunnel: [w1675 w1686] -> w1673
                frame False {
                  # "we are not measuring 1st channel\non Keithley 2182 (addr. 17)"
                }
                frame True {
                  w1678 = "17"
                  # "switching to channel 2 and then\nback to channel 1"
                  # "we are measuring 2nd channel\non Keithley 2182 (addr. 17)"
                  n956 = GPIB Write(0:w1678, 1:":SENSe:CHAN 2") -> (6:w1679:errorcluster)  [unwired: 3 in, 1 out]
                  n957 = GPIB Write(0:w1678, 1:":SENSe:DATA:FRES?", 3:w1679) -> (6:w1685:errorcluster)  [unwired: 2 in, 1 out]
                  n958 = GPIB Read(0:w1678, 1:200, 3:w1685) -> (5:w1681:string, 7:w1677:errorcluster)  [unwired: 2 in, 1 out]
                  n959 = GPIB Write(0:w1678, 1:":SENSe:CHAN 1", 3:w1677) -> ()  [unwired: 2 in, 2 out]
                  n960 = Fract/Exp String To Number(string=w1681) -> (number=w1683:dbl)  [unwired: 3 in, 1 out]
                  n961 = Build Array (concatenate)(w1687, w1683) -> (w1686:dbl[])
                }
              }
              n962 = property on="array for data" class="Arr (strict)"("Value"=w1673) -> ()  [unwired: 2 in, 2 out]
            }
            frame #23 {
              # "check if 1st \nthermometer on \nOxford ITC \n(address 24) \nis measured"
              n963 = property on="Thermometer 1 (T1)" class="Bool (strict)"() -> ("Value"=w1688:bool)  [unwired: 2 in, 2 out]
              n964 = property on="array for data" class="Arr (strict)"() -> ("Value"=w1690:dbl[])  [unwired: 2 in, 2 out]
              n965 = case shown="True" w1688 {
                tunnel: w1690 -> [w1691 w1700]
                tunnel: [w1691 w1699] -> w1689
                frame False {
                  # "we are not measuring temperature on\nthermometer 1 (addr. 24)"
                }
                frame True {
                  w1692 = 1
                  w1697 = "24"
                  # "we are measuring temperature,\nthermometer 1 (addr. 24)"
                  n966 = GPIB Write(0:w1697, 1:"R 1", 2:w1692) -> (6:w1698:errorcluster)  [unwired: 2 in, 1 out]
                  n967 = GPIB Read(0:w1697, 1:200, 2:w1692, 3:w1698) -> (5:w1693:string)  [unwired: 1 in, 2 out]
                  n968 = Fract/Exp String To Number(string=w1693, offset=w1692) -> (number=w1695:dbl)  [unwired: 2 in, 1 out]
                  n969 = Build Array (concatenate)(w1700, w1695) -> (w1699:dbl[])
                }
              }
              n970 = property on="array for data" class="Arr (strict)"("Value"=w1689) -> ()  [unwired: 2 in, 2 out]
            }
            frame #24 {
              # "check if 1st \nthermometer on \nOxford ITC \n(address 24) \nis measured"
              n971 = property on="Magnetic Field (B)" class="Bool (strict)"() -> ("Value"=w1701:bool)  [unwired: 2 in, 2 out]
              n972 = property on="array for data" class="Arr (strict)"() -> ("Value"=w1703:dbl[])  [unwired: 2 in, 2 out]
              n973 = case shown="True" w1701 {
                tunnel: w1703 -> [w1704 w1713]
                tunnel: [w1704 w1712] -> w1702
                frame False {
                  # "we are not measuringmagnetic field (addr. 25)"
                }
                frame True {
                  w1705 = 1
                  w1710 = "25"
                  # "we are measuring magnetic field  (addr. 25)"
                  n974 = GPIB Write(0:w1710, 1:"R 7", 2:w1705) -> (6:w1711:errorcluster)  [unwired: 2 in, 1 out]
                  n975 = GPIB Read(0:w1710, 1:200, 2:w1705, 3:w1711) -> (5:w1706:string)  [unwired: 1 in, 2 out]
                  n976 = Fract/Exp String To Number(string=w1706, offset=w1705) -> (number=w1708:dbl)  [unwired: 2 in, 1 out]
                  n977 = Build Array (concatenate)(w1713, w1708) -> (w1712:dbl[])
                }
              }
              n978 = property on="array for data" class="Arr (strict)"("Value"=w1702) -> ()  [unwired: 2 in, 2 out]
            }
            frame #25 {
              # "check if capacitance\nand loss (address 28)\nare measured"
              n979 = property on="Capacitance (C) and Loss (L)" class="Bool (strict)"() -> ("Value"=w1714:bool)  [unwired: 2 in, 2 out]
              n980 = property on="array for data" class="Arr (strict)"() -> ("Value"=w1716:dbl[])  [unwired: 2 in, 2 out]
              n981 = case shown="True" w1714 {
                tunnel: w1716 -> [w1717 w1723]
                tunnel: [w1717 w1719] -> w1715
                frame False {
                  # "we are not measuringmagnetic capacitance (addr. 28)"
                }
                frame True {
                  # "we are measuring capacitance and loss  (addr. 28)"
                  n982 = stacked-sequence {
                    seq-local: [w1725 _ _] -> [_ _ w1748]
                    tunnel: [_ _ w1742] -> w1718
                    tunnel: [_ _ w1743] -> w1721
                    tunnel: "28" ("data") -> [w1724 w1728 w1737]
                    frame #0 {
                      n983 = GPIB Write(0:w1724, 1:"SINGLE" ("data"), 2:i16 0 ("mode (0)")) -> (6:w1725:errorcluster)  [unwired: 2 in, 1 out]
                    }
                    frame #1 {
                      n984 = while {
                        tunnel: w1728 -> [w1729]
                        i -> [w1730]
                        stop <- w1732 continue-if-true
                        n985 = GPIB Serial Poll(0:w1729) -> (2:w1734:i16)  [unwired: 1 in, 2 out]
                        n986 = Less?(x=w1734, y=i16 128) -> (x < y?=w1732:bool)
                        n987 = Wait (ms)(milliseconds to wait=u32 50) -> ()  [unwired: 1 out]
                        "Numeric 3" <- w1730
                      }
                    }
                    frame #2 {
                      w1735 = i16 2 ("mode (0)")
                      n988 = GPIB Read(0:w1737, 1:200 ("byte count"), 2:i16 2 ("mode (0)"), 3:w1748) -> (5:w1741:string)  [unwired: 1 in, 2 out]
                      n989 = Match Pattern(string=w1741, regular expression="C=") -> (after substring=w1740:string)  [unwired: 1 in, 3 out]
                      n990 = Match Pattern(string=w1740, regular expression="PF L=") -> (after substring=w1738:string)  [unwired: 1 in, 3 out]
                      n991 = Search/Split String(string=w1740, search string/char (-)=" ", offset (0)=w1735) -> (substring before match=w1745:string)  [unwired: 2 out]
                      n992 = Search/Split String(string=w1738, search string/char (-)=" ", offset (0)=w1735) -> (substring before match=w1744:string)  [unwired: 2 out]
                      n993 = Fract/Exp String To Number(string=w1744) -> (number=w1742:dbl)  [unwired: 3 in, 1 out]
                      n994 = Fract/Exp String To Number(string=w1745) -> (number=w1743:dbl)  [unwired: 3 in, 1 out]
                    }
                  }
                  n995 = Build Array (concatenate)(w1723, w1721) -> (w1720:dbl[])
                  n996 = Build Array (concatenate)(w1720, w1718) -> (w1719:dbl[])
                }
              }
              n997 = property on="array for data" class="Arr (strict)"("Value"=w1715) -> ()  [unwired: 2 in, 2 out]
            }
          }
        }
      }
      n998 = property on="Sweep Rate" class="DigNum (strict)"() -> ("Value"=w538:dbl)  [unwired: 2 in, 2 out]
      n999 = property on="array for data" class="Arr (strict)"(error in=w575) -> ("Value"=w560:dbl[])  [unwired: 1 in, 2 out]
      n1000 = property on="Current B-Field" class="DigNum (strict)"() -> ("Value"=w534:dbl)  [unwired: 2 in, 2 out]
      n1001 = property on="Target B-Field" class="DigNum (strict)"() -> ("Value"=w540:dbl)  [unwired: 2 in, 2 out]
      n1002 = while {
        shift-right: [w1762] -> w556
        shift-left: w560 -> [w1764]
        i -> [w1763]
        stop <- w1767 stop-if-true
        # "loop goes through the list of all measured parameters\nif some columns are identified as current or resistance\nthey are recalculated according to selected or entered parameters"
        n1003 = Increment(x=w1763) -> (x+1=w1768:i32)
        n1004 = property on="Ring" class="Ring (strict)"() -> ("Strings []"=w1766:string[])  [unwired: 2 in, 2 out]
        n1005 = Index Array(array=w1766, index=w1763) -> (element=w1765:string)
        n1006 = property on="Ring" class="Ring (strict)"() -> ("NumItems"=w1769:u32)  [unwired: 2 in, 2 out]
        n1007 = case shown="\"False\", Default" w1765 {
          tunnel: w1764 -> [w1775 w1785 w1795 w1802]
          tunnel: w1763 -> [w1773 w1782 w1793 _]
          tunnel: [w1774 w1783 w1794 w1802] -> w1762
          frame "I" {
            n1008 = property on="Current is:" class="RadioBtnsControl (strict)"() -> ("Value"=w1771:T1)  [unwired: 2 in, 2 out]
            n1009 = case shown="\"Radio Selection 2\"" w1771 {
              tunnel: ["Ring 3" "Ring 2"] -> w1770
              frame "Radio Selection 3", Default {
              }
              frame "Radio Selection 2" {
              }
            }
            n1010 = Index Array(array=w1775, index=w1773) -> (element=w1776:dbl)
            n1011 = Power Of 10(x=w1770) -> (10^x=w1779:dbl)
            n1012 = Multiply(x=1000.0, y=w1779) -> (x*y=w1777:dbl)
            n1013 = Divide(x=w1776, y=w1777) -> (x/y=w1772:dbl)
            "Numeric Current" <- w1772
            n1014 = Replace Array Subset(array=w1775, new element=w1772, index=w1773) -> (w1774:dbl[])
          }
          frame "Ioop" {
            n1015 = property on="Ring 3" class="Ring (strict)"() -> ("Value"=w1784:u16)  [unwired: 2 in, 2 out]
            n1016 = Index Array(array=w1785, index=w1782) -> (element=w1787:dbl)
            n1017 = Power Of 10(x=w1784) -> (10^x=w1790:dbl)
            n1018 = Multiply(x=1000.0, y=w1790) -> (x*y=w1788:dbl)
            n1019 = Divide(x=w1787, y=w1788) -> (x/y=w1786:dbl)
            n1020 = Replace Array Subset(array=w1785, new element=w1786, index=w1782) -> (w1783:dbl[])
          }
          frame "R1", "R1oop", "R2", "R2oop", "R3", "R3oop", "R4", "R4oop", "R5", "R5oop" {
            n1021 = property on="Current is:" class="RadioBtnsControl (strict)"() -> ("Value"=w1792:T1)  [unwired: 2 in, 2 out]
            n1022 = case shown="\"Radio Selection 2\", Default" w1792 {
              tunnel: [w1798 w1801] -> w1791
              frame "Radio Selection 1" {
                n1023 = Divide(x="Fixed Current mkA", y=1000000.0) -> (x/y=w1798:dbl)
              }
              frame "Radio Selection 2", Default {
                n1024 = property on="Numeric Current" class="DigNum (strict)"() -> ("Value"=w1801:dbl)  [unwired: 2 in, 2 out]
              }
            }
            n1025 = Index Array(array=w1795, index=w1793) -> (element=w1797:dbl)
            n1026 = Divide(x=w1797, y=w1791) -> (x/y=w1796:dbl)
            n1027 = Replace Array Subset(array=w1795, new element=w1796, index=w1793) -> (w1794:dbl[])
          }
          frame "False", Default {
          }
        }
        n1028 = Less?(x=w1769, y=w1768) -> (x < y?=w1767:bool)
      }
      n1029 = Subtract(x=w540, y=w534) -> (x-y=w542:dbl)
      "Difference" <- w542
      n1030 = Sign(1:w542) -> (0:w543:dbl)
      n1031 = Multiply(x=w543, y=w542) -> (x*y=w539:dbl)
      n1032 = Divide(x=w539, y=w538) -> (x/y=w535:dbl)
      "Time of measurement Measurement" <- w535
      n1033 = Divide(x=w535, y="Time btw \npoints, sec") -> (x/y=w536:dbl)
      n1034 = Divide(x=w539, y=w536) -> (x/y=w541:dbl)
      n1035 = Sign(1:w542) -> (0:w561:dbl)
      n1036 = Multiply(x=w561, y=w541) -> (x*y=w554:dbl)
      n1037 = property on="points at each Vg" class="DigNum (strict)"() -> ("Value"=w553:i32)  [unwired: 2 in, 2 out]
      n1038 = To Double Precision Float(number=w553) -> (double precision float=w552:dbl)
      n1039 = Multiply(x=w552, y=w554) -> (x*y=w551:dbl)
      n1040 = property on="Commutator" class="Bool (strict)"() -> ("Value"=w545:bool)  [unwired: 2 in, 2 out]
      n1041 = property on="Data file:" class="Path"() -> ("Value"=w558:path)  [unwired: 2 in, 2 out]
      n1042 = Divide(x=w542, y=w551) -> (x/y=w573:dbl)
      n1043 = case shown="False" w545 {
        tunnel: w562 -> [w589 w600]
        tunnel: w547 -> [w584 w594]
        tunnel: [w576 w593] -> w544
        frame True {
          # "calculate deliberate time delay for the next step"
          n1044 = Subtract(x=w589, y=w584) -> (x-y=w582:u32)
          n1045 = property on="Delib Time delay" class="DigNum (strict)"() -> ("Value"=w583:i32)  [unwired: 2 in, 2 out]
          n1046 = property on="Time btw \npoints, sec" class="DigNum (strict)"() -> ("Value"=w588:dbl)  [unwired: 2 in, 2 out]
          n1047 = Subtract(x=w582, y=w583) -> (x-y=w581:u32)
          n1048 = Multiply(x=w588, y=1000.0) -> (x*y=w586:dbl)
          n1049 = To Long Integer(number=w586) -> (32bit integer=w585:i32)
          n1050 = Greater?(x=w585, y=w581) -> (0:w578:bool)
          n1051 = Subtract(x=w585, y=w581) -> (x-y=w580:u32)
          n1052 = Divide(x=w580, y=2) -> (x/y=w577:dbl)
          n1053 = case shown="False" w578 {
            tunnel: w577 -> [_ w592]
            tunnel: [0 w591] -> w576
            frame False {
            }
            frame True {
              n1054 = To Long Integer(number=w592) -> (32bit integer=w591:i32)
            }
          }
        }
        frame False {
          # "calculate deliberate time delay for the next step"
          n1055 = Subtract(x=w600, y=w594) -> (x-y=w597:u32)
          n1056 = property on="Time btw \npoints, sec" class="DigNum (strict)"() -> ("Value"=w599:dbl)  [unwired: 2 in, 2 out]
          n1057 = Multiply(x=w599, y=1000.0) -> (x*y=w596:dbl)
          n1058 = To Long Integer(number=w596) -> (32bit integer=w595:i32)
          n1059 = Greater?(x=w595, y=w597) -> ()  [unwired: 1 out]
          n1060 = Subtract(x=w595, y=w597) -> (x-y=w593:u32)
        }
      }
      "Delib Time delay" <- w544
      n1061 = Decrement(x=w573) -> (x-1=w572:dbl)
      n1062 = Absolute Value(x=w542) -> (abs(x)=w569:dbl)
      n1063 = Build Array (concatenate)(w574, w556) -> (w555:dbl[][])
      n1064 = Greater Than 0?(x=w572) -> (x > 0?=w571:bool)
      n1065 = property on="array for data" class="Arr (strict)"("Value"=w556) -> ()  [unwired: 2 in, 2 out]
      n1066 = call-poly <vilib>:"Write To Spreadsheet File.vi"("format (%.3f)"="%#g", "append to file? (new file:F)"=TRUE, "1D data"=w556, "file path (dialog if empty)"=w558) -> ()  [unwired: 4 in, 1 out]
      n1067 = Less?(x=w569, y=1e-06) -> (x < y?=w567:bool)
      n1068 = flat-sequence {
        tunnel: [w1761] -> w562
        tunnel: w555 -> [w1755]
        frame #0 {
          # "time is mesured at the end of the cycle\nto adjust a delay time"
          # "this part plots selected measurements"
          n1069 = Tick Count (ms)() -> (millisecond timer value=w1761:u32)
          n1070 = Index Array(array=w1755, index (col)="Ring") -> (element=w1760:dbl[])  [unwired: 1 in]
          n1071 = Index Array(array=w1755, index (col)=0) -> (element=w1758:dbl[])  [unwired: 1 in]
          n1072 = Bundle(w1758, w1760) -> (→"XY Graph":cluster{dbl[], dbl[]})  [unwired: 1 in]
        }
      }
      n1073 = case shown="True" w571 {
        tunnel: w565 -> [_ w1806]
        tunnel: w551 -> [_ w1805]
        tunnel: [w1803 w1804] -> w570
        frame False {
          # "if next step is too long\nuse target voltage"
          n1074 = property on="Target B-Field" class="DigNum (strict)"() -> ("Value"=w1803:dbl)  [unwired: 2 in, 2 out]
        }
        frame True {
          # "add increment to\nthe current B"
          n1075 = Add(x=w1805, y=w1806) -> (x+y=w1804:dbl)
        }
      }
    }
    n1076 = Number To Fractional String(number=w514) -> (F-format string=w518:string)  [unwired: 3 in]
    n1077 = Concatenate Strings("$J " ("data"), w518) -> (w517:string)
    n1078 = Equal?(x=w512, y="optional Bias (V)") -> (x = y?=w515:bool)
    n1079 = case shown="False" w515 {
      tunnel: "optional Bias (V)" -> [w525 _]
      tunnel: w514 -> [w526 _]
      frame False {
        n1080 = Multiply(x=w526, y=22.62) -> (x*y=w527:dbl)
        n1081 = Number To Fractional String(number=w525) -> (F-format string=w533:string)  [unwired: 3 in]
        n1082 = Add(x=w525, y=w527) -> ()  [unwired: 1 out]
        n1083 = Concatenate Strings(":INIT:IMM; :SOUR:VOLT:LEV:IMM:AMPL " ("data"), w533) -> (w532:string)
        n1084 = property on="optional Bias (V)" class="DigNum (strict)"("Visible"=TRUE) -> ()  [unwired: 2 in, 2 out]
        n1085 = GPIB Write(0:"13", 1:w532) -> ()  [unwired: 3 in, 2 out]
      }
      frame True {
      }
    }
    n1086 = GPIB Write(0:"25" ("address string"), 1:w517, 2:i16 1 ("mode (0)")) -> ()  [unwired: 2 in, 2 out]
  }
  "Array 2" <- w13
  n1087 = Write to Text File(file (use dialog)=w16, text=w15) -> ()  [unwired: 2 in, 3 out]
  n1088 = Array Size(array=w6) -> (size(s)=→"Numeric 2":i32)
  n1089 = property on="optional Bias (V)" class="DigNum (strict)"("Value"=w11, "Visible"=FALSE) -> ()  [unwired: 2 in, 2 out]
